vi "ControlProgram5.5.vi"() -> ()   [LabVIEW 2016]
uses:
  <vilib>/Utility/error.llb/DialogType.ctl
  <vilib>/Utility/miscctls.llb/LVPoint32TypeDef.ctl
  <vilib>/DAQmx/write.llb/DAQmx Write (Digital Bool 1Line 1Point).vi
  <vilib>/DAQmx/create/channels.llb/DAQmx Create Channel (DO-Digital Output).vi
  <vilib>/platform/TimedLoop/XDataNode/XDataNode.xnode
  <vilib>/Platform/TimedLoop/XDataNode/nitl_modes.ctl
  <vilib>/Platform/TimedLoop/XDataNode/XDNodeRunTimeDep.lvlib
  <vilib>/Platform/TimedLoop/XDataNode/wakeup.ctl
  <vilib>/Platform/TimedLoop/XDataNode/timing_clust.ctl
  <vilib>/DAQmx/create/channels.llb/DAQmx Create Channel (AI-Voltage-Basic).vi
  <vilib>/DAQmx/create/channels.llb/DAQmx Create Channel (AO-Voltage-Basic).vi
  <vilib>/DAQmx/write.llb/DAQmx Write (Analog 1D DBL NChan 1Samp).vi
  <resource>/objmgr/daqmx.rc
  <vilib>/Analysis/NI_AALBase.lvlib
  <vilib>/Analysis/baseanly.llb/Mean (DBL).vi
  <vilib>/Instr/_visa.llb/VISA Configure Serial Port (Instr).vi
  <vilib>/Utility/inputDevices.llb/closeMouse.vi
  <vilib>/Utility/inputDevices.llb/mouseAcquire.vi
  <vilib>/DAQmx/read.llb/DAQmx Read (Analog 2D DBL NChan NSamp).vi
  <vilib>/DAQmx/configure/timing.llb/DAQmx Timing (Sample Clock).vi
panel:
  in  "Save file index":i32
  out "Flush Sample Start Time":u32=2111292881
  out "Sample flush time (s)":dbl=48.0
  in  "Inject Sample":bool
  out "Chart Freq (Hz)":dbl=500.0
  out "Cal values":T1={"AX alpha"=612.9626061060078, "BX alpha"=549.6584469744151, "AX kappa"=0.3485731373010688, "BX kappa"=0.3853424216291352, "AX offset"=-0.03900484438240665, "BX offset"=-0.11295550662085417, "AY alpha"=582.7562541114835, "BY alpha"=571.1587543790358, "AY kappa"=0.37498408087930674, "BY kappa"=0.36252029651198364, "AY offset"=-0.21125584642206058, "BY offset"=-0.12469077200400738}
  in  "Inject Pump 1":bool
  in  "Inject Pump 2":bool
  in  "Tab Control 2":T2(tab)
  in  "Force FB script":bool
  in  "Got ADig bead":bool
  in  "Move Cap. 2 (ADig Top)":bool
  in  "Dump beads":bool
  in  "Got DNA bead":bool
  in  "Flow on\ncap 2?":bool=TRUE
  in  "Flow on\ncap 1?":bool=TRUE
  in  "Flow on\ndump?":bool=TRUE
  in  "Fish After TA?":bool=TRUE
  in  "Delta after tether":dbl=1600.0
  in  "TA Cancel Save?":bool=TRUE
  in  "Min fish\ndelta (nm)":dbl=1425.0 min=0.0 max=5000.0 step=50.0
  in  "Max fish\ndelta (nm)":dbl=1900.0 min=0.0 max=5000.0 step=25.0
  in  "Fish Speed (ms)":i32=5000
  in  "Wait (ms)":i32=1500
  in  "# attempts":dbl=10.0
  in  "Cutoff force (pN)":dbl=4.5
  in  "Raster after\n tether?":bool=TRUE
  out "Tether":bool
  out "Attempt #":i32
  in  "Flow on\nwhile fish?":bool=TRUE
  in  "Flow on\nafter raster?":bool=TRUE
  in  "Offset @ Delta (nm)":dbl=1600.0
  in  "Cal @ Delta (nm)":dbl=2500.0
  in  "Cal stage position":i32=3
  out "Cal Final Sampling Rate":dbl=125000.0
  in  "Cal Averaging":i32=1
  in  "Wait before dip (s)":dbl=3.0
  in  "Start dipping after?":bool
  in  "Start trap delta (nm)":dbl=1700.0
  in  "Cancel dwell":bool
  in  "Pause dwell":bool
  in  "Return position":dbl=3.0
  in  "Dip duration":dbl=15.0
  in  "Dip position":dbl=4.0
  in  "Dip":bool
  out "Dip time":i32
  in  "Stop":bool=TRUE
  in  "?":T3(tab)=enum."Raster scan"
  in  "Save N sets":bool
  in  "N sets":i32=200
  in  "Cal sets to save":i32=500
  in  "Reset data stream":bool
  out "Buffer Overflow":bool
  out "Stage moving":bool
  in  "Comment":string
  in  "Raster scan":bool
  out "Saving":bool
  in  "Save cal":bool
  in  "Save Data":bool
  in  "Stop saving":bool
  out "Calibrating":bool
  out "Progress":dbl(slide) scale=0.0..100.0
  in  "Read Cal":bool
  in  "Fish":bool
  in  "Averaging Number":i32=1250
  out "Final Sampling Rate":dbl=100.0
  in  "Trap position (V)":cluster{"X":dbl, "Y":dbl}={"X"=4.184262478968032, "Y"=2.3}
  in  "Trap delta (nm)":dbl=2500.0 min=0.0 max=5000.0 step=50.0
  in  "Fixed X":dbl=1.38
  in  "Fixed Y":dbl=2.3
  in  "Shutter 1 (B)":bool=TRUE
  in  "Shutter 2 (A)":bool
  in  "Pulling direction":bool
  out "Raster scanning...":bool
  out "Current file name":path=path "D:/data/160111/160111_006.dat"
  in  "AX alpha":dbl=612.9626061060078 format="%#_3p"
  in  "BX alpha":dbl=549.6584469744151 format="%#_3g"
  in  "AX kappa":dbl=0.3485731373010688 format="%#_3g"
  in  "BX kappa":dbl=0.3853424216291352 format="%#_3g"
  in  "AX offset":dbl=-0.03900484438240665 format="%#_3g"
  in  "BX offset":dbl=-0.11295550662085417 format="%#_3g"
  in  "AY alpha":dbl=582.7562541114835 format="%#_3g"
  in  "BY alpha":dbl=571.1587543790358 format="%#_3g"
  in  "AY kappa":dbl=0.37498408087930674 format="%#_3g"
  in  "BY kappa":dbl=0.36252029651198364 format="%#_3g"
  in  "AY offset":dbl=-0.21125584642206058 format="%#_3g"
  in  "BY offset":dbl=-0.12469077200400738 format="%#_3g"
  out "Buffer status":u8(slide) scale=0.0..100.0
  in  "Set Current\nPos to (0,0,0)":bool
  in  "dump spot":string="Dump beads spot"
  in  "up flow spot":string="Upper flow spot"
  in  "low flow spot":string="Lower flow spot"
  in  "up cap":string="Upper capillary (ADig beads)"
  in  "bottom cap":string="Lower capillary (DNA beads)"
  in  "Move to Position 5":bool
  in  "Set Position 5":bool
  in  "Saved stage positions":dbl[][](array[numeric])=[[1.0, 0.0, 0.0, 0.0], [2.0, -0.13716, -3.21132, 0.01436], [3.0, 0.45, -0.73974, 0.005], [4.0, 0.45, -2.1978, 0.005], [5.0, 0.45, -2.63158, -0.02256]]
  in  "Set Position 2":bool
  in  "Move to Position 2":bool
  in  "Set Position 1":bool
  in  "Move to Position 1":bool
  in  "Set Position 4":bool
  in  "Move to Position 4":bool
  in  "Set Position 3":bool
  in  "Move to Position 3":bool
  out "Stage error":errorcluster
  in  "Clear Volume":bool
  out "Sample Flush Meter":u8(slide) scale=0.0..100.0
  out "Flushing Sample":bool
  in  "Flush Sample":bool
  in  "Normal \nRate (ul/hr)  3":dbl=100.0
  in  "Normal \nVolume (ul) 3":dbl=250.0
  in  "Normal \nVolume (ul) 2":dbl
  in  "Normal \nRate (ul/hr)":dbl
  in  "Normal \nVolume (ul)":dbl
  in  "Flush\nRate (ul/min)":dbl
  in  "Flush\nVolume (ul)":dbl
  in  "Flush \nRate (ul/min)  2":dbl
  in  "Flush Pump 2":bool
  in  "Flush\nVolume (ul)  2":dbl
  in  "Flush Pump 1":bool
  in  "Normal \nRate (ul/hr)  2":dbl
  in  "Write Wait":i32=1000
  in  "Flush \nRate (ul/min)  3":dbl=100.0
  in  "Flush\nVolume (ul)  3":dbl=80.0
  out "error out":errorcluster
  in  "Use Mouse to Move Trap?":bool
  in  "Pause Mouse/Mirror Connection":bool
  out "Reference Voltage":cluster{dbl, dbl}={0.0, -0.0}
  out "Saved voltage":cluster{dbl, dbl}={5.766666666666665, 1.45}
  out "Real Coordinates":cluster{"Horizontal":i32, "Vertical":i32}={"Horizontal"=897, "Vertical"=-1271}
  out "CoordinatesMousePressed":T4
  out "Sum error":dbl(knob) scale=-0.1..0.1
  out "Trap sep":waveform(dbl)[](graph)=[{"t0"=timestamp(254.52999999991349 s since 1904-01-01), "dt"=0.002, "Y"=[2500.401353709495, 2500.7138927997967, 2500.64380131258, 2500.593243518474, 2500.684017739553], "attributes"=variant("NI_ChannelName"=variant(string "T2 X"))}, {"t0"=timestamp(254.52999999991349 s since 1904-01-01), "dt"=0.002, "Y"=[2.3273345839872768, 2.356012897788485, 2.38273587208189, 2.3403701811713593, 2.3442808603313674], "attributes"=variant("NI_ChannelName"=variant(string "T2 Y"))}]
  in  "Set reading to\nsetpoint":bool
  in  "Offset Y (nm)":dbl format="%0.2f"
  in  "Offset X (nm)":dbl format="%0.2f"
  in  "Remove offsets":bool
  in  "Force Feedback":bool
  out "Feedback Output Voltage 2":cluster{dbl, dbl} {"?" format="%#_4g"; "?" format="%#_4g"}
  in  "Offset":cluster{"Off Y":dbl, "Off X":dbl}={"Off Y"=1.5, "Off X"=0.17}
  in  "Setpoint voltage":cluster{"SP Y":dbl, "SP X":dbl}={"SP Y"=0.6, "SP X"=0.0}
  in  "Feedback const":T5={"Ki_B_Y"=0.5, "Ki_B_X"=0.0, "Kp Y"=1.0, "Kp X"=0.0}
  out "Mean Trap Pos X 2 (nm)":dbl=2500.6072618159797 format="%0.2f"
  out "Mean Trp Pos Y 2 (nm)":dbl=2.3501468790720756 format="%0.2f"
  out "T2 X RMS (A)":dbl=1.1062679088370557 format="%0.2f"
  out "T2 Y RMS (A)":dbl=0.1869142822643123 format="%0.2f"
  in  "Scan range (nm)":dbl=425.0
  in  "Scan speed (nm/s)":dbl=100.0 min=0.0 max=100.0
  in  "Step size (nm)":dbl=1.0
  in  "Save scans":bool=TRUE
  in  "# scans":i32=1
  in  "Load param":bool
  in  "Scan Parameters":T6(array[cluster])=[{"Label"="Offset", "Max delta 2"=3.8, "Start delta 2"=2.4, "Speed (ms) 2"=10000, "# scans 2"=1}]
  in  "Trap delta\nafter (nm)":dbl=1750.0
  in  "Stop raster":bool
  out "Scan range (V)":dbl=0.47672462142456534
  out "Scan steps (mirror)":u64=425
  out "Scan increment (V)":dbl=0.0011217049915872126
  out "Time per step (ms)":dbl=10.0
  out "Total raster time (s)":dbl=8.5
  out "N sets to be saved":dbl=850.0
  out "Continue to display?":bool
  out "Video Error":errorcluster
  in  "# Samples/channel (in)":i32=40000 format="%.2f"
  out "Buffer size\n(Samples/channel)":u32=511
  out "DAQ rate\n(Samples/s)":dbl=125000.0 format="%#_6p"
  out "# Samples/channel":i32=1250
  out "# Samples/channel/s":dbl=100.0
  out "AvailSampPerChan":u32=9
  out "Data update period (s/set)":dbl=0.01 format="%#_6p"
  out "AvailSampPerChan 2":u32=110
  in  "PC samp per channel":i32=1000
  in  "Sampling Rate":dbl=125000.0 format="%0.0p"
  in  "DAQ Rate2":dbl=1000000.0 format="%#_6p"
  out "Data period (s)":dbl=8e-06 format="%#_6p"
  in  "Tether break\nforce (pN)":dbl=1.0
  in  "Path":path=path "D:/data"
  out "Mirror task":refnum<k21>
  in  "Conv X (nm/V)":dbl=891.5
  in  "Conv Y (nm/V)":dbl=505.7
  in  "Min value Y":dbl format="%.1g"
  in  "Max value Y":dbl=10.0 format="%.1f"
  in  "Min value X":dbl format="%0.1f"
  in  "Max value X":dbl=10.0 format="%.1f"
  in  "HWP1":string="Half waveplate 1: differential trap power"
  in  "HWP0":string="Half waveplate 0: total trap power"
  in  "Move 1":bool
  in  "\"Degrees\" 1":dbl
  in  "Move 0":bool
  in  "\"Degrees\" 0":dbl
  out "Chamber":T7(plugin-control)
  out "Deflection":T4
  in  "Sampling Rate":dbl=125000.0 format="%0.2f"
  in  "Averaging Number":i32=12500
  in  "DAQ Rate":dbl=1000000.0
  out "Final Sampling Rate":dbl
  in  "Tab Control":T8(tab)
  in  "Downsamp\nfact":dbl=250.0
  out "Bead sep":waveform(dbl)[](graph)=[{"t0"=timestamp(254.52999999991349 s since 1904-01-01), "dt"=0.002, "Y"=[213.39995113031458, 213.93706235351536, 212.9933488170291, 212.83435664066477, 214.2058422181686], "attributes"=variant("NI_ChannelName"=variant(string "T2"))}, {"t0"=timestamp(254.52999999991349 s since 1904-01-01), "dt"=0.002, "Y"=[5.143660273474187, 5.894059413878943, 4.88588887583271, 5.354302143675658, 5.8339035430258015], "attributes"=variant("NI_ChannelName"=variant(string "T1"))}]
  out "Force (pN)":waveform(dbl)[](graph)=[{"t0"=timestamp(254.52999999991349 s since 1904-01-01), "dt"=0.002, "Y"=[77.86854854855086, 78.08600694234892, 77.6994254352176, 77.66772581948469, 78.22322365982815], "attributes"=variant("NI_ChannelName"=variant(string "T2"))}, {"t0"=timestamp(254.52999999991349 s since 1904-01-01), "dt"=0.002, "Y"=[1.9758532189955713, 2.255599507656321, 1.8769321413323554, 2.045475885196074, 2.2199437572021146], "attributes"=variant("NI_ChannelName"=variant(string "T1"))}]
  out "Mean force (pN)":dbl=39.991873491581266 format="%0.2f"
  out "Force noise (pN)":dbl=0.17287401460430454 format="%0.2f"
  out "Mean Bead Sep\n(nm)":dbl=109.44823754095798 format="%0.2f"
  out "Bead Sep Noise\n(A)":dbl=4.382305822805036 format="%0.2f"
  out "PSD 2":cluster{dbl[], dbl[]}(graph)
  out "PSD 1":cluster{dbl[], dbl[]}(graph)
  out "PSD 1 Sum":dbl(slide) scale=0.0..10.0
  out "PSD 2 Sum":dbl(slide) scale=0.0..10.0
  in  "Start":bool
  out "All signals":waveform(dbl)[](graph)=[{"t0"=timestamp(254.52999999991349 s since 1904-01-01), "dt"=0.002, "Y"=[-0.015598133099047685, -0.01565794312346797, -0.015569001492569037, -0.015625202290861444, -0.015752814195447103], "attributes"=variant("NI_ChannelName"=variant(string "A y"))}, {"t0"=timestamp(254.52999999991349 s since 1904-01-01), "dt"=0.002, "Y"=[-0.008051314077172257, -0.008039455196512668, -0.008078641062942567, -0.008046931447407441, -0.00800258954569925], "attributes"=variant("NI_ChannelName"=variant(string "A x"))}, {"t0"=timestamp(254.52999999991349 s since 1904-01-01), "dt"=0.002, "Y"=[-0.8186799727186506, -0.828518168587136, -0.8182847428509795, -0.8289376238127658, -0.8367167087325929], "attributes"=variant("NI_ChannelName"=variant(string "B y"))}, {"t0"=timestamp(254.52999999991349 s since 1904-01-01), "dt"=0.002, "Y"=[-0.7880865286255396, -0.794686015346124, -0.785544853888779, -0.7877818022288781, -0.7909004423629264], "attributes"=variant("NI_ChannelName"=variant(string "B x"))}, {"t0"=timestamp(254.52999999991349 s since 1904-01-01), "dt"=0.002, "Y"=[0.031377424462748806, 0.03139546842223122, 0.03140835696460643, 0.03146506655133351, 0.031459911134330096], "attributes"=variant("NI_ChannelName"=variant(string "A sum"))}, {"t0"=timestamp(254.52999999991349 s since 1904-01-01), "dt"=0.002, "Y"=[6.456821009406946, 6.459892496810089, 6.459914408291232, 6.460361662568834, 6.464131742766271], "attributes"=variant("NI_ChannelName"=variant(string "B sum"))}, {"t0"=timestamp(254.52999999991349 s since 1904-01-01), "dt"=0.002, "Y"=[4.184712679427364, 4.185063256085021, 4.184984634113943, 4.18492792318393, 4.185029745080822], "attributes"=variant("NI_ChannelName"=variant(string "Trap x"))}, {"t0"=timestamp(254.52999999991349 s since 1904-01-01), "dt"=0.002, "Y"=[2.3046022040418968, 2.3046589141739933, 2.3047117577063116, 2.3046279813746713, 2.304635714574513], "attributes"=variant("NI_ChannelName"=variant(string "Trap y"))}]
  # "Bead Calibration"
  # "Y"
  # "X"
  # "Pump #1 Controls"
  # "Pump #2 Controls"
  # "Sample Pump Controls"
  # "Retract the pumps manually. Change it back to INFUSE when you're done. Suck it up, don't whine."
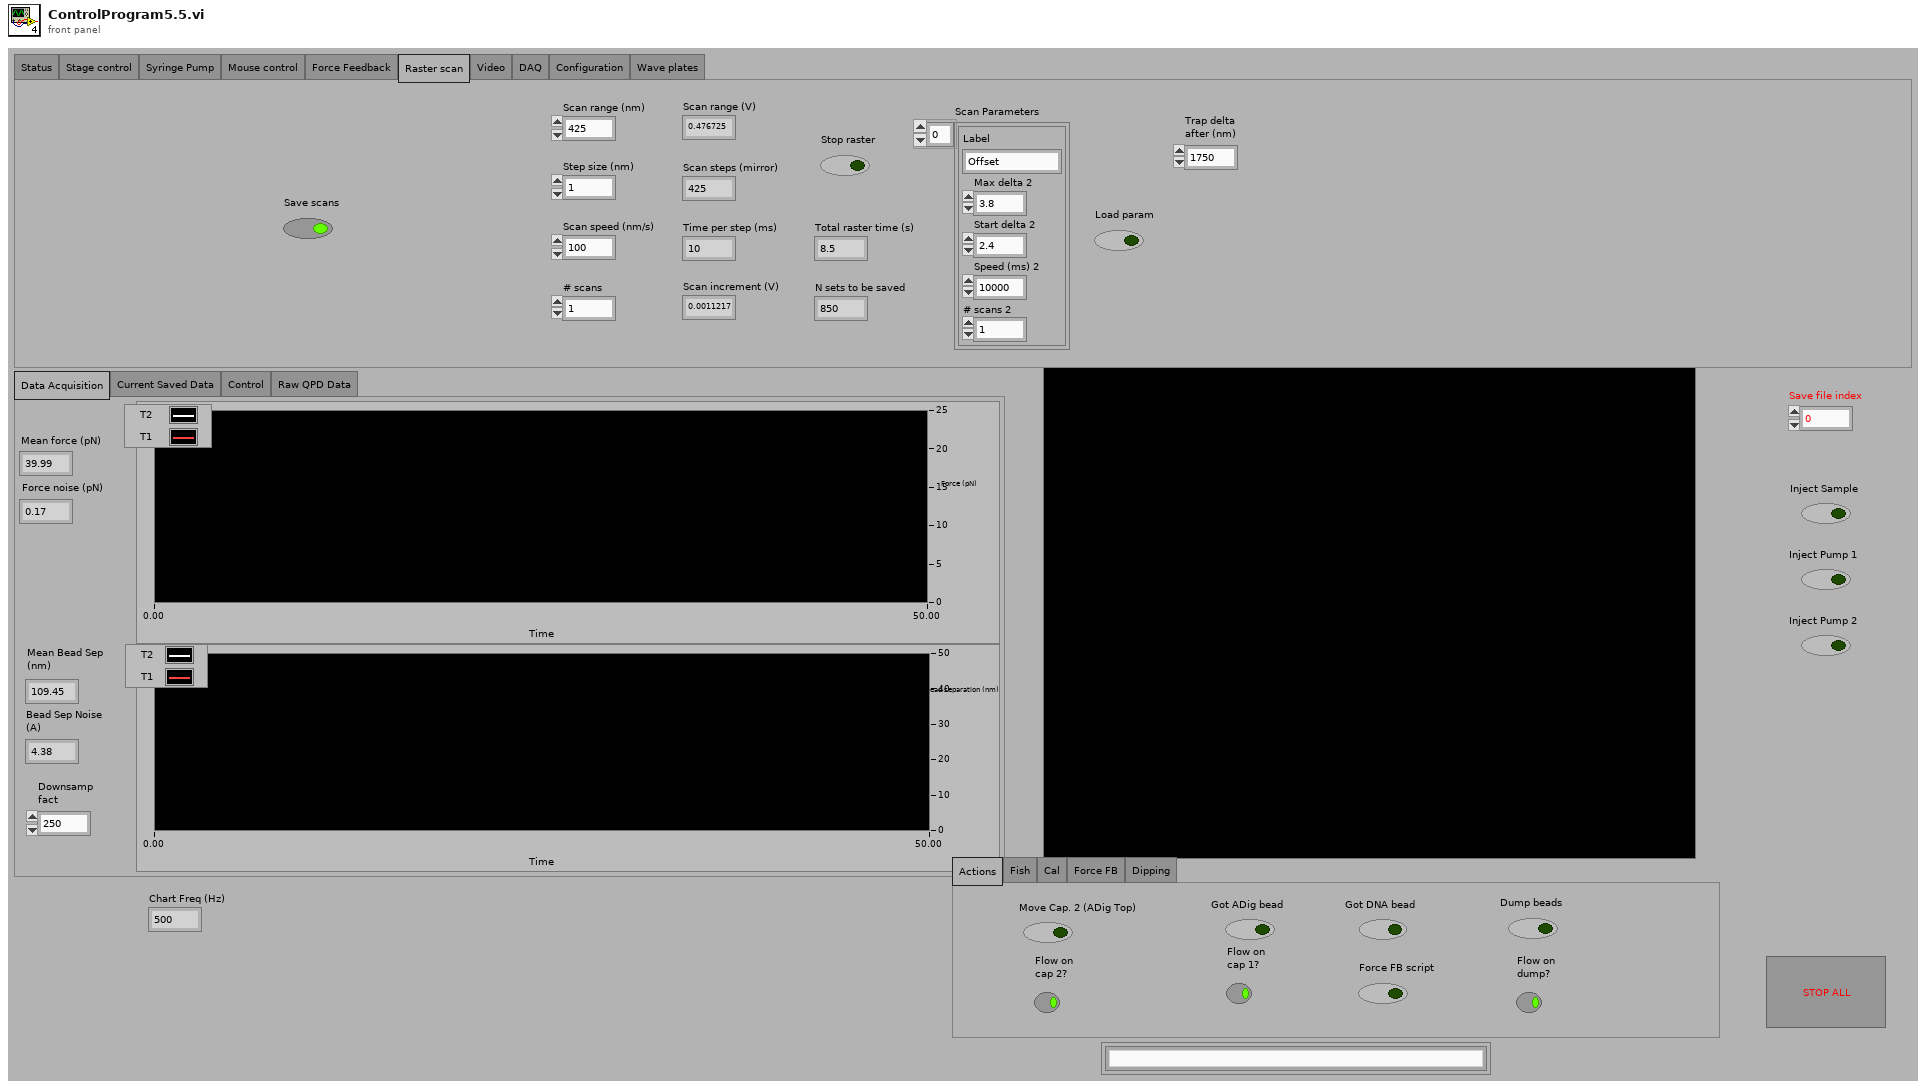
[diagram p1: front panel]
types:
  T1 = cluster{"AX alpha":dbl, "BX alpha":dbl, "AX kappa":dbl, "BX kappa":dbl, "AX offset":dbl, "BX offset":dbl, "AY alpha":dbl, "BY alpha":dbl, "AY kappa":dbl, "BY kappa":dbl, "AY offset":dbl, "BY offset":dbl}
  T2 = enum32{"Actions", "Fish", "Cal", "Force FB", "Dipping"}
  T3 = enum32{"Status", "Stage control", "Syringe Pump", "Mouse control", "Force Feedback", "Raster scan", "Video", "DAQ", "Configuration", "Wave plates"}
  T4 = typedef "LVPoint32TypeDef.ctl" = cluster{"Horizontal":i32, "Vertical":i32}
  T5 = cluster{"Ki_B_Y":dbl, "Ki_B_X":dbl, "Kp Y":dbl, "Kp X":dbl}
  T6 = cluster{"Label":string, "Max delta 2":dbl, "Start delta 2":dbl, "Speed (ms) 2":i32, "# scans 2":i32}[]
  T7 = typedef "IMAQ Image.ctl" = refnum<image>
  T8 = enum32{"Data Acquisition", "Current Saved Data", "Control", "Raw QPD Data"}
  T9 = enum16{"open", "replace", "create", "open or create", "replace or create", "replace or create with confirmation"}
  T10 = enum16{"big-endian, network order", "native, host order", "little-endian"}
  T11 = cluster{string, string, string, string, string, string, string, string}
  T12 = typedef "XDNodeRunTimeDep.lvlib/timing_clust.ctl" = cluster{"Expected End [f-1]":u64, "Actual End [f-1]":u64, "Finished Late? [f-1]":bool, "Expected End [i-1]":u64, "Actual End [i-1]":u64, "Finished Late? [i-1]":bool, "Expected Start [i]":u64, "Actual Start [i]":u64, "Expected Start [f]":u64, "Actual Start [f]":u64, "Source Name":string, "Structure Name":string, "Period":i64, "Deadline":i64, "Offset":i64, "Start":i64, "Priority":i32, "Timeout":i32, "Mode":T13, "Wakeup Reason":T14, "Error":errorcluster, "Source Type":string, "Secondary Source Type":string, "Global End Time":u64, "Global Start Time":u64, "Frame Duration":u64, "Iteration Duration":u64, "Assigned CPU":i32, "I/O Scan Engine Mode":u32}
  T13 = typedef "XDNodeRunTimeDep.lvlib/nitl_modes.ctl" = enum32{"No Change", "Process missed periods, maintain original phase", "Discard missed periods, maintain original phase", "Process missed periods, ignore original phase", "Discard missed periods, ignore original phase"}
  T14 = typedef "XDNodeRunTimeDep.lvlib/wakeup.ctl" = enum32{"Normal", "Aborted", "Asynchronous wakeup", "Timing source error", "Timed loop error", "Timeout"}
  T15 = typedef "DialogType.ctl" = u16
  T16 = cluster{"button 1":bool, "button 2":bool, "button 3":bool, "button 4":bool}
  T17 = cluster{"[0]":dbl, "[1]":dbl, "[2]":dbl, "[3]":dbl, "[4]":dbl, "[5]":dbl, "[6]":dbl, "[7]":dbl, "[8]":dbl, "[9]":dbl, "[10]":dbl, "[11]":dbl}
  T18 = cluster{"Label":string, "Max delta 2":dbl, "Start delta 2":dbl, "Speed (ms) 2":i32, "# scans 2":i32}
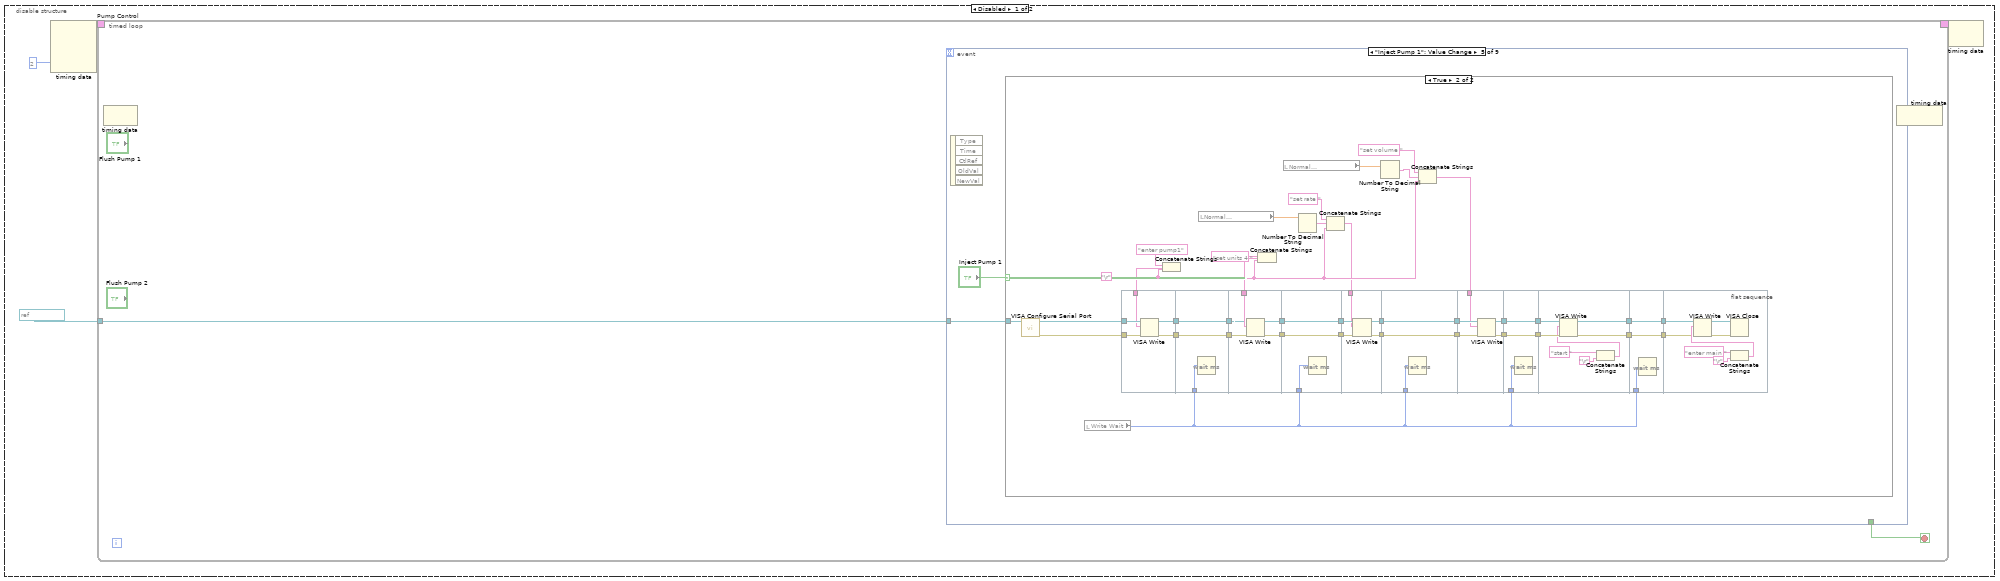
[diagram p2: hidden frame]
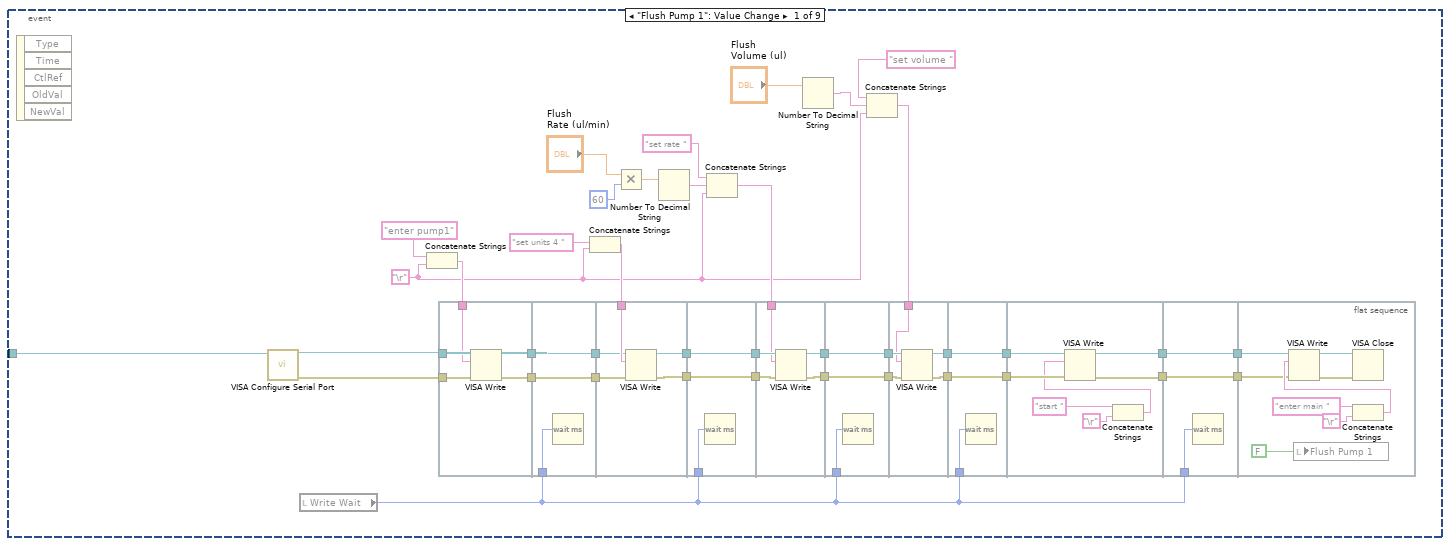
[diagram p3: hidden frame]
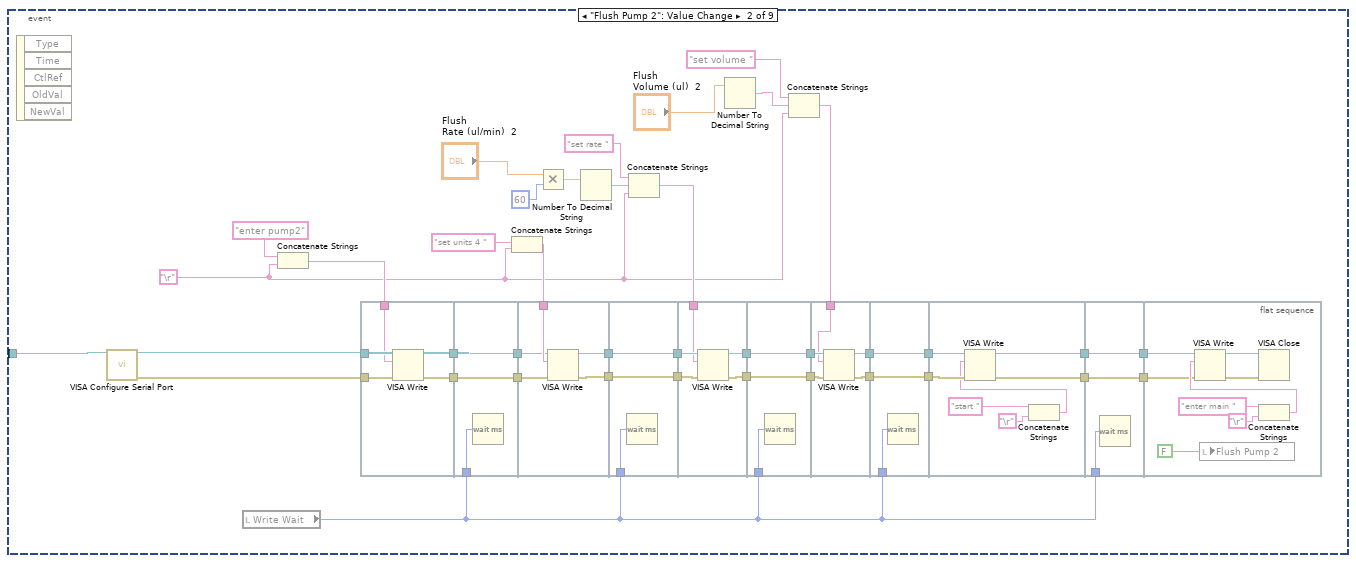
[diagram p4: hidden frame]
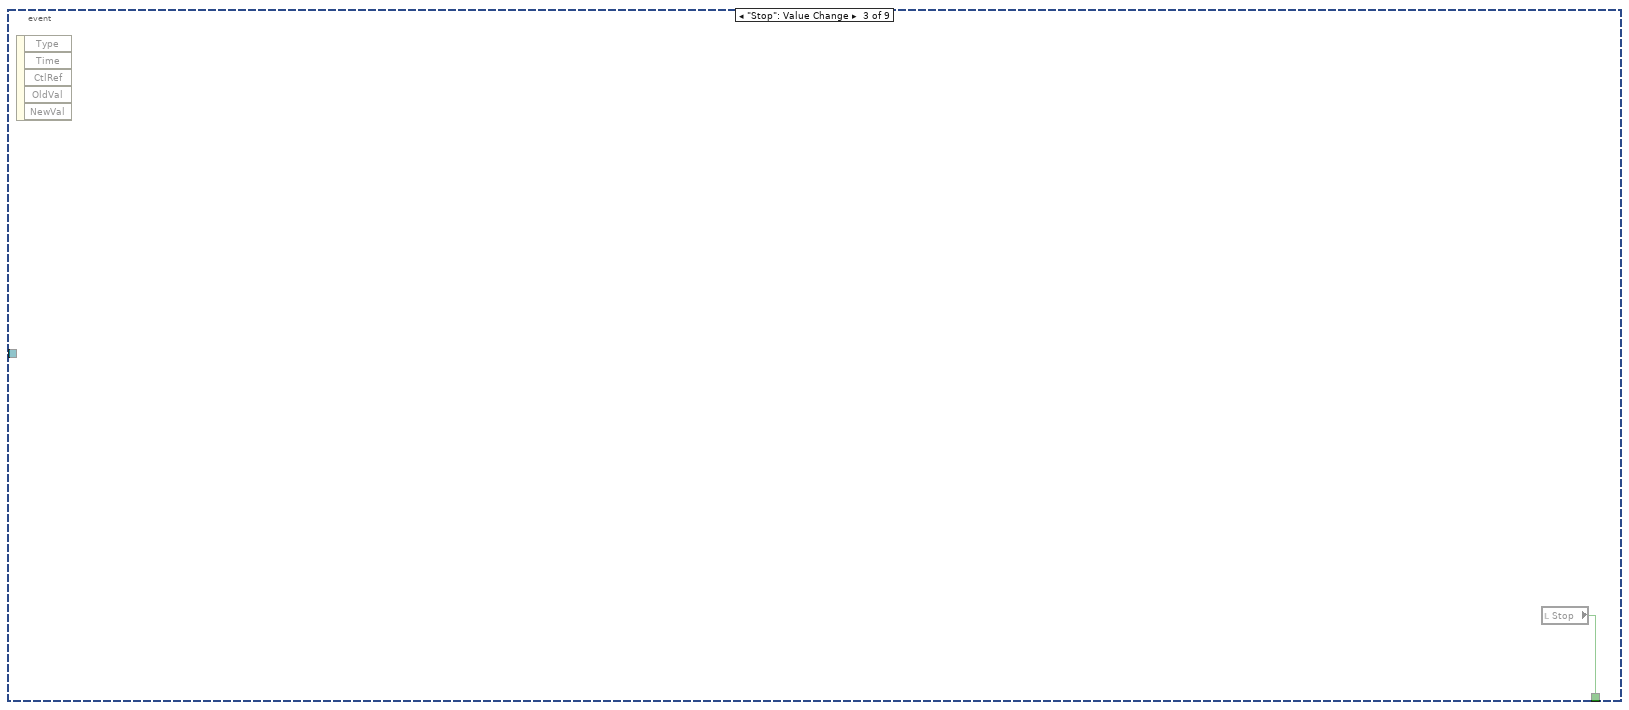
[diagram p5: hidden frame]
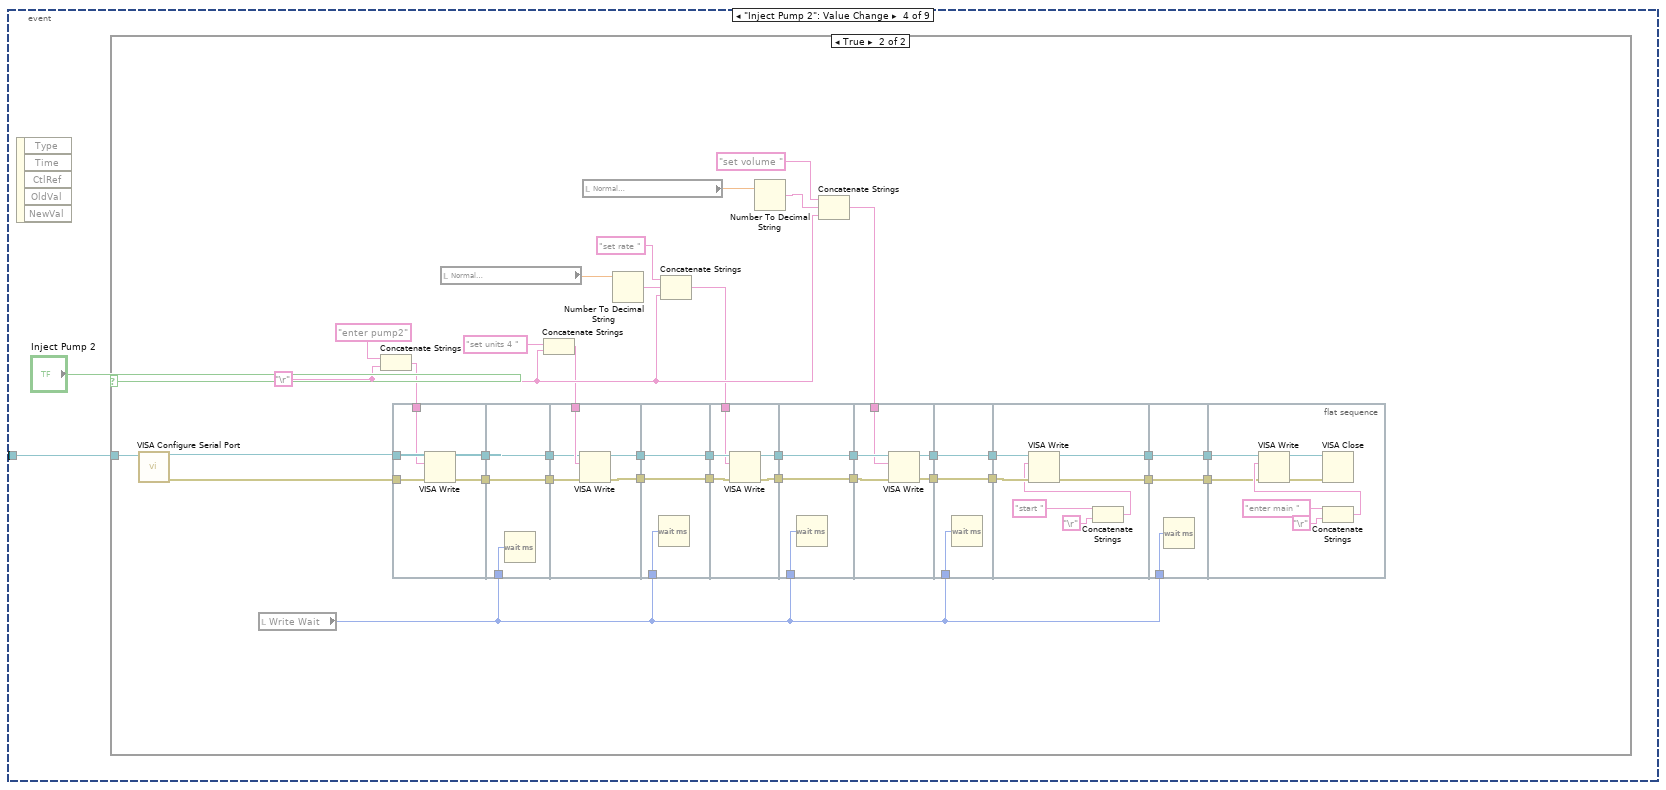
[diagram p6: hidden frame]
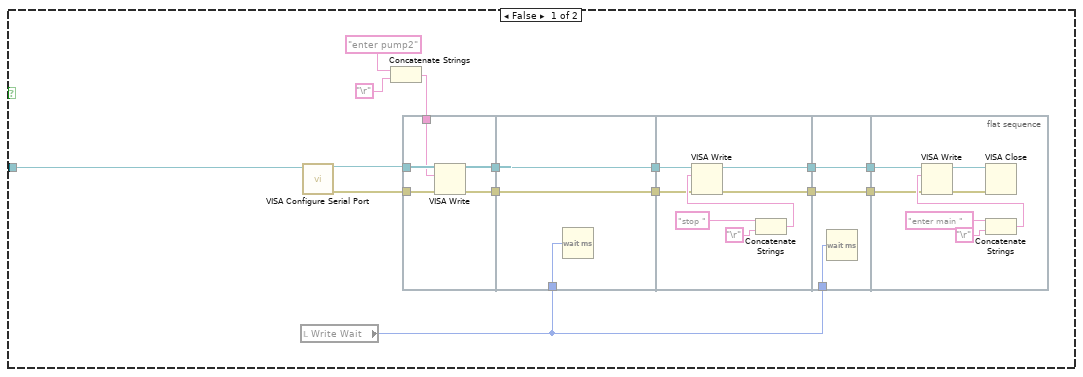
[diagram p7: hidden frame]
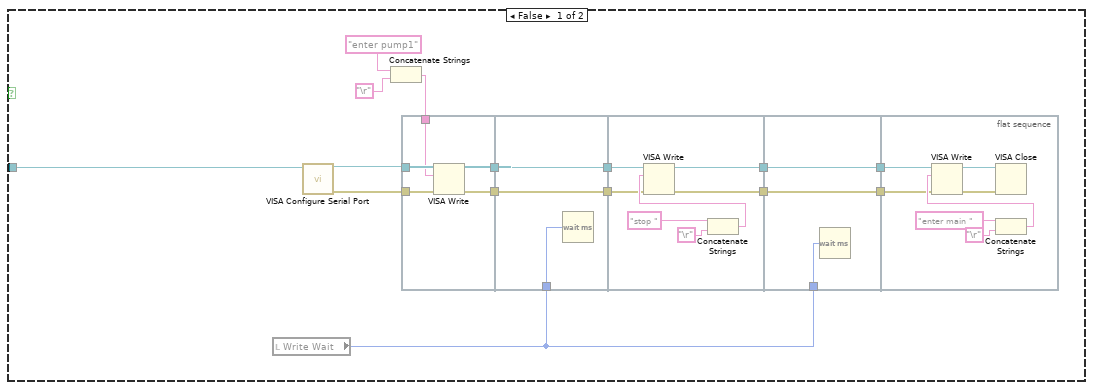
[diagram p8: hidden frame]
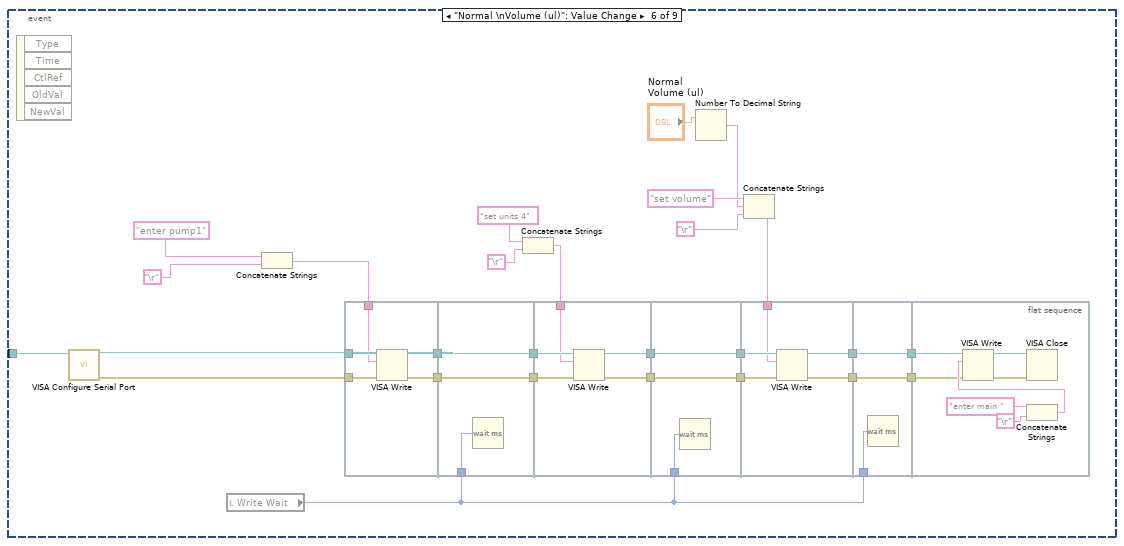
[diagram p9: hidden frame]
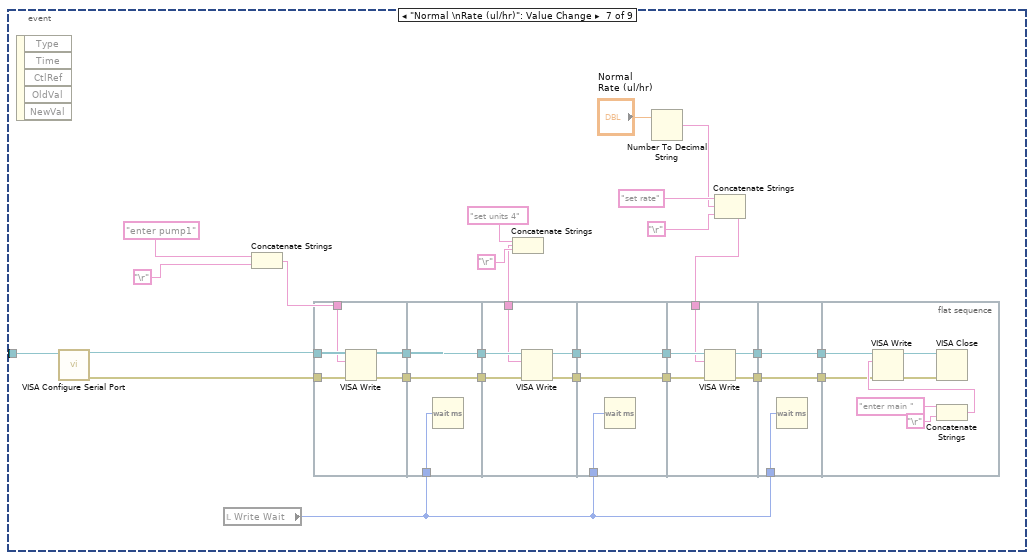
[diagram p10: hidden frame]
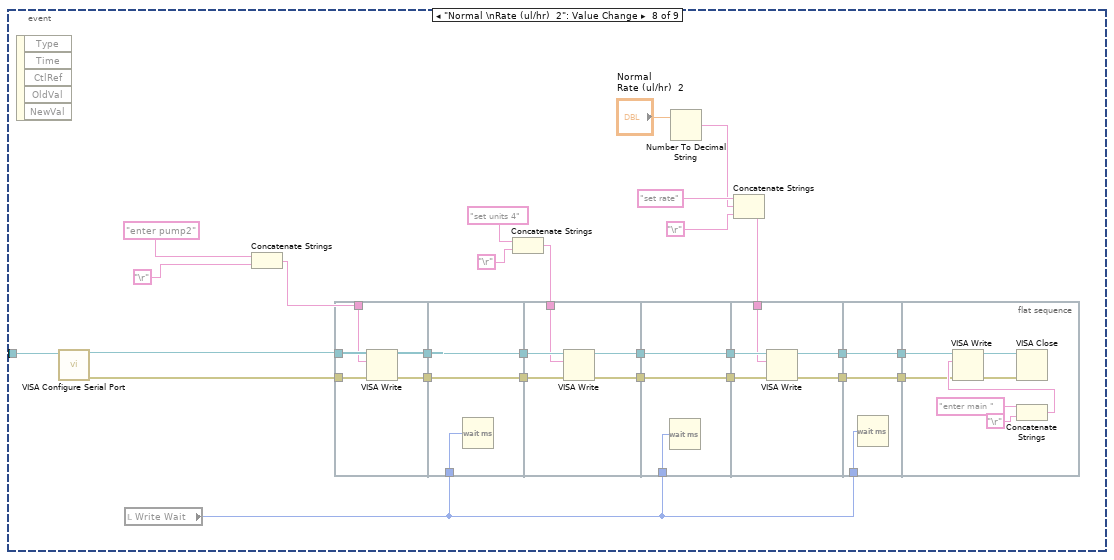
[diagram p11: hidden frame]
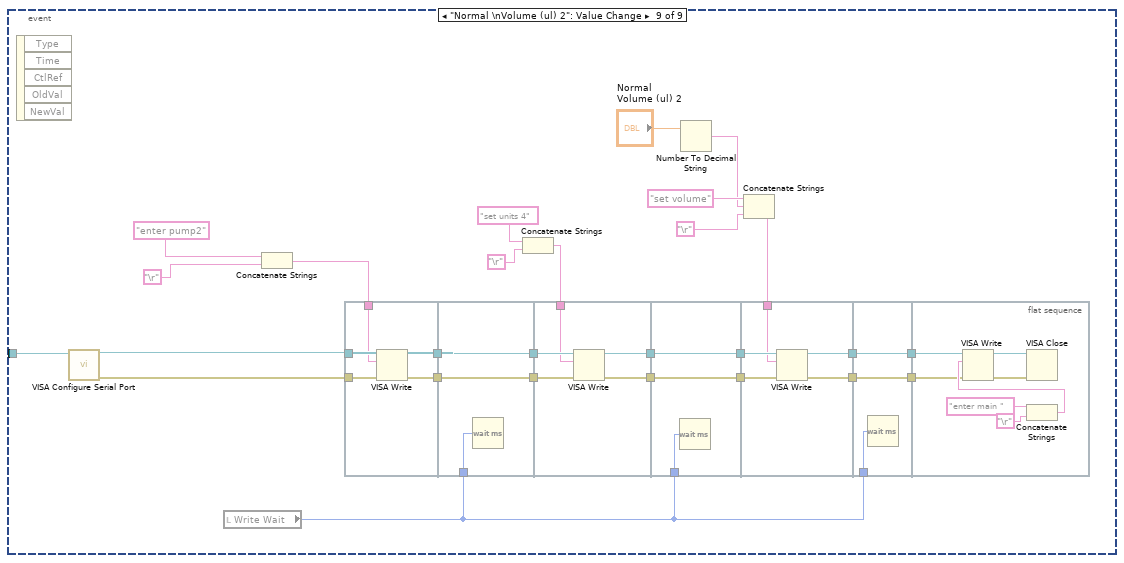
[diagram p12: hidden frame]
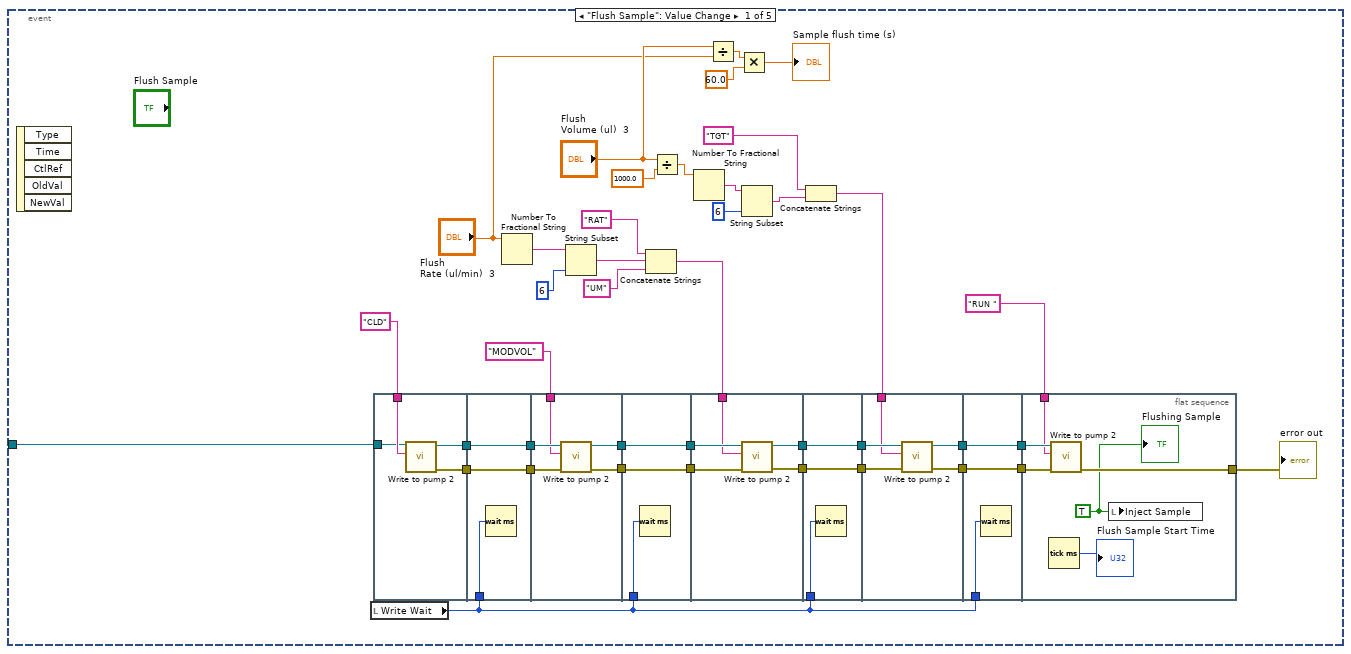
[diagram p13: hidden frame]
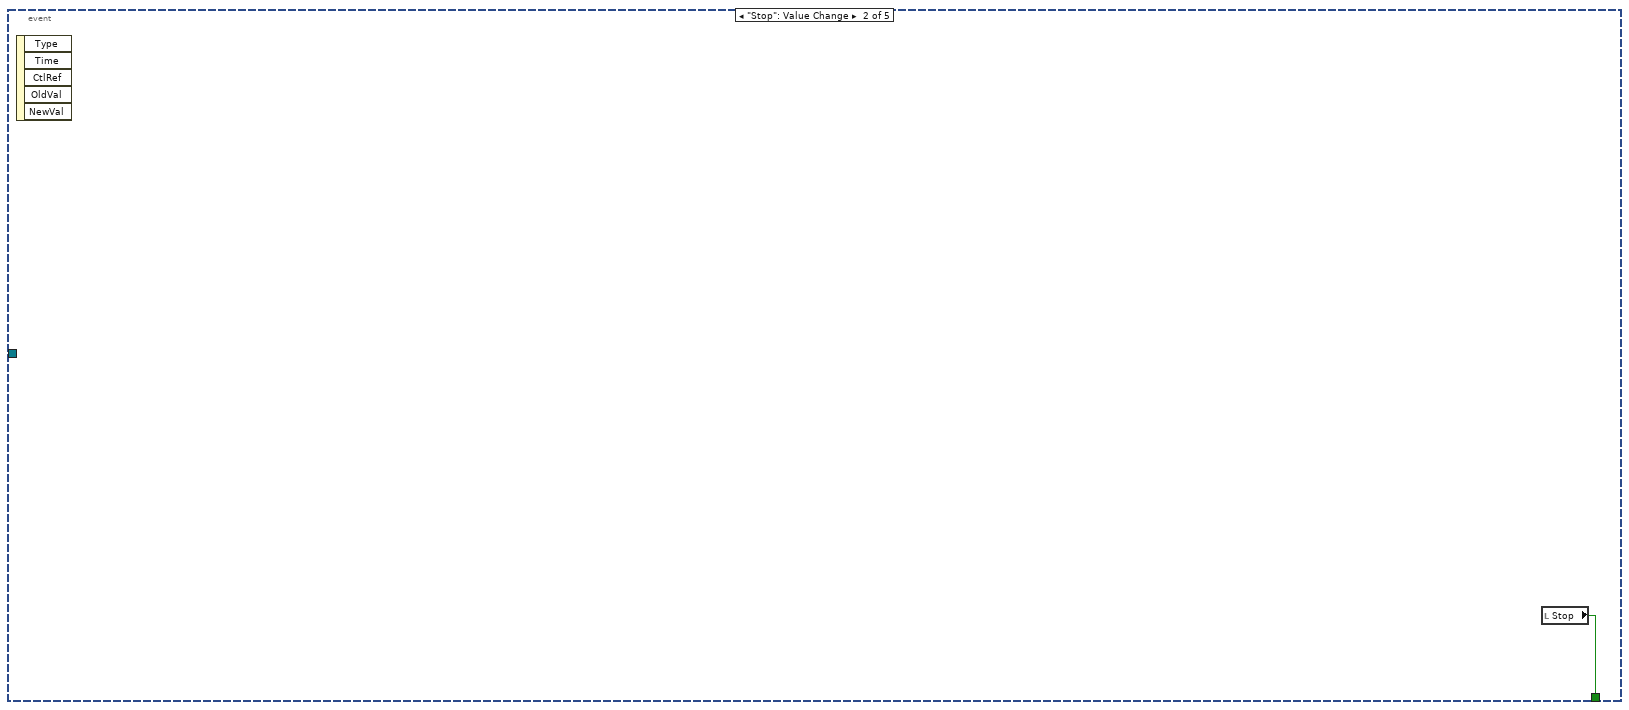
[diagram p14: hidden frame]
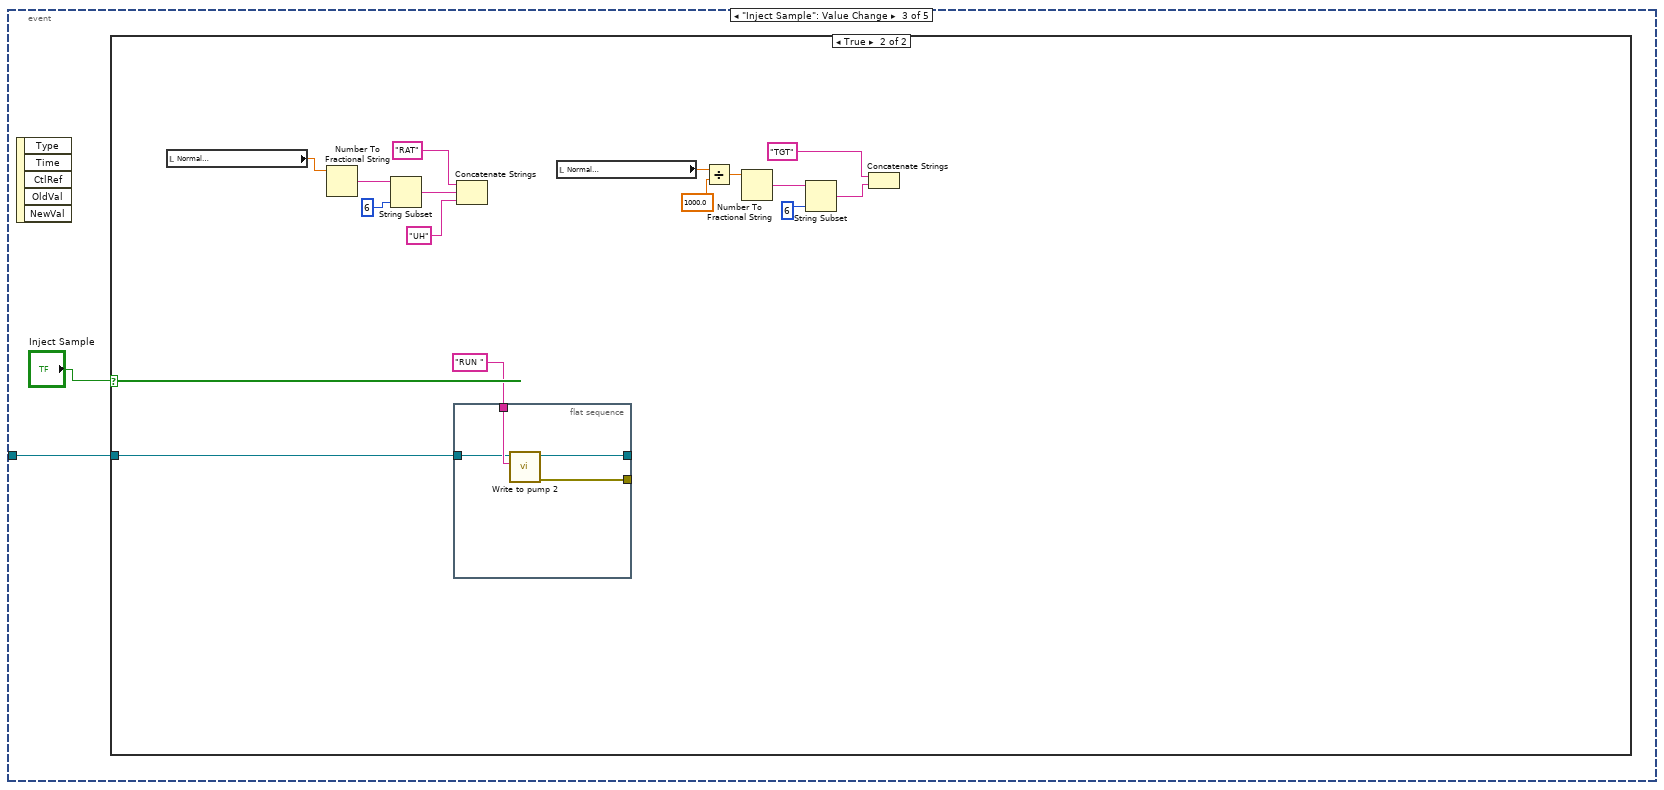
[diagram p15: hidden frame]
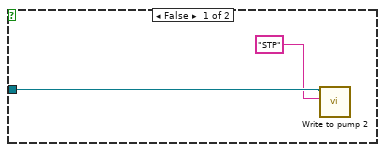
[diagram p16: hidden frame]
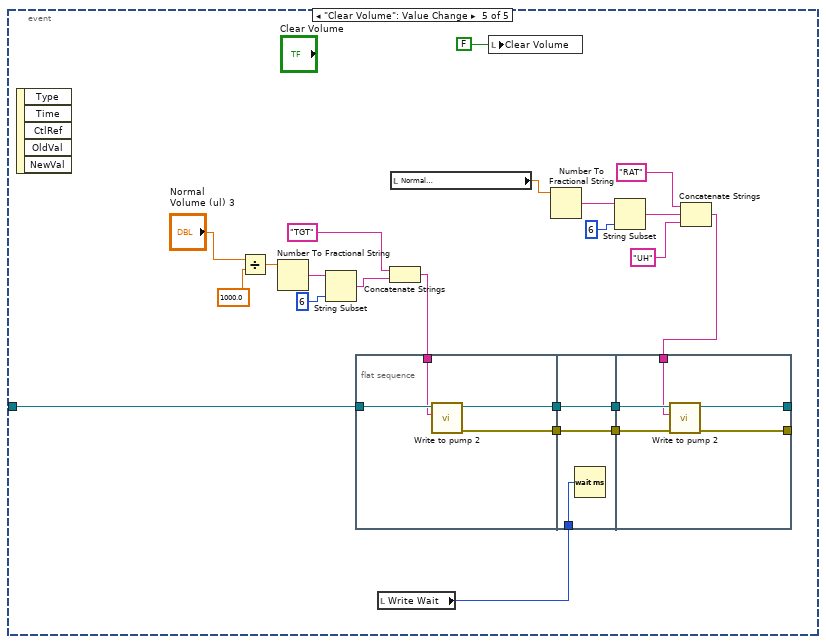
[diagram p17: hidden frame]
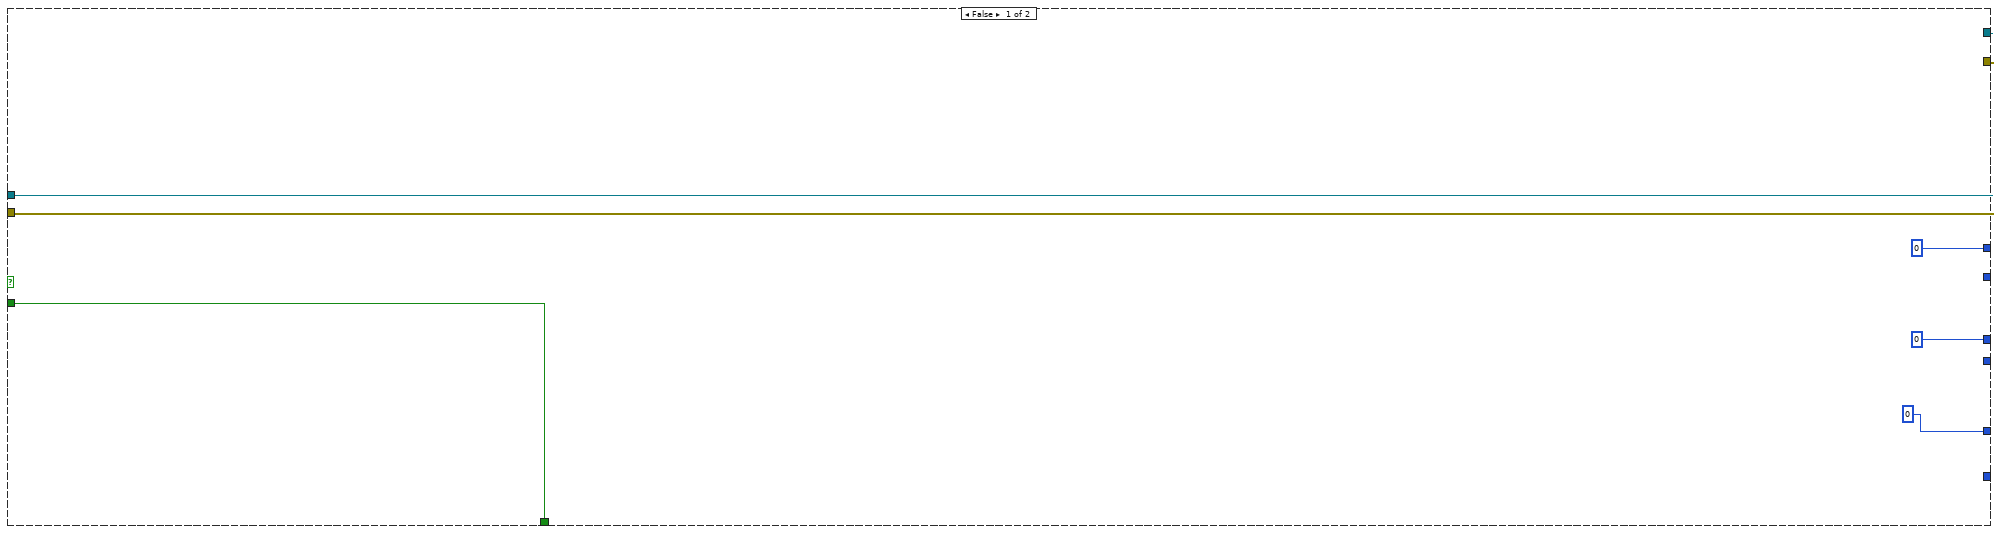
[diagram p20: hidden frame]
diagram:
  w42 = 10.0 ("Minimum Value")
  w43 = -10.0 ("Minimum Value")
  w45 = -2.0 ("Minimum Value")
  w46 = 2.0 ("Maximum Value")
  w71 = 10123 items=["Finite Samples"=10178, "Continuous Samples"=10123] ("sample mode")
  w92 = tag "Dev1/port2/line1"  # Shutter 2
  w95 = tag "Dev1/port1/line4"  # Shutter 1
  # "Create channels for movable mirror"
  # "Create channels for detectors"
  n1 = call-poly <vilib>:"DAQmx Create Virtual Channel.vi"("maximum value"=w46, "minimum value"=w45, "physical channels"=tag "Dev1/ai0" ("Physical Channel")) -> ("task out"=w47:refnum<k21>, "error out"=w70:errorcluster)  [unwired: 11 in]
  n2 = call-poly <vilib>:"DAQmx Create Virtual Channel.vi"("task in"=w47, "maximum value"=w46, "minimum value"=w45, "physical channels"=tag "Dev1/ai1", "error in"=w70) -> ("task out"=w68:refnum<k21>, "error out"=w67:errorcluster)  [unwired: 9 in]
  n3 = call-poly <vilib>:"DAQmx Create Virtual Channel.vi"("task in"=w68, "maximum value"=w46, "minimum value"=w45, "physical channels"=tag "Dev1/ai2", "error in"=w67) -> ("task out"=w59:refnum<k21>, "error out"=w58:errorcluster)  [unwired: 9 in]
  n4 = call-poly <vilib>:"DAQmx Create Virtual Channel.vi"("task in"=w59, "maximum value"=w46, "minimum value"=w45, "physical channels"=tag "Dev1/ai3" ("Physical Channel"), "error in"=w58) -> ("task out"=w44:refnum<k21>, "error out"=w64:errorcluster)  [unwired: 9 in]
  n5 = call-poly <vilib>:"DAQmx Create Virtual Channel.vi"("task in"=w44, "maximum value"=w42, "minimum value"=w43, "physical channels"=tag "Dev1/ai4", "error in"=w64) -> ("task out"=w62:refnum<k21>, "error out"=w61:errorcluster)  [unwired: 9 in]
  n6 = call-poly <vilib>:"DAQmx Create Virtual Channel.vi"("task in"=w62, "maximum value"=w42, "minimum value"=w43, "physical channels"=tag "Dev1/ai5", "error in"=w61) -> ("task out"=w57:refnum<k21>, "error out"=w56:errorcluster)  [unwired: 9 in]
  n7 = call-poly <vilib>:"DAQmx Create Virtual Channel.vi"("task in"=w57, "maximum value"=w42, "minimum value"=w43, "physical channels"=tag "Dev1/ai6", "error in"=w56) -> ("task out"=w51:refnum<k21>, "error out"=w49:errorcluster)  [unwired: 9 in]
  n8 = call-poly <vilib>:"DAQmx Create Virtual Channel.vi"("task in"=w51, "maximum value"=w42, "minimum value"=w43, "physical channels"=tag "Dev1/ai7", "error in"=w49) -> ("task out"=w50:refnum<k21>, "error out"=w48:errorcluster)  [unwired: 9 in]
  n9 = call-poly <vilib>:"DAQmx Timing.vi"("task/channels in"=w50, "sample mode"=w71, "samples per channel"="PC samp per channel", "rate"="Sampling Rate", "error in"=w48) -> ("task out"=w54:refnum<k21>, "error out"=w53:errorcluster)  [unwired: 9 in]
  n10 = call-poly <vilib>:"DAQmx Create Virtual Channel.vi"("maximum value"="Max value Y", "minimum value"="Min value Y", "physical channels"=tag "Dev1/ao1" ("Trap X Axis")) -> ("task out"=w39:refnum<k21>, "error out"=w41:errorcluster)  [unwired: 11 in]
  n11 = property class="DAQmx Timing"(reference=w54, error in=w53, "More:AI Convert:Rate"="DAQ Rate2") -> (reference out=w6:refnum<k21>, error out=w5:errorcluster, "SampClk.Rate"=→"DAQ rate\n(Samples/s)":dbl)
  n12 = call-poly <vilib>:"DAQmx Create Virtual Channel.vi"("task in"=w39, "maximum value"="Max value X", "minimum value"="Min value X", "physical channels"=tag "Dev1/ao0" ("Trap Y Axis"), "error in"=w41) -> ("task out"=w30:refnum<k21>, "error out"=w29:errorcluster)  [unwired: 9 in]
  "Mirror task" <- w30
  n13 = property class="DAQmx Buffer"(reference=w6, error in=w5) -> (reference out=w3:refnum<k21>, error out=w2:errorcluster, "Input.OnbrdBufSize"=→"Buffer size\n(Samples/channel)":u32)
  n14 = call <vilib>:"DAQmx Start Task.vi"("task/channels in"=w3, "error in"=w2) -> ("task out"=w31:refnum<k21>)  [unwired: 12 in, 1 out]
  n15 = while {
    tunnel: [w126] -> w77
    tunnel: [w318] -> w78
    tunnel: [w124] -> w76
    tunnel: [w430] -> w73
    tunnel: w31 -> [w111]
    tunnel: w30 -> [w426]
    tunnel: w29 -> [w431]
    stop <- w430 stop-if-true
    w167 = "NI_ChannelName" ("name")
    w243 = -1
    # "Scan # counter"
    # "DAQ loop iteration\ncounter (for timing)"
    # "Step counter"
    # "Force feedback"
    # "Raster scan"
    # "Rewire everything"
    # "Invert these because changed\nfrom PSD to QPD"
    # "Trap Y"
    # "Trap X"
    # "Convert to\npN"
    # "Convert to\nnm"
    # "Subtract\noffset"
    # "Normalize by\nsum"
    # "B sum"
    # "BX"
    # "BY"
    # "AX"
    # "AY"
    # "A sum"
    # "Close files when done saving"
    n16 = disable-structure shown="Disabled" {
      frame Disabled {
        n17 = property class="DAQmx Read"() -> ("AvailSampPerChan"=→"AvailSampPerChan 2":u32)  [unwired: 2 in, 2 out]
      }
      frame Enabled {
      }
    }
    n18 = local read "Averaging Number"() -> (w134:i32)
    n19 = local read "Averaging Number"() -> (w137:i32)
    "# Samples/channel" <- w137
    n20 = local read "Sampling Rate"() -> (w429:dbl)
    n21 = call-poly <vilib>:"DAQmx Read.vi"("task/channels in"=w111, "number of samples per channel"=w134, "timeout"=10.0) -> ("task out"=w110:refnum<k21>, "data"=w135:dbl[][], "error out"=w246:errorcluster)  [unwired: 10 in]
    n22 = Unbundle By Name(w246) -> ("status"=w366:bool)
    n23 = Divide(x=w429, y="Cal Averaging") -> (x/y=→"Cal Final Sampling Rate":dbl)
    n24 = Divide(x=w429, y=w137) -> (x/y=→"Final Sampling Rate" →"# Samples/channel/s":dbl)
    n25 = disable-structure shown="Disabled" {
      frame Disabled {
        n26 = local read "Buffer size\n(Samples/channel)"() -> (w433:u32)
        n27 = property class="DAQmx Read"() -> ("AvailSampPerChan"=w434:u32)  [unwired: 2 in, 2 out]
        "AvailSampPerChan" <- w434
        n28 = Divide(x=w434, y=w433) -> (x/y=→"Buffer status":dbl)
      }
      frame Enabled {
      }
    }
    n29 = case shown="True" w366 {
      frame False {
      }
      frame True {
        n30 = call <vilib>:"Beep.vi"() -> ()  [unwired: 12 in]
        "Buffer Overflow" <- TRUE
      }
    }
    n31 = local read "Cal values"() -> (w358:T1)
    n32 = Index Array(array=w135, index (row)=4) -> (element=w235:dbl[])  [unwired: 1 in]
    n33 = Index Array(array=w135, index (row)=0) -> (element=w245:dbl[])  [unwired: 1 in]
    n34 = Index Array(array=w135, index (row)=2) -> (element=w240:dbl[])  [unwired: 1 in]
    n35 = Index Array(array=w135, index (row)=1) -> (element=w244:dbl[])  [unwired: 1 in]
    n36 = Index Array(array=w135, index (row)=3) -> (element=w238:dbl[])  [unwired: 1 in]
    n37 = Index Array(array=w135, index (row)=6) -> (element=w237:dbl[])  [unwired: 1 in]
    n38 = Index Array(array=w135, index (row)=7) -> (element=w236:dbl[])  [unwired: 1 in]
    n39 = Index Array(array=w135, index (row)=5) -> (element=w234:dbl[])  [unwired: 1 in]
    n40 = Unbundle(w358) -> ("AX alpha"=w346:dbl, "BX alpha"=w342:dbl, "AX kappa"=w338:dbl, "BX kappa"=w334:dbl, "AX offset"=w352:dbl, "BX offset"=w350:dbl, "AY alpha"=w349:dbl, "BY alpha"=w344:dbl, "AY kappa"=w340:dbl, "BY kappa"=w336:dbl, "AY offset"=w356:dbl, "BY offset"=w354:dbl)
    n41 = Multiply(x=w244, y=w243) -> (x*y=w239:dbl[])
    n42 = Multiply(x=w245, y=w243) -> (x*y=w241:dbl[])
    n43 = local write "AX alpha"(w346) -> ()
    n44 = local write "BY offset"(w354) -> ()
    n45 = Build Array(w241, w240, w239, w238, w237, w236, w235, w234) -> (w164:dbl[][])
    n46 = local write "BX alpha"(w342) -> ()
    n47 = case shown="True" "Reset data stream" {
      selector: "Reset data stream" -> [_ w573]
      tunnel: w110 -> [w565 w571]
      tunnel: [w565 w569] -> w318
      tunnel: w246 -> [w564 w568]
      tunnel: [w564 w566] -> _
      frame False {
      }
      frame True {
        n48 = Not(x=w573) -> (.not. x?=w572:bool)
        n49 = call <vilib>:"DAQmx Stop Task.vi"("task/channels in"=w571, "error in"=w568) -> ("task out"=w570:refnum<k21>, "error out"=w567:errorcluster)  [unwired: 12 in]
        n50 = local write "Reset data stream"(w572) -> ()
        n51 = local write "Buffer Overflow"(w572) -> ()
        n52 = call <vilib>:"DAQmx Start Task.vi"("task/channels in"=w570, "error in"=w567) -> ("task out"=w569:refnum<k21>, "error out"=w566:errorcluster)  [unwired: 12 in]
      }
    }
    n53 = call-poly <vilib>:"Mean.vi"("X"=w234) -> ("mean"=w372:dbl)  [unwired: 1 out]
    n54 = local write "AY offset"(w356) -> ()
    n55 = call-poly <vilib>:"Mean.vi"("X"=w235) -> ("mean"=w373:dbl)  [unwired: 1 out]
    n56 = call-poly <vilib>:"Mean.vi"("X"=w240) -> ("mean"=w379:dbl)  [unwired: 1 out]
    n57 = call-poly <vilib>:"Mean.vi"("X"=w238) -> ("mean"=w377:dbl)  [unwired: 1 out]
    n58 = call-poly <vilib>:"Mean.vi"("X"=w237) -> ("mean"=w376:dbl)  [unwired: 1 out]
    n59 = call-poly <vilib>:"Mean.vi"("X"=w236) -> ("mean"=w375:dbl)  [unwired: 1 out]
    n60 = local read "Averaging Number"() -> (w133:i32)
    n61 = local write "BY kappa"(w336) -> ()
    n62 = local write "AX kappa"(w338) -> ()
    n63 = call-poly <vilib>:"Mean.vi"("X"=w239) -> ("mean"=w378:dbl)  [unwired: 1 out]
    n64 = local write "AY kappa"(w340) -> ()
    n65 = call-poly <vilib>:"Mean.vi"("X"=w241) -> ("mean"=w380:dbl)  [unwired: 1 out]
    n66 = local read "DAQ rate\n(Samples/s)"() -> (w142:dbl)
    n67 = Build Array(w373, w372) -> (w371:dbl[])
    n68 = local write "BX kappa"(w334) -> ()
    n69 = local write "BY alpha"(w344) -> ()
    n70 = local write "AX offset"(w352) -> ()
    n71 = local write "BX offset"(w350) -> ()
    n72 = local write "AY alpha"(w349) -> ()
    n73 = Build Array(w380, w379, w378, w377, w376, w375) -> (w369:dbl[])
    n74 = Divide(x=w133, y=w142) -> (x/y=w139:dbl)
    "Data update period (s/set)" <- w139
    n75 = Reciprocal(x=w142) -> (1/x=w143:dbl)
    "Data period (s)" <- w143
    n76 = Divide(x=w380, y=w376) -> (x/y=w410:dbl)
    n77 = Divide(x=w379, y=w376) -> (x/y=w411:dbl)
    n78 = Divide(x=w378, y=w375) -> (x/y=w418:dbl)
    n79 = Divide(x=w377, y=w375) -> (x/y=w419:dbl)
    n80 = Subtract(x=w410, y="AY offset") -> (x-y=w392:dbl)
    n81 = Subtract(x=w411, y="AX offset") -> (x-y=w393:dbl)
    n82 = Subtract(x=w418, y="BY offset") -> (x-y=w391:dbl)
    n83 = Subtract(x=w419, y="BX offset") -> (x-y=w394:dbl)
    n84 = Subtract(x=w418, y=w410) -> (x-y=w408:dbl)
    n85 = Subtract(x=w419, y=w411) -> (x-y=w409:dbl)
    n86 = feedback #1(0.0) -> (w317:dbl)
    n87 = Multiply(x="Downsamp\nfact", y=w143) -> (x*y=w144:dbl)
    n88 = Multiply(x=w392, y="AY alpha") -> (x*y=w326:dbl)
    n89 = Multiply(x=w393, y="AX alpha") -> (x*y=w324:dbl)
    n90 = Multiply(x=w394, y="BX alpha") -> (x*y=w325:dbl)
    n91 = Multiply(x=w391, y="BY alpha") -> (x*y=w327:dbl)
    n92 = Add(x=w139, y=w317) -> (x+y=w315:dbl)
    n93 = feedback-in #1(w315) -> ()
    n94 = Square(x=w326) -> (x^2=w402:dbl)
    n95 = Square(x=w324) -> (x^2=w403:dbl)
    n96 = Square(x=w327) -> (x^2=w404:dbl)
    n97 = Square(x=w325) -> (x^2=w405:dbl)
    n98 = Bundle(w408, w409) -> (w136:cluster{dbl, dbl})  [unwired: 1 in]
    n99 = case shown="True" "Set reading to\nsetpoint" {
      tunnel: w136 -> [_ w562]
      frame False {
      }
      frame True {
        n100 = local write "Set reading to\nsetpoint"(FALSE ("Set reading to\nsetpoint")) -> ()
        n101 = local read "Trap position (V)"() -> (w561:cluster{"X":dbl, "Y":dbl})
        n102 = property on="Setpoint voltage" class="Clust (strict)"("Val(Sgnl)"=w562) -> ()  [unwired: 2 in, 2 out]
        n103 = Unbundle(w561) -> ("X"=w560:dbl, "Y"=w559:dbl)
        n104 = Bundle("Y"=w559, "X"=w560) -> (w558:cluster{"Y":dbl, "X":dbl})  [unwired: 1 in]
        n105 = property on="Offset" class="Clust (strict)"("Val(Sgnl)"=w558) -> ()  [unwired: 2 in, 2 out]
      }
    }
    n106 = Reciprocal(x=w144) -> (1/x=→"Chart Freq (Hz)":dbl)
    n107 = To Time Stamp(1:w315) -> (0:w314:timestamp)
    n108 = Add(x=w402, y=w403) -> (x+y=w406:dbl)
    n109 = Add(x=w404, y=w405) -> (x+y=w417:dbl)
    n110 = Multiply(x=w324, y="AX kappa") -> (x*y=w320:dbl)
    n111 = Bundle("A y", "A x", "B y", "B x", "A sum", "B sum", "Trap x", "Trap y") -> (w305:T11)  [unwired: 1 in]
    n112 = Multiply(x=w325, y="BX kappa") -> (x*y=w321:dbl)
    n113 = Square Root(x=w406) -> (sqrt(x)=w422:dbl)
    n114 = Square Root(x=w417) -> (sqrt(x)=w421:dbl)
    n115 = Multiply(x=w326, y="AY kappa") -> (x*y=w322:dbl)
    n116 = Multiply(x=w327, y="BY kappa") -> (x*y=w323:dbl)
    n117 = Subtract(x=w372, y="Fixed Y") -> (x-y=w407:dbl)
    n118 = Subtract(x=w373, y="Fixed X") -> (x-y=w412:dbl)
    n119 = Cluster To Array(cluster=w305) -> (array=w304:string[])
    n120 = for {
      tunnel: w164 -> [w550] mode=indexing
      tunnel: w144 -> [w549]
      tunnel: "Downsamp\nfact" -> [w555]
      tunnel: [w553] -> w220 mode=indexing
      tunnel: w314 -> [w557]
      tunnel: w304 -> [w552] mode=indexing
      tunnel: "NI_ChannelName" ("name") -> [w551]
      n121 = call "Downsample 1D array.vi"("Ave N"=w555, "Arrray In"=w550) -> ("Array Out"=w556:dbl[])  [unwired: 9 in]
      n122 = Bundle By Name("Y"=w556, "dt"=w549, "t0"=w557) -> (w554:waveform(dbl))  [unwired: 1 in]
      n123 = Set Waveform Attribute(5:w552, 6:w551, 7:w554) -> (3:w553:waveform(dbl))  [unwired: 1 in, 2 out]
    }
    "All signals" <- w220
    n124 = Square(x=w322) -> (x^2=w395:dbl)
    n125 = Square(x=w320) -> (x^2=w396:dbl)
    n126 = Square(x=w323) -> (x^2=w397:dbl)
    n127 = Square(x=w321) -> (x^2=w398:dbl)
    n128 = Add(x=w395, y=w396) -> (x+y=w399:dbl)
    n129 = Add(x=w397, y=w398) -> (x+y=w400:dbl)
    n130 = Multiply(x=w407, y="Conv Y (nm/V)") -> (x*y=w329:dbl)
    n131 = Multiply(x=w412, y="Conv X (nm/V)") -> (x*y=w330:dbl)
    n132 = feedback #2() -> (w367:cluster{"B_Y":dbl, "B_X":dbl})  [unwired: 1 in]
    n133 = case shown="True" "Force Feedback" {
      tunnel: [w847 w863] -> w127
      tunnel: [w846 w862] -> w125
      tunnel: w136 -> [_ w861]
      tunnel: [cluster{"B_Y":dbl, "B_X":dbl} {"B_Y"=0.0, "B_X"=0.0} ("Sum error past") w853] -> w368
      tunnel: w367 -> [_ w860]
      tunnel: w426 -> [w847 w856]
      tunnel: w431 -> [w846 w855]
      frame False {
        # "Force feedback"
      }
      frame True {
        n134 = call "ForceFeedback2.vi"("PSD/Mirror Voltages"=w861, "Sum error"=w860, "task/channels in"=w856, "error in"=w855, "Desired voltage"="Setpoint voltage", "Feedback const"="Feedback const", "offset"="Offset") -> ("task out"=w863:refnum<k21>, "Sum error past"=w853:cluster{"B_Y":dbl, "B_X":dbl}, "Output Voltage"=→"Feedback Output Voltage 2":cluster{dbl, dbl}, "error out"=w862:errorcluster)  [unwired: 8 in, 1 out]
        n135 = local read "Pulling direction"() -> (w852:bool)
        n136 = Unbundle(w853) -> ("B_Y"=w850:dbl, "B_X"=w849:dbl)
        n137 = Select(t=w850, s=w852, f=w849) -> (s? t:f=→"Sum error":dbl)
      }
    }
    n138 = feedback-in #2(w368) -> ()
    n139 = Square Root(x=w399) -> (sqrt(x)=w328:dbl)
    n140 = Square Root(x=w400) -> (sqrt(x)=w423:dbl)
    n141 = Add(x=w328, y=w423) -> (x+y=w401:dbl)
    n142 = Build Array(w410, w411, w418, w419, w376, w375, w328, w423, w422, w421, w330, w329) -> ()  [unwired: 1 out]
    n143 = Divide(x=w401, y=2.0) -> (x/y=w365:dbl)
    n144 = Index Array(array=w220, index=6) -> (element=w169:waveform(dbl))
    n145 = Index Array(array=w220, index=7) -> (element=w171:waveform(dbl))
    n146 = local read "Fixed X"() -> (w224:dbl)
    n147 = local read "Fixed Y"() -> (w226:dbl)
    n148 = Unbundle By Name(w169) -> ("Y"=w228:dbl[])
    n149 = Unbundle By Name(w171) -> ("Y"=w227:dbl[])
    n150 = Index Array(array=w220, index=0) -> (element=w177:waveform(dbl))
    n151 = Index Array(array=w220, index=1) -> (element=w301:waveform(dbl))
    n152 = Index Array(array=w220, index=4) -> (element=w295:waveform(dbl))
    n153 = Subtract(x=w228, y=w224) -> (x-y=w225:dbl[])
    n154 = Subtract(x=w227, y=w226) -> (x-y=w222:dbl[])
    n155 = Unbundle By Name(w177) -> ("Y"=w293:dbl[])
    n156 = Unbundle By Name(w301) -> ("Y"=w292:dbl[])
    n157 = Unbundle By Name(w295) -> ("Y"=w291:dbl[])
    n158 = Index Array(array=w220, index=5) -> (element=w294:waveform(dbl))
    n159 = local read "Conv X (nm/V)"() -> (w223:dbl)
    n160 = local read "Conv Y (nm/V)"() -> (w221:dbl)
    n161 = Index Array(array=w220, index=2) -> (element=w174:waveform(dbl))
    n162 = Index Array(array=w220, index=3) -> (element=w298:waveform(dbl))
    n163 = Set Waveform Attribute(5:"T2 X", 6:w167, 7:w169) -> (3:w168:waveform(dbl))  [unwired: 1 in, 2 out]
    n164 = Set Waveform Attribute(5:"T2 Y", 6:w167, 7:w171) -> (3:w170:waveform(dbl))  [unwired: 1 in, 2 out]
    n165 = Unbundle By Name(w294) -> ("Y"=w288:dbl[])
    n166 = Unbundle By Name(w174) -> ("Y"=w290:dbl[])
    n167 = Unbundle By Name(w298) -> ("Y"=w289:dbl[])
    n168 = Divide(x=w293, y=w291) -> (x/y=w192:dbl[])
    n169 = Divide(x=w292, y=w291) -> (x/y=w190:dbl[])
    n170 = local read "AY offset"() -> (w279:dbl)
    n171 = local read "AX offset"() -> (w277:dbl)
    n172 = Multiply(x=w225, y=w223) -> (x*y=w161:dbl[])
    n173 = Multiply(x=w222, y=w221) -> (x*y=w163:dbl[])
    n174 = Divide(x=w289, y=w288) -> (x/y=w191:dbl[])
    n175 = Subtract(x=w190, y=w277) -> (x-y=w280:dbl[])
    n176 = local read "BY offset"() -> (w284:dbl)
    n177 = local read "BX offset"() -> (w287:dbl)
    n178 = Subtract(x=w192, y=w279) -> (x-y=w281:dbl[])
    n179 = Divide(x=w290, y=w288) -> (x/y=w193:dbl[])
    n180 = local read "AY alpha"() -> (w278:dbl)
    n181 = local read "AX alpha"() -> (w276:dbl)
    n182 = call-poly <vilib>:"Mean.vi"("X"=w163) -> ("mean"=w203:dbl)  [unwired: 1 out]
    "Mean Trp Pos Y 2 (nm)" <- w203
    n183 = Subtract(x=w193, y=w192) -> (x-y=w189:dbl[])
    n184 = Subtract(x=w191, y=w190) -> (x-y=w188:dbl[])
    n185 = Subtract(x=w161, y="Offset X (nm)") -> (x-y=w160:dbl[])
    n186 = Subtract(x=w163, y="Offset Y (nm)") -> (x-y=w162:dbl[])
    n187 = Subtract(x=w193, y=w284) -> (x-y=w286:dbl[])
    n188 = Subtract(x=w191, y=w287) -> (x-y=w285:dbl[])
    n189 = Subtract(x=w203, y=w163) -> (x-y=w202:dbl[])
    n190 = call-poly <vilib>:"Mean.vi"("X"=w161) -> ("mean"=w207:dbl)  [unwired: 1 out]
    "Mean Trap Pos X 2 (nm)" <- w207
    n191 = Build Array(w189, w188) -> (w186:dbl[][])
    n192 = Index Array(array=w186, index (row)=0) -> (element=w184:dbl[])  [unwired: 1 in]
    n193 = Index Array(array=w186, index (row)=1) -> (element=w183:dbl[])  [unwired: 1 in]
    n194 = call-poly <vilib>:"Mean.vi"("X"=w184) -> ("mean"=w182:dbl)  [unwired: 1 out]
    n195 = call-poly <vilib>:"Mean.vi"("X"=w183) -> ("mean"=w181:dbl)  [unwired: 1 out]
    n196 = Bundle("mean"=w182, "mean"=w181) -> ()  [unwired: 1 in, 1 out]
    n197 = local read "BY alpha"() -> (w283:dbl)
    n198 = local read "BX alpha"() -> (w282:dbl)
    n199 = Multiply(x=w281, y=w278) -> (x*y=w269:dbl[])
    n200 = Multiply(x=w280, y=w276) -> (x*y=w268:dbl[])
    n201 = Square(x=w202) -> (x^2=w201:dbl[])
    n202 = Subtract(x=w207, y=w161) -> (x-y=w206:dbl[])
    n203 = Bundle By Name(cluster=w170, "Y"=w162) -> (w218:waveform(dbl))
    n204 = Bundle By Name(cluster=w168, "Y"=w160) -> (w219:waveform(dbl))
    n205 = local read "Raster scanning..."() -> (w109:bool)
    n206 = local read "Saving"() -> (w331:bool)
    n207 = local read "Tether"() -> (w332:bool)
    n208 = Square(x=w206) -> (x^2=w205:dbl[])
    n209 = call-poly <vilib>:"Mean.vi"("X"=w201) -> ("mean"=w200:dbl)  [unwired: 1 out]
    n210 = Square(x=w269) -> (x^2=w275:dbl[])
    n211 = Multiply(x=w286, y=w283) -> (x*y=w267:dbl[])
    n212 = Square(x=w268) -> (x^2=w274:dbl[])
    n213 = Multiply(x=w285, y=w282) -> (x*y=w266:dbl[])
    n214 = Less?(x=w365, y="Tether break\nforce (pN)") -> (x < y?=w363:bool)
    n215 = call-poly <vilib>:"Mean.vi"("X"=w205) -> ("mean"=w204:dbl)  [unwired: 1 out]
    n216 = Build Array(w219, w218) -> (w128:waveform(dbl)[])
    "Trap sep" <- w128
    n217 = Square Root(x=w200) -> (sqrt(x)=w199:dbl)
    n218 = Square(x=w267) -> (x^2=w273:dbl[])
    n219 = Square(x=w266) -> (x^2=w272:dbl[])
    n220 = Add(x=w275, y=w274) -> (x+y=w271:dbl[])
    n221 = Square Root(x=w204) -> (sqrt(x)=w197:dbl)
    n222 = Compound Arithmetic op=AND(w331, w332, w363) -> (w362:bool)
    n223 = Multiply(x=w199, y=10) -> (x*y=→"T2 Y RMS (A)":dbl)
    n224 = Square Root(x=w271) -> (sqrt(x)=w156:dbl[])
    n225 = Add(x=w273, y=w272) -> (x+y=w270:dbl[])
    n226 = Set Waveform Attribute(5:"T2", 6:"NI_ChannelName" ("name"), 7:w177) -> (3:w176:waveform(dbl))  [unwired: 1 in, 2 out]
    n227 = Set Waveform Attribute(5:"T1", 6:"NI_ChannelName" ("name"), 7:w174) -> (3:w173:waveform(dbl))  [unwired: 1 in, 2 out]
    n228 = case shown="True" w362 {
      selector: w362 -> [_ w580]
      tunnel: w109 -> [w574 w575]
      tunnel: [w574 w575] -> w108
      frame False {
      }
      frame True {
        n229 = call <vilib>:"Beep.vi"() -> ()  [unwired: 12 in]
        n230 = Not(x=w580) -> (.not. x?=w578:bool)
        n231 = And(x=w575, y="Fish After TA?") -> (x .and. y?=w577:bool)
        n232 = local write "Tether"(w578) -> ()
        n233 = local write "Force Feedback"(w578) -> ()
        n234 = case shown="True" w577 {
          selector: w577 -> [_ w581]
          frame False {
          }
          frame True {
            n235 = property on="Fish" class="Bool (strict)"("Val(Sgnl)"=w581) -> ()  [unwired: 2 in, 2 out]
          }
        }
        n236 = property on="Stop saving" class="Bool (strict)"("Val(Sgnl)"="TA Cancel Save?") -> ()  [unwired: 2 in, 2 out]
      }
    }
    n237 = Square Root(x=w270) -> (sqrt(x)=w155:dbl[])
    n238 = Multiply(x=w197, y=10) -> (x*y=→"T2 X RMS (A)":dbl)
    n239 = Bundle By Name(cluster=w176, "Y"=w156) -> (w180:waveform(dbl))
    n240 = Bundle By Name(cluster=w173, "Y"=w155) -> (w248:waveform(dbl))
    n241 = Add(x=w156, y=w155) -> (x+y=w154:dbl[])
    n242 = case shown="True" "Remove offsets" {
      selector: "Remove offsets" -> [_ w547]
      frame False {
      }
      frame True {
        n243 = local read "Mean Trp Pos Y 2 (nm)"() -> (w545:dbl)
        n244 = Not(x=w547) -> (.not. x?=w548:bool)
        n245 = local read "Mean Trap Pos X 2 (nm)"() -> (w546:dbl)
        n246 = local write "Remove offsets"(w548) -> ()
        n247 = local write "Offset Y (nm)"(w545) -> ()
        n248 = local write "Offset X (nm)"(w546) -> ()
      }
    }
    n249 = Build Array(w180, w248) -> (→"Bead sep":waveform(dbl)[])
    n250 = local read "AY kappa"() -> (w265:dbl)
    n251 = local read "AX kappa"() -> (w264:dbl)
    n252 = Divide(x=w154, y=2) -> (x/y=w152:dbl[])
    n253 = local read "BX kappa"() -> (w262:dbl)
    n254 = local read "BY kappa"() -> (w263:dbl)
    n255 = call-poly <vilib>:"Mean.vi"("X"=w152) -> ("mean"=w151:dbl)  [unwired: 1 out]
    "Mean Bead Sep\n(nm)" <- w151
    n256 = local read "Calibrating"() -> (w424:bool)
    n257 = Multiply(x=w269, y=w265) -> (x*y=w258:dbl[])
    n258 = Multiply(x=w268, y=w264) -> (x*y=w259:dbl[])
    n259 = Square(x=w258) -> (x^2=w257:dbl[])
    n260 = Square(x=w259) -> (x^2=w256:dbl[])
    n261 = Subtract(x=w152, y=w151) -> (x-y=w150:dbl[])
    n262 = Multiply(x=w267, y=w263) -> (x*y=w260:dbl[])
    n263 = Multiply(x=w266, y=w262) -> (x*y=w261:dbl[])
    n264 = Or(x=w108, y="Raster scan") -> (x .or. y?=w123:bool)
    n265 = Add(x=w257, y=w256) -> (x+y=w253:dbl[])
    n266 = Square(x=w150) -> (x^2=w149:dbl[])
    n267 = Square Root(x=w253) -> (sqrt(x)=w217:dbl[])
    n268 = Square(x=w260) -> (x^2=w255:dbl[])
    n269 = Square(x=w261) -> (x^2=w254:dbl[])
    n270 = call-poly <vilib>:"Mean.vi"("X"=w149) -> ("mean"=w148:dbl)  [unwired: 1 out]
    n271 = Add(x=w255, y=w254) -> (x+y=w252:dbl[])
    n272 = Bundle By Name(cluster=w176, "Y"=w217) -> (w251:waveform(dbl))
    n273 = local read "Saving"() -> (w361:bool)
    n274 = Or(x=w424, y=w361) -> ()  [unwired: 1 out]
    n275 = Square Root(x=w148) -> (sqrt(x)=w147:dbl)
    n276 = Square Root(x=w252) -> (sqrt(x)=w216:dbl[])
    n277 = Multiply(x=10, y=w147) -> (x*y=→"Bead Sep Noise\n(A)":dbl)
    n278 = Bundle By Name(cluster=w173, "Y"=w216) -> (w250:waveform(dbl))
    n279 = Add(x=w217, y=w216) -> (x+y=w215:dbl[])
    n280 = Build Array(w251, w250) -> (→"Force (pN)":waveform(dbl)[])
    n281 = Divide(x=w215, y=2) -> (x/y=w212:dbl[])
    n282 = call-poly <vilib>:"Mean.vi"("X"=w212) -> ("mean"=w213:dbl)  [unwired: 1 out]
    "Mean force (pN)" <- w213
    n283 = Subtract(x=w213, y=w212) -> (x-y=w211:dbl[])
    n284 = Square(x=w211) -> (x^2=w210:dbl[])
    n285 = call-poly <vilib>:"Mean.vi"("X"=w210) -> ("mean"=w209:dbl)  [unwired: 1 out]
    n286 = Square Root(x=w209) -> (sqrt(x)=→"Force noise (pN)":dbl)
    n287 = flat-sequence {
      tunnel: w424 -> [w621]
      tunnel: w361 -> [_]
      tunnel: w424 -> [_]
      tunnel: w361 -> [_]
      tunnel: w164 -> [w608]
      tunnel: [w608] -> w382
      tunnel: w246 -> [w607]
      tunnel: [w607] -> w381
      tunnel: w369 -> [w606]
      tunnel: [w606] -> w374
      tunnel: w371 -> [w605]
      tunnel: [w605] -> w370
      tunnel: [w602] -> w360
      tunnel: [w599] -> w359
      tunnel: [w596] -> w233
      tunnel: [w595] -> w232
      tunnel: [w592] -> w231
      tunnel: w130 -> [w589]
      tunnel: ["Save Data"] -> w129
      tunnel: w382 -> [w769]
      tunnel: w381 -> [w768]
      tunnel: w374 -> [_]
      tunnel: w370 -> [_]
      tunnel: w360 -> [w767]
      tunnel: w359 -> [w766]
      tunnel: w233 -> [w765]
      tunnel: w232 -> [w764]
      tunnel: w231 -> [w763]
      tunnel: w129 -> [w761]
      tunnel: w128 -> [w760]
      frame #0 {
        w587 = 0.0
        # "1: old trap\n0: fleezers"
        # "Create files if saving data"
        n288 = local read "Save N sets"() -> (w591:bool)
        n289 = local read "Sampling Rate"() -> (w619:dbl)
        n290 = Or(x=w591, y="Save Data") -> (x .or. y?=w590:bool)
        n291 = Build Array(w590, "Save cal", w589) -> (w610:bool[])
        n292 = Compound Arithmetic op=OR("Save Data", "Save cal", w589) -> (w612:bool)
        n293 = Boolean Array To Number(Boolean array=w610) -> (number=w609:u32)
        n294 = local read "Trap position (V)"() -> (w616:cluster{"X":dbl, "Y":dbl})
        n295 = local read "Fixed X"() -> (w586:dbl)
        n296 = local read "Fixed Y"() -> (w585:dbl)
        n297 = Unbundle(w616) -> ("X"=w584:dbl, "Y"=w583:dbl)
        n298 = Build Array(w584, w583, w586, w585, w587, w587) -> (w615:dbl[])
        n299 = feedback #3(refnum<k0> refnum) -> (w600:refnum<file>)
        n300 = feedback #4() -> (w597:dbl)  [unwired: 1 in]
        n301 = feedback #5(FALSE) -> (w593:bool)
        n302 = feedback #6(0) -> (w613:i32)
        n303 = feedback #7(refnum<k0> refnum) -> (w603:refnum<file>)
        n304 = case shown="True" w612 {
          tunnel: w621 -> [_ _]
          tunnel: 9 -> [_ w664]
          tunnel: w619 -> [_ w663]
          tunnel: 6 -> [_ w662]
          tunnel: 5 -> [_ w661]
          tunnel: w615 -> [_ w660]
          tunnel: [w626 1] -> w596
          tunnel: w613 -> [w627 _]
          tunnel: w609 -> [_ w635]
          tunnel: [w625 w633] -> w602
          tunnel: w603 -> [w625 _]
          tunnel: [w624 w632] -> w599
          tunnel: w600 -> [w624 _]
          tunnel: 1.0 -> [_ w631]
          tunnel: [w623 w630] -> w595
          tunnel: w597 -> [w623 _]
          tunnel: [w622 w629] -> w592
          tunnel: w593 -> [w622 _]
          frame False {
            n305 = Increment(x=w627) -> (x+1=w626:i32)
          }
          frame True {
            w636 = FALSE ("Save Data")
            w642 = FALSE
            w643 = T10."big-endian, network order" ("byte order (0:big-endian, network order)")
            n306 = local write "Save cal"(w636) -> ()
            n307 = local write "Save Data"(w636) -> ()
            n308 = case shown="4" w635 {
              tunnel: w664 -> [w711 w729 w759]
              tunnel: w663 -> [w689 w728 w734]
              tunnel: w662 -> [w710 w726 w755]
              tunnel: w661 -> [w709 w725 w754]
              tunnel: w660 -> [w707 w722 w751]
              tunnel: [w706 w721 w740] -> w657
              tunnel: [w708 w718 w739] -> w629
              tunnel: ["Averaging Number" 200 w737] -> _
              tunnel: w631 -> [w694 w713 w736]
              tunnel: [w690 "Cal sets to save" w730] -> w630
              frame 1, Default {
                w708 = TRUE
                w695 = 0.0
                # "Time trace"
                n309 = local read "Averaging Number"() -> (w705:i32)
                n310 = Boolean To (0,1)(Boolean=w708) -> (0, 1=w700:i16)
                n311 = Increment(x=w700) -> (x+1=w699:i16)
                n312 = Divide(x=w689, y=w705) -> (x/y=w704:dbl)
                n313 = To Double Precision Float(number=w699) -> (double precision float=w698:dbl)
                n314 = Reciprocal(x=w704) -> (1/x=w703:dbl)
                n315 = Reciprocal(x=w689) -> (1/x=w688:dbl)
                n316 = Build Array(w711, w688, w703, w710, w709, 0 ("f")) -> (w702:dbl[])
                n317 = Build Array(w698, w694, w695, w695, w695) -> (w701:dbl[])
                n318 = Build Array (concatenate)(w702, w707, w701) -> (w706:dbl[])
                n319 = Select(t="N sets", s="Save N sets", f=2147483647) -> (s? t:f=w690:i32)
              }
              frame 2 {
                w718 = FALSE
                w716 = 0.0
                # "Calibration file"
                n320 = Reciprocal(x=w728) -> (1/x=w727:dbl)
                n321 = Boolean To (0,1)(Boolean=w718) -> (0, 1=w720:i16)
                n322 = To Double Precision Float(number=w720) -> (double precision float=w719:dbl)
                n323 = Build Array(w729, w727, w727, w726, w725, 1) -> (w723:dbl[])
                n324 = Build Array(w719, w713, w716, w716, w716) -> (w717:dbl[])
                n325 = Build Array (concatenate)(w723, w722, w717) -> (w721:dbl[])
                "Calibrating" <- TRUE ("Calibrating")
              }
              frame 4 {
                w747 = 0.0
                w739 = TRUE
                # "Not using ncycles"
                # "FX curve"
                n326 = local read "Averaging Number"() -> (w758:i32)
                n327 = Boolean To (0,1)(Boolean=w739) -> (0, 1=w750:i16)
                n328 = Increment(x=w750) -> (x+1=w749:i16)
                n329 = local write "Raster scan"(FALSE ("Raster scan")) -> ()
                n330 = To Double Precision Float(number=w749) -> (double precision float=w748:dbl)
                n331 = Divide(x=w734, y=w758) -> (x/y=w757:dbl)
                n332 = Reciprocal(x=w757) -> (1/x=w756:dbl)
                n333 = Build Array(w748, w736, w747, w747, w747) -> (w746:dbl[])
                n334 = Reciprocal(x=w734) -> (1/x=w733:dbl)
                n335 = Build Array(w759, w733, w756, w755, w754, 2) -> (w752:dbl[])
                n336 = local read "Pulling direction"() -> (w744:bool)
                n337 = local read "Scan range (V)"() -> (w731:dbl)
                n338 = local read "N sets to be saved"() -> (w730:dbl)
                n339 = local read "Scan steps (mirror)"() -> (w732:u64)
                n340 = local read "# scans"() -> (w742:i32)
                n341 = Not(x=w744) -> (.not. x?=w743:bool)
                n342 = local read "Averaging Number"() -> (w737:i32)
                n343 = Boolean To (0,1)(Boolean=w743) -> (0, 1=w745:i16)
                n344 = Build Array(w745, w731, w732, 0, w742) -> (w741:dbl[])
                n345 = Build Array (concatenate)(w752, w751, w746, w741) -> (w740:dbl[])
              }
            }
            n346 = call "CreateSaveFile.vi"("Index In"="Save file index", "Ext"=".dat", "Insert"="", "Directory"="Path") -> ("Index Out"=w628:i32, "Path Out"=w641:path)  [unwired: 6 in]
            "Current file name" <- w641
            n347 = Open/Create/Replace File(file path (use dialog)=w641, operation (0:open)=T9."create", access (0:read/write)=enum16{"read/write", "read-only", "write-only"}."write-only") -> (refnum out=w650:refnum<file>, error out=w651:errorcluster)  [unwired: 3 in, 1 out]
            n348 = local write "Save file index"(w628) -> ()
            n349 = Array Size(array=w657) -> (size(s)=w659:i32)
            n350 = case shown="True" w629 {
              tunnel: w641 -> [_ w687]
              tunnel: [refnum<k0> refnum w666] -> w632
              frame False {
              }
              frame True {
                w673 = 0.0
                n351 = Path To String(path=w687) -> (string=w683:string)
                n352 = Build Array(w673, w673, w673, w673, w673, w673, w673, w673) -> (w670:dbl[])
                n353 = String Length(string=w683) -> (length=w686:i32)
                n354 = Array Size(array=w670) -> (size(s)=w672:i32)
                n355 = Subtract(x=w686, y=4) -> (x-y=w684:i32)
                n356 = To Double Precision Float(number=w672) -> (double precision float=w671:dbl)
                n357 = String Subset(string=w683, length (rest)=w684) -> (substring=w682:string)  [unwired: 1 in]
                n358 = Build Array (concatenate)(w671, w670) -> (w669:dbl[])
                n359 = Concatenate Strings(w682, "_pos.dat" ("string")) -> (w680:string)
                n360 = String To Path(string=w680) -> (path=w679:path)
                n361 = Open/Create/Replace File(file path (use dialog)=w679, operation (0:open)=T9."create", access (0:read/write)=enum16{"read/write", "read-only", "write-only"}."write-only") -> (refnum out=w675:refnum<file>, error out=w676:errorcluster)  [unwired: 3 in, 1 out]
                n362 = Deny Access(4:w676, 7:w675) -> (3:w674:refnum<file>)  [unwired: 1 in, 1 out]
                n363 = Write to Binary File(file (use dialog)=w674, data=w669, 5:FALSE ("prepend array or string size? (T)"), 9:T10."big-endian, network order" ("byte order (0:big-endian, network order)")) -> (refnum out=w666:refnum<file>)  [unwired: 2 in, 2 out]
              }
            }
            n364 = Deny Access(4:w651, 7:w650) -> (0:w640:errorcluster, 3:w649:refnum<file>)  [unwired: 1 in]
            n365 = String Length(string="Comment") -> (length=w656:i32)
            n366 = To Double Precision Float(number=w659) -> (double precision float=w658:dbl)
            n367 = To Double Precision Float(number=w656) -> (double precision float=w655:dbl)
            n368 = Build Array (concatenate)(w658, w657, w655) -> (w646:dbl[])
            n369 = Write to Binary File(file (use dialog)=w649, data=w646, error in=w640, 5:w642, 9:w643) -> (refnum out=w645:refnum<file>, error out=w639:errorcluster)  [unwired: 1 in, 1 out]
            n370 = Write to Binary File(file (use dialog)=w645, data="Comment", error in=w639, 5:w642, 9:w643) -> (refnum out=w633:refnum<file>)  [unwired: 1 in, 2 out]
            "Saving" <- TRUE
          }
        }
        n371 = feedback-in #3(w599) -> ()
        n372 = feedback-in #4(w595) -> ()
        n373 = feedback-in #5(w592) -> ()
        n374 = feedback-in #6(w596) -> ()
        n375 = feedback-in #7(w602) -> ()
      }
      frame #1 {
        n376 = local read "Saving"() -> (w762:bool)
        n377 = case shown="True" w762 {
          tunnel: w769 -> [_ w788]
          tunnel: w768 -> [_ w787]
          tunnel: w767 -> [_ w786]
          tunnel: w766 -> [_ w785]
          tunnel: w765 -> [_ w775]
          tunnel: w764 -> [_ w776]
          tunnel: w763 -> [_ w779]
          tunnel: w761 -> [_ w771]
          tunnel: w760 -> [_ w770]
          frame False {
            (unwired) FALSE ("Calibrating")
          }
          frame True {
            n378 = local read "Stop"() -> (w783:bool)
            n379 = Less Or Equal?(x=w775, y=w776) -> (x <= y?=w784:bool)
            n380 = Divide(x=w775, y=w776) -> (x/y=w774:dbl)
            n381 = Or(x=w783, y="Stop saving") -> (x .or. y?=w782:bool)
            n382 = Not(x=w782) -> (.not. x?=w781:bool)
            n383 = Multiply(x=100.0, y=w774) -> (x*y=w773:dbl)
            n384 = And(x=w784, y=w781) -> (x .and. y?=w780:bool)
            n385 = case shown="True" w780 {
              tunnel: w786 -> [w793 w802]
              tunnel: w787 -> [_ w801]
              tunnel: w788 -> [_ w800]
              tunnel: w785 -> [w792 w799]
              tunnel: w779 -> [w790 _]
              tunnel: [0.0 ("Progress") w798] -> w778
              tunnel: w773 -> [_ w798]
              tunnel: w771 -> [_ w795]
              tunnel: w770 -> [_ w796]
              frame False {
                w791 = FALSE
                n386 = Close File(refnum=w793) -> ()  [unwired: 1 in, 2 out]
                n387 = case shown="True" w790 {
                  tunnel: w792 -> [_ w794]
                  frame False {
                  }
                  frame True {
                    n388 = Close File(refnum=w794) -> ()  [unwired: 1 in, 2 out]
                  }
                }
                n389 = call <vilib>:"Beep.vi"() -> ()  [unwired: 12 in]
                n390 = local write "Saving"(w791) -> ()
                n391 = local write "Stop saving"(w791) -> ()
                n392 = local write "Calibrating"(w791) -> ()
              }
              frame True {
                n393 = local read "Calibrating"() -> (w797:bool)
                n394 = case shown="True" w797 {
                  tunnel: w802 -> [w829 w845]
                  tunnel: w801 -> [_ w844]
                  tunnel: w800 -> [w816 w838]
                  tunnel: w799 -> [w815 _]
                  tunnel: w796 -> [w807 _]
                  tunnel: w795 -> [_ _]
                  frame False {
                    n395 = local read "Averaging Number"() -> (w823:i32)
                    n396 = Array Subset(array=w816, index (row)=0 ("index"), length (row)=6 ("length")) -> (w812:dbl[][])  [unwired: 2 in]
                    n397 = Array Subset(array=w816, index (row)=6 ("index"), length (row)=2 ("length")) -> (w811:dbl[][])  [unwired: 2 in]
                    n398 = Array Size(array=w811) -> (size(s)=w822:i32[])
                    n399 = Array Size(array=w812) -> (size(s)=w819:i32[])
                    n400 = Index Array(array=w807, index=0) -> (element=w804:waveform(dbl))
                    n401 = Index Array(array=w807, index=1) -> (element=w803:waveform(dbl))
                    n402 = for {
                      tunnel: w812 -> [w833] mode=indexing
                      tunnel: w823 -> [w835]
                      tunnel: [w834] -> w810 mode=indexing
                      n403 = call "Downsample 1D array.vi"("Ave N"=w835, "Arrray In"=w833) -> ("Array Out"=w834:dbl[])  [unwired: 9 in]
                    }
                    n404 = Unbundle By Name(w804) -> ()  [unwired: 1 out]
                    n405 = Unbundle By Name(w803) -> ()  [unwired: 1 out]
                    n406 = Multiply Array Elements(1:w819) -> (0:w818:i32)
                    n407 = for {
                      tunnel: w811 -> [w832] mode=indexing
                      tunnel: w823 -> [w831]
                      tunnel: [w830] -> w814 mode=indexing
                      n408 = call "Downsample 1D array.vi"("Ave N"=w831, "Arrray In"=w832) -> ("Array Out"=w830:dbl[])  [unwired: 9 in]
                    }
                    n409 = Multiply Array Elements(1:w822) -> (0:w821:i32)
                    n410 = Divide(x=w818, y=w823) -> (x/y=w824:dbl)
                    n411 = Divide(x=w821, y=w823) -> (x/y=w820:dbl)
                    n412 = Transpose 2D Array(2D array=w810) -> (transposed array=w809:dbl[][])
                    n413 = Transpose 2D Array(2D array=w814) -> (transposed array=w808:dbl[][])
                    n414 = Reshape Array(w809, w824) -> (w813:dbl[])
                    n415 = Reshape Array(w808, w820) -> (w817:dbl[])
                    n416 = call <vilib>:"Write File+ [SGL].vi"("1D array"=w817, "refnum"=w815) -> ()  [unwired: 7 in, 3 out]
                    n417 = call <vilib>:"Write File+ [SGL].vi"("1D array"=w813, "refnum"=w829) -> ()  [unwired: 7 in, 3 out]
                  }
                  frame True {
                    n418 = Array Subset(array=w838, index (row)=0 ("index"), length (row)=6 ("length")) -> (w836:dbl[][])  [unwired: 2 in]
                    n419 = Transpose 2D Array(2D array=w836) -> (transposed array=w842:dbl[][])
                    n420 = Array Size(array=w836) -> (size(s)=w837:i32[])
                    n421 = Multiply Array Elements(1:w837) -> (0:w843:i32)
                    n422 = Reshape Array(w842, w843) -> (w841:dbl[])
                    n423 = call <vilib>:"Write File+ [SGL].vi"("1D array"=w841, "error in (no error)"=w844, "refnum"=w845) -> ()  [unwired: 6 in, 3 out]
                  }
                }
              }
            }
            "Progress" <- w778
          }
        }
      }
    }
    n424 = local read "Flushing Sample"() -> (w132:bool)
    n425 = case shown="True" w132 {
      frame False {
      }
      frame True {
        n426 = local read "Flush Sample Start Time"() -> (w541:u32)
        n427 = local read "Sample flush time (s)"() -> (w534:dbl)
        n428 = Tick Count (ms)() -> (millisecond timer value=w542:u32)
        n429 = Subtract(x=w542, y=w541) -> (x-y=w532:u32)
        n430 = Multiply(x=u32 1000, y=w534) -> (x*y=w533:dbl)
        n431 = Divide(x=w532, y=w533) -> (x/y=w537:dbl)
        n432 = Greater?(x=w532, y=w533) -> (0:w540:bool)
        n433 = Not(x=w540) -> (.not. x?=w539:bool)
        n434 = Boolean To (0,1)(Boolean=w539) -> (0, 1=w538:i16)
        n435 = Compound Arithmetic op=MULTIPLY(w538, w537, 100.0 ("value")) -> (→"Sample Flush Meter":dbl)
        n436 = case shown="True" w540 {
          frame False {
          }
          frame True {
            w544 = FALSE ("Inject Sample")
            n437 = property on="Clear Volume" class="Bool (strict)"("Val(Sgnl)"=TRUE ("Value (Signaling)")) -> ()  [unwired: 2 in, 2 out]
            n438 = local write "Inject Sample"(w544) -> ()
            n439 = local write "Flushing Sample"(w544) -> ()
          }
        }
      }
    }
    n440 = feedback #8(0) -> (w116:i32)
    n441 = feedback #9(0) -> (w113:i32)
    n442 = feedback #10(0) -> (w118:i32)
    n443 = case shown="True" w123 {
      tunnel: w127 -> [w442 w490]
      tunnel: [w442 w474] -> w126
      tunnel: w125 -> [w441 w489]
      tunnel: [w441 w473] -> w124
      tunnel: "Raster scan" -> [w440 w466]
      tunnel: [w440 w465] -> w121
      tunnel: [0 w464] -> w119
      tunnel: w118 -> [_ w458]
      tunnel: w116 -> [_ w446]
      tunnel: [0 w449] -> w115
      tunnel: w113 -> [_ w455]
      tunnel: [0 w454] -> w112
      frame False {
      }
      frame True {
        # "Reset step counter"
        # "Current position"
        # "Initial values"
        n444 = disable-structure shown="Disabled" {
          frame Disabled {
            n445 = local write "Raster scan"(FALSE ("Raster scan")) -> ()
            n446 = property on="Reset data stream" class="Bool (strict)"("Val(Sgnl)"=TRUE) -> ()  [unwired: 2 in, 2 out]
          }
          frame Enabled {
          }
        }
        n447 = local read "Data update period (s/set)"() -> (w463:dbl)
        n448 = local read "Time per step (ms)"() -> (w460:dbl)
        n449 = local read "Trap position (V)"() -> (w445:cluster{"X":dbl, "Y":dbl})
        n450 = local read "Fixed X"() -> (w483:dbl)
        n451 = local read "Fixed Y"() -> (w484:dbl)
        n452 = Unbundle(w445) -> ("X"=w443:dbl, "Y"=w444:dbl)
        n453 = local read "Scan steps (mirror)"() -> (w472:u64)
        n454 = Multiply(x=w463, y=1000.0) -> (x*y=w461:dbl)
        n455 = local read "Stop raster"() -> (w479:bool)
        n456 = local read "Stop saving"() -> (w480:bool)
        n457 = Select(t=w483, s="Pulling direction", f=w484) -> (s? t:f=w491:dbl)
        n458 = Divide(x=w460, y=w461) -> (x/y=w459:dbl)
        n459 = Quotient & Remainder(x=w458, y=w459) -> (x-y*floor(x/y)=w457:dbl)  [unwired: 1 out]
        n460 = Not(x=w479) -> (.not. x?=w478:bool)
        n461 = Not(x=w480) -> (.not. x?=w477:bool)
        n462 = Multiply(x=u64 2, y=w472) -> (x*y=w468:u64)
        n463 = Select(t=w444, s="Pulling direction", f=w443) -> (s? t:f=w467:dbl)
        n464 = Equal To 0?(x=w457) -> (x = 0?=w456:bool)
        n465 = Less?(x=w446, y=w468) -> (x < y?=w469:bool)
        n466 = Compound Arithmetic op=AND(w469, w478, w477, w456) -> (w470:bool)
        n467 = Not(x=w469) -> (.not. x?=w452:bool)
        n468 = feedback #11() -> (w475:dbl)  [unwired: 1 in]
        n469 = case shown="True" w470 {
          tunnel: w491 -> [_ w527]
          tunnel: w467 -> [_ w509]
          tunnel: w490 -> [w504 w526]
          tunnel: w489 -> [w503 w525]
          tunnel: [w504 w524] -> w474
          tunnel: [w503 w523] -> w473
          tunnel: [w500 w512] -> w476
          tunnel: w446 -> [w501 w507]
          tunnel: w475 -> [w500 w506]
          tunnel: w466 -> [w502 w511]
          tunnel: [w502 w511] -> w465
          tunnel: [w501 w510] -> w450
          frame False {
          }
          frame True {
            # "Go forward or backward?"
            n470 = local read "Scan increment (V)"() -> (w505:dbl)
            n471 = local read "Scan steps (mirror)"() -> (w516:u64)
            n472 = Multiply(x=w505, y=w507) -> (x*y=w508:dbl)
            n473 = Less?(x=w507, y=w516) -> (x < y?=w515:bool)
            n474 = Add(x=w509, y=w508) -> (x+y=w518:dbl)
            n475 = Subtract(x=w506, y=w505) -> (x-y=w517:dbl)
            n476 = Select(t=w518, s=w515, f=w517) -> (s? t:f=w512:dbl)
            n477 = local read "Pulling direction"() -> (w514:bool)
            n478 = Build Array(w512, w527) -> (w521:dbl[])
            n479 = Build Array(w527, w512) -> (w520:dbl[])
            n480 = Select(t=w521, s=w514, f=w520) -> (s? t:f=w519:dbl[])
            n481 = call-poly <vilib>:"DAQmx Write.vi"("task/channels in"=w526, "auto start"=TRUE, "data"=w519, "error in"=w525) -> ("task out"=w524:refnum<k21>, "error out"=w523:errorcluster)  [unwired: 9 in, 1 out]
            n482 = Increment(x=w507) -> (x+1=w510:i32)
            "Raster scanning..." <- TRUE ("Raster scanning...")
          }
        }
        n483 = feedback-in #11(w476) -> ()
        n484 = case shown="True" w452 {
          tunnel: w455 -> [w497 w499]
          tunnel: [w497 w498] -> w454
          frame False {
          }
          frame True {
            n485 = Increment(x=w499) -> (x+1=w498:i32)
          }
        }
        n486 = local read "# scans"() -> (w453:i32)
        n487 = local read "Stop saving"() -> (w482:bool)
        n488 = Greater Or Equal?(x=w454, y=w453) -> (x >= y?=w447:bool)
        n489 = Not(x=w447) -> (.not. x?=w448:bool)
        n490 = And(x=w452, y=w448) -> (x .and. y?=w451:bool)
        n491 = Compound Arithmetic op=OR(w447, "Stop raster", w482) -> (w485:bool)
        n492 = case shown="True" w485 {
          frame False {
          }
          frame True {
            n493 = flat-sequence {
              frame #0 {
                n494 = Wait (ms)(milliseconds to wait=u32 300) -> ()  [unwired: 1 out]
              }
              frame #1 {
                n495 = property on="Trap delta (nm)" class="DigNum (strict)"("Val(Sgnl)"="Trap delta\nafter (nm)") -> ()  [unwired: 2 in, 2 out]
              }
            }
          }
        }
        n496 = And(x="Flow on\nafter raster?", y=w485) -> (x .and. y?=w486:bool)
        n497 = case shown="True" w486 {
          frame False {
          }
          frame True {
            n498 = property on="Inject Sample" class="Bool (strict)"("Val(Sgnl)"=TRUE ("Value (Signaling)")) -> ()  [unwired: 2 in, 2 out]
          }
        }
        n499 = case shown="True" w451 {
          tunnel: w450 -> [w495 _]
          tunnel: [w495 0] -> w449
          frame False {
          }
          frame True {
          }
        }
        n500 = Not(x=w485) -> (.not. x?=w488:bool)
        n501 = local write "Raster scanning..."(w488) -> ()
        n502 = Increment(x=w458) -> (x+1=w464:i32)
      }
    }
    n503 = And(x="Save scans", y=w121) -> (x .and. y?=w130:bool)
    n504 = feedback-in #8(w115) -> ()
    n505 = feedback-in #9(w112) -> ()
    n506 = feedback-in #10(w119) -> ()
    n507 = local read "Stop"() -> (w430:bool)
  }
  n508 = local write "Progress"(u8 0 ("Progress")) -> ()
  n509 = local write "Calibrating"(FALSE ("Calibrating")) -> ()
  n510 = call "InitializeChamberImage.vi"() -> ("error out"=w101:errorcluster, "IMAQ Session Out"=w102:refnum<k11>, "Display Out"=w103:T7, "Acquired Image"=w9:T7)  [unwired: 8 in]
  n511 = node-c288(i64 10 ("Period"), 2 ("Processor")) -> (w15:T12)  [unwired: 2 in]
  n512 = timed-loop {
    tunnel: w103 -> [w873]
    tunnel: w102 -> [w872]
    tunnel: w101 -> [w871]
    tunnel: [w869] -> w100
    tunnel: [w868] -> w99
    timing: w15 -> [_]
    timing-out: [_] -> w14
    i -> [w870]
    stop <- w864 continue-if-true
    n513 = node-c288() -> ()  [unwired: 1 in, 1 out]
    n514 = call <vilib>:"IMAQ Copy Acquired Buffer.vi"("IMAQ Session In"=w872, "Image In"=w873, "Buffer Number"=w870, "error in (no error)"=w871) -> ("IMAQ Session Out"=w869:refnum<k11>, "Image Out"=→"Chamber":T7, "error out"=w868:errorcluster)  [unwired: 7 in, 2 out]
    "Video Error" <- w868
    n515 = local read "Stop"() -> (w866:bool)
    n516 = Unbundle By Name(w868) -> ("status"=w867:bool)
    n517 = Not Or(1:w866, 2:w867) -> (0:w864:bool)
    "Continue to display?" <- w864
    n518 = node-c288() -> ()  [unwired: 1 in, 1 out]
  }
  n519 = node-c288(w14) -> ()  [unwired: 1 out]
  n520 = call <vilib>:"IMAQ Close.vi"("error in (no error)"=w99, "IMAQ Session In"=w100) -> ("error out"=w107:errorcluster)  [unwired: 9 in]
  n521 = call "IMAQ Dispose"("error in (no error)"=w107) -> ("error out"=w106:errorcluster)  [unwired: 5 in]
  n522 = call-poly "VISA Configure Serial Port"("VISA resource name"=refnum<visa-resource-name> "COM3") -> ("VISA resource name out"=w21:refnum<visa-resource-name>, "error out"=w20:errorcluster)  [unwired: 13 in]
  n523 = call "IMAQ Dispose"("Image"=w9, "error in (no error)"=w106) -> ("error out"=w105:errorcluster)  [unwired: 4 in]
  n524 = node-c288(i64 100 ("Period"), 2 ("Processor")) -> (w23:T12)  [unwired: 2 in]
  n525 = call <vilib>:"Simple Error Handler.vi"("error in (no error)"=w105) -> ()  [unwired: 4 in, 5 out]
  n526 = timed-loop {
    timing: w23 -> [_]
    timing-out: [_] -> w22
    tunnel: w21 -> [w876]
    tunnel: w20 -> [w878]
    tunnel: [w876] -> w19
    stop <- w877 stop-if-true
    n527 = node-c288() -> ()  [unwired: 1 in, 1 out]
    n528 = event shown="[6] \"Set Current Pos to (0,0,0)\": Value Change" {
      selector: _ -> [_ _ _ _ _ _ _ _ _ _ _ _]
      dyn-events: _ -> [_ _ _ _ _ _ _ _ _ _ _ _]
      timeout: _ -> [_ _ _ _ _ _ _ _ _ _ _ _]
      tunnel: w876 -> [w885 w924 w944 w961 w978 w997 w1020 w1030 _ _ _ _]
      tunnel: w878 -> [w884 w923 w943 w960 w977 w996 w1019 w1029 _ _ _ _]
      tunnel: [_ _ _ _ _ _ _ _ _ _ _ w1083] -> w877
      event "Got DNA bead": Value Change {
        n529 = event-data() -> ()  [unwired: 1 in, 5 out]
        n530 = flat-sequence {
          tunnel: w885 -> [w889]
          tunnel: w884 -> [w887]
          tunnel: [w904] -> w883
          tunnel: w883 -> [w907]
          tunnel: [w907] -> w882
          tunnel: w882 -> [w909]
          tunnel: [w909] -> w881
          tunnel: w881 -> [w913]
          tunnel: [w913] -> w880
          tunnel: w880 -> [w915]
          tunnel: [w915] -> w879
          tunnel: w879 -> [w917]
          frame #0 {
            n531 = local read "Saved stage positions"() -> (w890:dbl[][])
            n532 = disable-structure shown="Disabled" {
              frame Disabled {
                n533 = property on="Inject Pump 2" class="Bool (strict)"("Val(Sgnl)"=FALSE ("Inject Pump 2")) -> ()  [unwired: 2 in, 2 out]
              }
              frame Enabled {
              }
            }
            n534 = property on="Inject Sample" class="Bool (strict)"("Val(Sgnl)"=TRUE ("Value (Signaling)")) -> ()  [unwired: 2 in, 2 out]
            n535 = local write "Stage moving"(TRUE ("Stage moving")) -> ()
            n536 = property on="Trap delta (nm)" class="DigNum (strict)"("Val(Sgnl)"="Cal @ Delta (nm)") -> ()  [unwired: 2 in, 2 out]
            n537 = call "move to saved stage position.vi"("error in"=w887, "Stage VISA resource name in"=w889, "Position"="Cal stage position", "Saved Stage Positions"=w890) -> ()  [unwired: 2 out]
          }
          frame #1 {
            n538 = local write "Stage moving"(FALSE ("Stage moving")) -> ()
            n539 = property on="Inject Sample" class="Bool (strict)"("Val(Sgnl)"=FALSE ("Value (Signaling)")) -> ()  [unwired: 2 in, 2 out]
            n540 = call <vilib>:"Beep.vi"() -> ()  [unwired: 12 in]
          }
          frame #2 {
            n541 = Wait (ms)(milliseconds to wait=u32 1000) -> ()  [unwired: 1 out]
          }
          frame #3 {
            n542 = property on="Save cal" class="Bool (strict)"("Val(Sgnl)"=TRUE ("Value (Signaling)")) -> ()  [unwired: 2 in, 2 out]
          }
          frame #4 {
            n543 = Wait (ms)(milliseconds to wait=u32 2000) -> ()  [unwired: 1 out]
          }
          frame #5 {
            n544 = while {
              stop <- w900 stop-if-true
              n545 = local read "Saving"() -> (w901:bool)
              n546 = Not(x=w901) -> (.not. x?=w900:bool)
              n547 = Wait (ms)(milliseconds to wait=u32 100) -> ()  [unwired: 1 out]
            }
          }
          frame #6 {
            n548 = Wait (ms)(milliseconds to wait=u32 2000) -> ()  [unwired: 1 out]
            n549 = property on="Trap delta (nm)" class="DigNum (strict)"("Val(Sgnl)"="Offset @ Delta (nm)") -> ()  [unwired: 2 in, 2 out]
          }
          frame #7 {
            # "Only continue if there is no buffer\noverflow error"
            n550 = local read "Buffer Overflow"() -> (w905:bool)
            n551 = Not(x=w905) -> (.not. x?=w904:bool)
            n552 = case shown="True" w904 {
              frame False {
              }
              frame True {
                n553 = property on="Raster scan" class="Bool (strict)"("Val(Sgnl)"=TRUE ("Value (Signaling)")) -> ()  [unwired: 2 in, 2 out]
              }
            }
          }
          frame #8 {
            n554 = case shown="True" w907 {
              frame False {
              }
              frame True {
                n555 = Wait (ms)(milliseconds to wait=u32 2000) -> ()  [unwired: 1 out]
              }
            }
          }
          frame #9 {
            n556 = case shown="True" w909 {
              frame False {
              }
              frame True {
                n557 = while {
                  stop <- w911 stop-if-true
                  n558 = local read "Saving"() -> (w912:bool)
                  n559 = Not(x=w912) -> (.not. x?=w911:bool)
                  n560 = Wait (ms)(milliseconds to wait=u32 100) -> ()  [unwired: 1 out]
                }
              }
            }
          }
          frame #10 {
            n561 = case shown="True" w913 {
              frame False {
              }
              frame True {
                n562 = property on="Read Cal" class="Bool (strict)"("Val(Sgnl)"=TRUE ("Value (Signaling)")) -> ()  [unwired: 2 in, 2 out]
              }
            }
          }
          frame #11 {
            n563 = case shown="True" w915 {
              frame False {
              }
              frame True {
                n564 = Wait (ms)(milliseconds to wait=u32 1000) -> ()  [unwired: 1 out]
              }
            }
          }
          frame #12 {
            n565 = case shown="True" w917 {
              frame False {
              }
              frame True {
                n566 = property on="Fish" class="Bool (strict)"("Val(Sgnl)"=TRUE ("Value (Signaling)")) -> ()  [unwired: 2 in, 2 out]
                n567 = case shown="True" "Flow on\nwhile fish?" {
                  frame False {
                  }
                  frame True {
                    n568 = property on="Inject Sample" class="Bool (strict)"("Val(Sgnl)"=TRUE ("Value (Signaling)")) -> ()  [unwired: 2 in, 2 out]
                  }
                }
              }
            }
          }
        }
      }
      event "Dump beads": Value Change {
        n569 = event-data() -> ()  [unwired: 1 in, 5 out]
        n570 = flat-sequence {
          tunnel: w923 -> [w927]
          tunnel: w924 -> [w928]
          tunnel: [w928] -> w922
          tunnel: [w927] -> w921
          tunnel: w922 -> [w931]
          tunnel: w921 -> [w930]
          frame #0 {
            w925 = FALSE ("Fish")
            n571 = local read "Saving"() -> (w926:bool)
            n572 = local write "Pause dwell"(w925) -> ()
            n573 = local write "Force Feedback"(w925) -> ()
            n574 = local write "Dump beads"(w925) -> ()
            n575 = property on="Stop saving" class="Bool (strict)"("Val(Sgnl)"=w926) -> ()  [unwired: 2 in, 2 out]
            n576 = local write "Fish"(w925) -> ()
          }
          frame #1 {
            n577 = local read "Saved stage positions"() -> (w933:dbl[][])
            n578 = case shown="True" "Flow on\ndump?" {
              frame False {
              }
              frame True {
                n579 = property on="Inject Sample" class="Bool (strict)"("Val(Sgnl)"=TRUE ("Value (Signaling)")) -> ()  [unwired: 2 in, 2 out]
              }
            }
            n580 = local write "Stage moving"(TRUE ("Stage moving")) -> ()
            n581 = call "move to saved stage position.vi"("error in"=w930, "Stage VISA resource name in"=w931, "Position"=5, "Saved Stage Positions"=w933) -> ()  [unwired: 2 out]
          }
          frame #2 {
            n582 = local read "Shutter 1 (B)"() -> (w938:bool)
            n583 = local read "Shutter 2 (A)"() -> (w937:bool)
            n584 = call <vilib>:"Beep.vi"() -> ()  [unwired: 12 in]
            n585 = case shown="True" w938 {
              frame False {
              }
              frame True {
                n586 = property on="Shutter 1 (B)" class="Bool (strict)"("Val(Sgnl)"=FALSE ("Value (Signaling)")) -> ()  [unwired: 2 in, 2 out]
              }
            }
            n587 = case shown="True" w937 {
              frame False {
              }
              frame True {
                n588 = property on="Shutter 2 (A)" class="Bool (strict)"("Val(Sgnl)"=FALSE) -> ()  [unwired: 2 in, 2 out]
              }
            }
            n589 = local write "Stage moving"(FALSE ("Stage moving")) -> ()
            n590 = local write "Tether"(FALSE ("Tether")) -> ()
          }
          frame #3 {
            n591 = property on="Move Cap. 2 (ADig Top)" class="Bool (strict)"("Val(Sgnl)"=TRUE ("Value (Signaling)")) -> ()  [unwired: 2 in, 2 out]
          }
        }
      }
      event "Move Cap. 2 (ADig Top)": Value Change {
        n592 = event-data() -> ()  [unwired: 1 in, 5 out]
        n593 = flat-sequence {
          tunnel: w944 -> [w948]
          tunnel: w943 -> [w947]
          frame #0 {
            n594 = local read "Saved stage positions"() -> (w946:dbl[][])
            n595 = case shown="True" "Flow on\ncap 2?" {
              frame False {
              }
              frame True {
                n596 = property on="Inject Sample" class="Bool (strict)"("Val(Sgnl)"=TRUE ("Value (Signaling)")) -> ()  [unwired: 2 in, 2 out]
              }
            }
            n597 = local write "Move Cap. 2 (ADig Top)"(FALSE ("Move Cap. 2 (ADig Top)")) -> ()
            n598 = local write "Stage moving"(TRUE ("Stage moving")) -> ()
            n599 = call "move to saved stage position.vi"("error in"=w947, "Stage VISA resource name in"=w948, "Position"=2, "Saved Stage Positions"=w946) -> ()  [unwired: 2 out]
          }
          frame #1 {
            # "Make sure you don't reverse\nwhich is ON and OFF"
            n600 = local read "Cal @ Delta (nm)"() -> (w955:dbl)
            n601 = local write "Stage moving"(FALSE ("Stage moving")) -> ()
            n602 = call <vilib>:"Beep.vi"() -> ()  [unwired: 12 in]
            n603 = property on="Trap delta (nm)" class="DigNum (strict)"("Val(Sgnl)"=w955) -> ()  [unwired: 2 in, 2 out]
            n604 = disable-structure shown="Disabled" {
              frame Disabled {
                n605 = property on="Inject Pump 1" class="Bool (strict)"("Val(Sgnl)"=TRUE ("Inject Pump 2")) -> ()  [unwired: 2 in, 2 out]
              }
              frame Enabled {
              }
            }
            n606 = local read "Shutter 2 (A)"() -> (w954:bool)
            n607 = case shown="False" w954 {
              frame False {
                n608 = property on="Shutter 2 (A)" class="Bool (strict)"("Val(Sgnl)"=TRUE ("Value (Signaling)")) -> ()  [unwired: 2 in, 2 out]
              }
              frame True {
              }
            }
            n609 = property on="Inject Sample" class="Bool (strict)"("Val(Sgnl)"=FALSE ("Value (Signaling)")) -> ()  [unwired: 2 in, 2 out]
          }
        }
      }
      event "Got ADig bead": Value Change {
        n610 = event-data() -> ()  [unwired: 1 in, 5 out]
        n611 = flat-sequence {
          tunnel: w961 -> [w965]
          tunnel: w960 -> [w964]
          frame #0 {
            n612 = local read "Saved stage positions"() -> (w967:dbl[][])
            n613 = property on="Inject Pump 1" class="Bool (strict)"("Val(Sgnl)"=FALSE ("Inject Pump 2")) -> ()  [unwired: 2 in, 2 out]
            n614 = case shown="True" "Flow on\ncap 1?" {
              frame False {
              }
              frame True {
                n615 = property on="Inject Sample" class="Bool (strict)"("Val(Sgnl)"=TRUE ("Value (Signaling)")) -> ()  [unwired: 2 in, 2 out]
              }
            }
            n616 = local write "Stage moving"(TRUE ("Stage moving")) -> ()
            n617 = call "move to saved stage position.vi"("error in"=w964, "Stage VISA resource name in"=w965, "Position"=1, "Saved Stage Positions"=w967) -> ()  [unwired: 2 out]
          }
          frame #1 {
            n618 = local read "Shutter 1 (B)"() -> (w971:bool)
            n619 = disable-structure shown="Disabled" {
              frame Disabled {
                n620 = property on="Inject Pump 2" class="Bool (strict)"("Val(Sgnl)"=TRUE ("Inject Pump 2")) -> ()  [unwired: 2 in, 2 out]
              }
              frame Enabled {
              }
            }
            n621 = local write "Stage moving"(FALSE ("Stage moving")) -> ()
            n622 = case shown="False" w971 {
              frame False {
                n623 = property on="Shutter 1 (B)" class="Bool (strict)"("Val(Sgnl)"=TRUE ("Value (Signaling)")) -> ()  [unwired: 2 in, 2 out]
              }
              frame True {
              }
            }
            n624 = property on="Inject Sample" class="Bool (strict)"("Val(Sgnl)"=FALSE ("Value (Signaling)")) -> ()  [unwired: 2 in, 2 out]
            n625 = call <vilib>:"Beep.vi"() -> ()  [unwired: 12 in]
          }
        }
        n626 = local write "Got ADig bead"(FALSE ("Got ADig bead")) -> ()
      }
      event "Set Position 1", "Set Position 2", "Set Position 3", "Set Position 4", "Set Position 5": Value Change {
        n627 = event-data() -> ()  [unwired: 1 in, 5 out]
        n628 = Build Array("Set Position 1", "Set Position 2", "Set Position 3", "Set Position 4", "Set Position 5") -> (w990:bool[])
        n629 = Boolean Array To Number(Boolean array=w990) -> (number=w989:u32)
        n630 = call "Read Stage Position.vi"("error in"=w977, "VISA resource name in"=w978) -> ("Current Position"=w975:cluster{dbl, dbl, dbl}, "error out"=→"Stage error":errorcluster)  [unwired: 1 in, 1 out]
        n631 = Logarithm Base 2(1:w989) -> (0:w983:dbl)
        n632 = Cluster To Array(cluster=w975) -> (array=w985:dbl[])
        n633 = Increment(x=w983) -> (x+1=w986:dbl)
        n634 = Build Array (concatenate)(w986, w985) -> (w984:dbl[])
        n635 = Replace Array Subset(array="Saved stage positions", new element=w984, index (row)=w983) -> (w987:dbl[][])  [unwired: 1 in]
        n636 = local write "Saved stage positions"(w987) -> ()
      }
      event "Move to Position 2", "Move to Position 4", "Move to Position 3", "Move to Position 5", "Move to Position 1": Value Change {
        n637 = event-data() -> ()  [unwired: 1 in, 5 out]
        n638 = Build Array("Move to Position 1", "Move to Position 2", "Move to Position 3", "Move to Position 4", "Move to Position 5") -> (w1000:bool[])
        n639 = Boolean Array To Number(Boolean array=w1000) -> (number=w999:u32)
        n640 = Logarithm Base 2(1:w999) -> (0:w998:dbl)
        n641 = flat-sequence {
          tunnel: w998 -> [w1005]
          tunnel: w997 -> [w1004]
          tunnel: w996 -> [w1003]
          frame #0 {
            n642 = local read "Saved stage positions"() -> (w1006:dbl[][])
            n643 = Increment(x=w1005) -> (x+1=w1002:dbl)
            n644 = call "move to saved stage position.vi"("error in"=w1003, "Stage VISA resource name in"=w1004, "Position"=w1002, "Saved Stage Positions"=w1006) -> ()  [unwired: 2 out]
            "Stage moving" <- TRUE ("Stage moving")
          }
          frame #1 {
            n645 = call <vilib>:"Beep.vi"() -> ()  [unwired: 12 in]
            n646 = local write "Stage moving"(FALSE ("Stage moving")) -> ()
          }
        }
      }
      event "Set Current\nPos to (0,0,0)": Value Change {
        w1010 = ";" ("string")
        # "DH is \"Define Home\" -KW"
        n647 = event-data() -> ()  [unwired: 1 in, 5 out]
        n648 = local write "Set Current\nPos to (0,0,0)"(FALSE ("Set Current\nPos to (0,0,0)")) -> ()
        n649 = call-poly "VISA Configure Serial Port"("VISA resource name"=w1020, "baud rate (9600)"=u32 19200, "error in (no error)"=w1019) -> ("VISA resource name out"=w1014:refnum<visa-resource-name>, "error out"=w1013:errorcluster)  [unwired: 11 in]
        n650 = Concatenate Strings("1DH" ("string"), w1010, "2DH" ("string"), w1010, "3DH" ("string"), "\r") -> (w1012:string)
        n651 = VISA Write(VISA resource name=w1014, write buffer=w1012, error in (no error)=w1013) -> (error out=w1011:errorcluster)  [unwired: 2 out]
        n652 = local write "Stage error"(w1011) -> ()
      }
      event "Dip": Value Change {
        n653 = event-data() -> ()  [unwired: 1 in, 5 out]
        n654 = local write "Dip"(FALSE ("Dip")) -> ()
        n655 = flat-sequence {
          tunnel: w1030 -> [w1032]
          tunnel: w1029 -> [w1031]
          tunnel: [w1033] -> w1027
          tunnel: [w1032] -> w1025
          tunnel: [w1031] -> w1023
          tunnel: [w1041] -> w1028
          tunnel: w1027 -> [w1041]
          tunnel: [w1040] -> w1026
          tunnel: w1025 -> [w1040]
          tunnel: [w1039] -> w1024
          tunnel: w1023 -> [w1039]
          tunnel: w1028 -> [w1060]
          tunnel: w1026 -> [w1059]
          tunnel: w1024 -> [w1058]
          frame #0 {
            n656 = local read "Saved stage positions"() -> (w1033:dbl[][])
            n657 = local write "Stage moving"(TRUE) -> ()
            n658 = call "move to saved stage position.vi"("error in"=w1031, "Stage VISA resource name in"=w1032, "Position"="Dip position", "Saved Stage Positions"=w1033) -> ()  [unwired: 2 out]
          }
          frame #1 {
            n659 = node-c288() -> (w1038:T12)  [unwired: 4 in]
            n660 = timed-loop {
              timing: w1038 -> [_]
              timing-out: [_] -> w1037
              i -> [w1051]
              stop <- w1042 stop-if-true
              n661 = node-c288() -> ()  [unwired: 1 in, 1 out]
              n662 = Greater Or Equal?(x=w1051, y="Dip duration") -> (x >= y?=w1047:bool)
              n663 = local read "Dump beads"() -> (w1044:bool)
              n664 = Or(x=w1047, y="Cancel dwell") -> (x .or. y?=w1045:bool)
              n665 = Not(x="Pause dwell") -> (.not. x?=w1048:bool)
              n666 = node-c288() -> ()  [unwired: 1 in, 1 out]
              n667 = And(x=w1048, y=w1045) -> (x .and. y?=w1043:bool)
              n668 = Or(x=w1043, y=w1044) -> (x .or. y?=w1042:bool)
              "Dip time" <- w1051
            }
            n669 = local write "Stage moving"(FALSE ("Stage moving")) -> ()
            n670 = node-c288(w1037) -> ()  [unwired: 1 out]
          }
          frame #2 {
            n671 = local write "Cancel dwell"(FALSE ("Cancel dwell")) -> ()
            n672 = call "move to saved stage position.vi"("error in"=w1058, "Stage VISA resource name in"=w1059, "Position"="Return position", "Saved Stage Positions"=w1060) -> ()  [unwired: 2 out]
          }
          frame #3 {
            n673 = local write "Stage moving"(FALSE ("Stage moving")) -> ()
          }
        }
      }
      event "Force FB script": Value Change {
        n674 = event-data() -> ()  [unwired: 1 in, 5 out]
        n675 = flat-sequence {
          frame #0 {
            n676 = disable-structure shown="Disabled" {
              frame Disabled {
                n677 = local read "# Samples/channel"() -> (w1064:i32)
                n678 = local write "# Samples/channel (in)"(w1064) -> ()
              }
              frame Enabled {
              }
            }
            n679 = local write "Force FB script"(FALSE ("Force FB script")) -> ()
            n680 = property on="Trap delta (nm)" class="DigNum (strict)"("Val(Sgnl)"="Start trap delta (nm)") -> ()  [unwired: 2 in, 2 out]
          }
          frame #1 {
            n681 = Wait (ms)(milliseconds to wait=u32 500) -> ()  [unwired: 1 out]
          }
          frame #2 {
            n682 = property on="Set reading to\nsetpoint" class="Bool (strict)"("Val(Sgnl)"=TRUE ("Value (Signaling)")) -> ()  [unwired: 2 in, 2 out]
          }
          frame #3 {
            n683 = Wait (ms)(milliseconds to wait=u32 300) -> ()  [unwired: 1 out]
          }
          frame #4 {
            n684 = local write "Force Feedback"(TRUE ("Force Feedback")) -> ()
            n685 = property on="Tabs" class="TabCtl (strict)"("Val(Sgnl)"=T3."Force Feedback" ("Value (Signaling)")) -> ()  [unwired: 2 in, 2 out]
          }
          frame #5 {
            n686 = property on="Save Data" class="Bool (strict)"("Val(Sgnl)"=TRUE ("Value (Signaling)")) -> ()  [unwired: 2 in, 2 out]
          }
          frame #6 {
            n687 = Multiply(x="Wait before dip (s)", y=1000) -> (x*y=w1071:dbl)
            n688 = Wait (ms)(milliseconds to wait=w1071) -> ()  [unwired: 1 out]
          }
          frame #7 {
            n689 = case shown="True" "Start dipping after?" {
              selector: "Start dipping after?" -> [_ w1076]
              frame False {
              }
              frame True {
                n690 = property on="Dip" class="Bool (strict)"("Val(Sgnl)"=w1076) -> ()  [unwired: 2 in, 2 out]
              }
            }
            n691 = property on="Remove offsets" class="Bool (strict)"("Val(Sgnl)"=TRUE ("Value (Signaling)")) -> ()  [unwired: 2 in, 2 out]
          }
        }
      }
      event "Move 0": Value Change {
        n692 = event-data() -> ()  [unwired: 1 in, 5 out]
        n693 = local write "Move 0"(FALSE) -> ()
        n694 = call "HalfWavePlate.vi"("Degrees"="\"Degrees\" 0", "Motor"=0) -> ()  [unwired: 1 in]
      }
      event "Move 1": Value Change {
        n695 = event-data() -> ()  [unwired: 1 in, 5 out]
        n696 = local write "Move 1"(FALSE) -> ()
        n697 = call "HalfWavePlate.vi"("Degrees"="\"Degrees\" 1", "Motor"=1) -> ()  [unwired: 1 in]
      }
      event "Stop": Value Change {
        n698 = event-data() -> ()  [unwired: 1 in, 5 out]
        n699 = local read "Stop"() -> (w1083:bool)
      }
    }
    n700 = node-c288() -> ()  [unwired: 1 in, 1 out]
  }
  n701 = node-c288(2 ("Processor")) -> (w75:T12)  [unwired: 3 in]
  n702 = node-c288(2 ("Processor")) -> (w27:T12)  [unwired: 3 in]
  n703 = timed-loop {
    timing: w75 -> [_]
    timing-out: [_] -> w74
    stop <- w1086 stop-if-true
    n704 = node-c288() -> ()  [unwired: 1 in, 1 out]
    n705 = case shown="\"Current Saved Data\"" "Tab Control" {
      frame "Control" {
        n706 = case shown="True" "Start" {
          frame False {
          }
          frame True {
            w1099 = T15 3 items=["no dialog", "OK message", "continue or stop message", "OK message + warnings", "continue/stop + warnings"] ("type of dialog (OK msg:1)")
            n707 = call "InitializeAcquireFF.vi"("DAQ Rate"="DAQ Rate", "Averaging Number"="Averaging Number", "Sampling Rate"="Sampling Rate") -> ("error out"=w1093:errorcluster, "task out"=w1092:refnum<k21>, "Final Sampling Rate"=→"Final Sampling Rate":dbl)  [unwired: 4 in, 2 out]
            n708 = while {
              tunnel: [w1111] -> w1098
              tunnel: [w1110] -> w1091
              tunnel: "Averaging Number" -> [w1109]
              tunnel: w1093 -> [w1108]
              tunnel: w1092 -> [w1106]
              stop <- w1107 continue-if-true
              n709 = call "Acquire2_QPD.vi"("task/channels in"=w1106, "Save Data?"=FALSE ("Take Data?"), "Averaging Number"=w1109, "error in"=w1108) -> ("PSD 1"=→"PSD 1":cluster{dbl[], dbl[]}, "PSD 1 Sum"=→"PSD 1 Sum":dbl, "PSD 2"=→"PSD 2":cluster{dbl[], dbl[]}, "PSD 2 Sum"=→"PSD 2 Sum":dbl, "task out"=w1111:refnum<k21>, "error out"=w1110:errorcluster)  [unwired: 14 in, 4 out]
              n710 = local read "Start"() -> (w1107:bool)
            }
            n711 = call <vilib>:"DAQmx Clear Task.vi"("task in"=w1098, "error in"=w1091) -> ("error out"=w1100:errorcluster)  [unwired: 13 in]
            n712 = call <vilib>:"Simple Error Handler.vi"("type of dialog (OK msg:1)"=w1099, "error in (no error)"=w1100) -> ()  [unwired: 3 in, 5 out]
          }
        }
      }
      frame "Current Saved Data" {
      }
      frame "Data Acquisition" {
      }
      frame "Raw QPD Data" {
      }
    }
    n713 = local read "Stop"() -> (w1086:bool)
    n714 = node-c288() -> ()  [unwired: 1 in, 1 out]
  }
  n715 = call-poly <vilib>:"DAQmx Create Virtual Channel.vi"("lines"=w92) -> ("task out"=w91:refnum<k21>)  [unwired: 13 in, 1 out]
  n716 = call-poly <vilib>:"DAQmx Create Virtual Channel.vi"("lines"=w95) -> ("task out"=w94:refnum<k21>)  [unwired: 13 in, 1 out]
  n717 = timed-loop {
    timing: w27 -> [_]
    timing-out: [_] -> w26
    stop <- w1112 stop-if-true
    n718 = node-c288() -> ()  [unwired: 1 in, 1 out]
    n719 = event shown="[0] \"Pause Mouse/Mirror Connection\": Value Change" {
      selector: _ -> [_ _]
      dyn-events: _ -> [_ _]
      timeout: _ -> [_ _]
      tunnel: [w1205 _] -> w1113
      tunnel: [_ w1206] -> w1112
      event "Pause Mouse/Mirror Connection": Value Change {
        n720 = event-data() -> ("NewVal"=w1205:bool)  [unwired: 1 in]
      }
      event "Stop": Value Change {
        n721 = event-data() -> ("NewVal"=w1206:bool)  [unwired: 1 in]
      }
    }
    n722 = case shown="True" w1113 {
      frame False {
      }
      frame True {
        n723 = call "InitializeMouseControl.vi"() -> ("error out 2"=w1122:errorcluster, "task out"=w1123:refnum<k21>, "error out"=w1125:errorcluster, "device ID"=w1124:refnum<k1>)  [unwired: 8 in]
        n724 = while {
          tunnel: w1125 -> [w1137]
          tunnel: w1124 -> [w1136]
          tunnel: w1123 -> [w1135]
          tunnel: w1122 -> [w1134]
          tunnel: [w1133] -> w1120
          tunnel: [w1132] -> w1119
          tunnel: [w1131] -> w1116
          tunnel: [w1130] -> w1117
          stop <- w1129 stop-if-true
          n725 = case shown="True" "Use Mouse to Move Trap?" {
            tunnel: w1136 -> [w1144 w1167]
            tunnel: w1137 -> [w1143 w1166]
            tunnel: w1135 -> [w1142 w1165]
            tunnel: w1134 -> [w1141 w1164]
            tunnel: [w1144 w1163] -> w1131
            tunnel: [w1143 w1162] -> w1130
            tunnel: [w1142 w1161] -> w1133
            tunnel: [w1141 w1160] -> w1132
            frame False {
              (unwired) FALSE ("button 1")
            }
            frame True {
              w1155 = 0.0 ("y")
              w1157 = 10
              n726 = local read "Deflection"() -> (w1168:T4)
              n727 = call-poly <vilib>:"Acquire Input Data.vi"("device ID"=w1167, "error in (no error)"=w1166) -> ("device ID"=w1163:refnum<k1>, "button info"=w1181:T16, "error out"=w1162:errorcluster)  [unwired: 14 in, 1 out]
              n728 = Unbundle By Name(w1168) -> ("Horizontal"=w1170:i32, "Vertical"=w1169:i32)
              n729 = local read "Saved voltage"() -> (w1146:cluster{dbl, dbl})
              n730 = Divide(x=w1170, y=30) -> (x/y=w1173:dbl)
              n731 = Divide(x=w1169, y=-20) -> (x/y=w1174:dbl)
              n732 = Unbundle By Name(w1181) -> ("button 1"=w1159:bool, "button 2"=w1175:bool)
              n733 = Bundle(w1173, w1174) -> (w1151:cluster{dbl, dbl})  [unwired: 1 in]
              n734 = local write "Reference Voltage"(w1151) -> ()
              n735 = Add(x=w1151, y=w1146) -> (x+y=w1179:cluster{dbl, dbl})
              n736 = case shown="True" w1159 {
                frame False {
                  n737 = stacked-sequence {
                    frame #0 {
                      n738 = local write "CoordinatesMousePressed"(T4 {"Horizontal"=0, "Vertical"=0} ("Coords when pressed")) -> ()
                      n739 = local write "Deflection"(T4 {"Horizontal"=0, "Vertical"=0} ("deflaction")) -> ()
                    }
                  }
                }
                frame True {
                  n740 = local read "CoordinatesMousePressed"() -> (w1204:T4)
                  n741 = local read "Real Coordinates"() -> (w1203:cluster{"Horizontal":i32, "Vertical":i32})
                  n742 = Subtract(x=w1203, y=w1204) -> (x-y=w1202:T4)
                  n743 = local write "Deflection"(w1202) -> ()
                }
              }
              n744 = Unbundle(w1179) -> (w1156:dbl, w1147:dbl)
              n745 = case shown="True" w1175 {
                frame False {
                }
                frame True {
                  n746 = local read "Reference Voltage"() -> (w1185:cluster{dbl, dbl})
                  n747 = local read "Saved voltage"() -> (w1183:cluster{dbl, dbl})
                  n748 = Add(x=w1185, y=w1183) -> (x+y=→"Saved voltage":cluster{dbl, dbl})
                  n749 = local read "Real Coordinates"() -> (w1184:cluster{"Horizontal":i32, "Vertical":i32})
                  n750 = local write "CoordinatesMousePressed"(w1184) -> ()
                }
              }
              n751 = Less?(x=w1156, y=w1157) -> (x < y?=w1154:bool)
              n752 = Greater?(x=w1156, y=w1155) -> (0:w1153:bool)
              n753 = Greater?(x=w1147, y=w1155) -> (0:w1149:bool)
              n754 = Less?(x=w1147, y=w1157) -> (x < y?=w1150:bool)
              n755 = And(x=w1149, y=w1150) -> (x .and. y?=w1148:bool)
              n756 = And(x=w1154, y=w1153) -> (x .and. y?=w1152:bool)
              n757 = case shown="False" w1148 {
                tunnel: [w1195 w1199] -> w1158
                tunnel: w1147 -> [w1193 w1199]
                frame False {
                  n758 = Greater?(x=w1193, y=10.0) -> (0:w1196:bool)
                  n759 = case shown="True" w1196 {
                    tunnel: [0.0 10.0] -> w1195
                    frame False {
                    }
                    frame True {
                    }
                  }
                }
                frame True {
                }
              }
              n760 = case shown="False" w1152 {
                tunnel: w1156 -> [w1187 w1192]
                tunnel: [w1188 w1192] -> w1180
                frame False {
                  n761 = Greater?(x=w1187, y=10.0) -> (0:w1189:bool)
                  n762 = case shown="True" w1189 {
                    tunnel: [0.0 10.0] -> w1188
                    frame False {
                    }
                    frame True {
                    }
                  }
                }
                frame True {
                }
              }
              n763 = Bundle(w1180, w1158) -> (w1145:cluster{dbl, dbl})  [unwired: 1 in]
              n764 = Cluster To Array(cluster=w1145) -> (array=w1176:dbl[])
              n765 = call-poly <vilib>:"DAQmx Write.vi"("task/channels in"=w1165, "data"=w1176, "error in"=w1164) -> ("task out"=w1178:refnum<k21>, "error out"=w1177:errorcluster)  [unwired: 10 in, 1 out]
              n766 = call <vilib>:"DAQmx Is Task Done.vi"("task/channels in"=w1178, "error in"=w1177) -> ("task out"=w1161:refnum<k21>, "error out"=w1160:errorcluster)  [unwired: 11 in, 1 out]
            }
          }
          n767 = event shown="[0] \"Pane\": Mouse Move" {
            selector: _ -> [_ _ _]
            dyn-events: _ -> [_ _ _]
            timeout: _ -> [_ _ _]
            event Mouse Move {
              n768 = event-data() -> ("Coords"=w1139:T4)  [unwired: 1 in]
              n769 = local write "Real Coordinates"(w1139) -> ()
            }
            event Mouse Down {
              n770 = event-data() -> ("Coords"=w1140:T4)  [unwired: 1 in]
              n771 = local write "CoordinatesMousePressed"(w1140) -> ()
            }
            event "Pause Mouse/Mirror Connection": Value Change {
              n772 = event-data() -> ()  [unwired: 1 in, 3 out]
            }
          }
          n773 = local read "Stop"() -> (w1126:bool)
          n774 = Not(x="Pause Mouse/Mirror Connection") -> (.not. x?=w1127:bool)
          n775 = Or(x=w1127, y=w1126) -> (x .or. y?=w1129:bool)
        }
        n776 = call <vilib>:"DAQmx Clear Task.vi"("task in"=w1120, "error in"=w1119) -> ("error out"=w1121:errorcluster)  [unwired: 13 in]
        n777 = call <vilib>:"Simple Error Handler.vi"("error in (no error)"=w1121) -> ()  [unwired: 4 in, 5 out]
        n778 = call-poly <vilib>:"Close Input Device.vi"("error in (no error)"=w1117, "device ID"=w1116) -> ("error out"=w1118:errorcluster)  [unwired: 8 in]
        n779 = call <vilib>:"Simple Error Handler.vi"("error in (no error)"=w1118) -> ()  [unwired: 4 in, 5 out]
      }
    }
    n780 = node-c288() -> ()  [unwired: 1 in, 1 out]
  }
  n781 = node-c288(i64 100 ("Period")) -> (w89:T12)  [unwired: 3 in]
  n782 = timed-loop {
    tunnel: w91 -> [w1209]
    tunnel: [w1208] -> w90
    tunnel: w94 -> [w1211]
    tunnel: [w1210] -> w93
    timing: w89 -> [_]
    timing-out: [_] -> w88
    stop <- w1207 stop-if-true
    n783 = node-c288() -> ()  [unwired: 1 in, 1 out]
    n784 = event shown="[1] \"Shutter 2 (A)\": Value Change" {
      selector: _ -> [_ _ _]
      dyn-events: _ -> [_ _ _]
      timeout: _ -> [_ _ _]
      tunnel: w1211 -> [w1215 _ _]
      tunnel: [w1214 _ _] -> w1210
      tunnel: w1209 -> [_ w1235 _]
      tunnel: [_ w1233 _] -> w1208
      tunnel: [_ _ w1252] -> w1207
      event "Shutter 1 (B)": Value Change {
        n785 = event-data() -> ()  [unwired: 1 in, 1 out]
        n786 = flat-sequence {
          tunnel: [w1221] -> w1218
          tunnel: w1215 -> [w1220]
          tunnel: [w1225] -> w1217
          tunnel: [w1228] -> w1216
          tunnel: w1218 -> [w1223]
          tunnel: w1217 -> [w1232]
          tunnel: w1216 -> [w1230]
          tunnel: [w1229] -> w1214
          frame #0 {
            n787 = call-poly <vilib>:"DAQmx Write.vi"("task/channels in"=w1220, "data"=FALSE) -> ("task out"=w1221:refnum<k21>)  [unwired: 11 in, 2 out]
            n788 = Wait (ms)(milliseconds to wait=100) -> ()  [unwired: 1 out]
          }
          frame #1 {
            n789 = Or(x="Shutter 1 (B)", y=TRUE) -> (x .or. y?=w1225:bool)
            n790 = call-poly <vilib>:"DAQmx Write.vi"("task/channels in"=w1223, "data"=w1225) -> ("task out"=w1228:refnum<k21>)  [unwired: 11 in, 2 out]
            n791 = Wait (ms)(milliseconds to wait=100) -> ()  [unwired: 1 out]
          }
          frame #2 {
            n792 = Not(x=w1232) -> (.not. x?=w1231:bool)
            n793 = call-poly <vilib>:"DAQmx Write.vi"("task/channels in"=w1230, "data"=w1231) -> ("task out"=w1229:refnum<k21>)  [unwired: 11 in, 2 out]
          }
        }
      }
      event "Shutter 2 (A)": Value Change {
        n794 = event-data() -> ()  [unwired: 1 in, 1 out]
        n795 = flat-sequence {
          tunnel: w1235 -> [w1240]
          tunnel: [w1239] -> w1234
          tunnel: [w1244] -> w1237
          tunnel: [w1247] -> w1236
          tunnel: w1234 -> [w1242]
          tunnel: w1237 -> [w1251]
          tunnel: w1236 -> [w1249]
          tunnel: [w1248] -> w1233
          frame #0 {
            n796 = call-poly <vilib>:"DAQmx Write.vi"("task/channels in"=w1240, "data"=FALSE) -> ("task out"=w1239:refnum<k21>)  [unwired: 11 in, 2 out]
            n797 = Wait (ms)(milliseconds to wait=100) -> ()  [unwired: 1 out]
          }
          frame #1 {
            n798 = Or(x="Shutter 2 (A)", y=TRUE) -> (x .or. y?=w1244:bool)
            n799 = call-poly <vilib>:"DAQmx Write.vi"("task/channels in"=w1242, "data"=w1244) -> ("task out"=w1247:refnum<k21>)  [unwired: 11 in, 2 out]
            n800 = Wait (ms)(milliseconds to wait=100) -> ()  [unwired: 1 out]
          }
          frame #2 {
            n801 = Not(x=w1251) -> (.not. x?=w1250:bool)
            n802 = call-poly <vilib>:"DAQmx Write.vi"("task/channels in"=w1249, "data"=w1250) -> ("task out"=w1248:refnum<k21>)  [unwired: 11 in, 2 out]
          }
        }
      }
      event "Stop": Value Change {
        n803 = event-data() -> ("NewVal"=w1252:bool)  [unwired: 1 in, 5 out]
      }
    }
    n804 = node-c288() -> ()  [unwired: 1 in, 1 out]
  }
  n805 = node-c288(w88) -> ()  [unwired: 1 out]
  n806 = node-c288(w74) -> ()  [unwired: 1 out]
  n807 = call <vilib>:"DAQmx Clear Task.vi"("task in"=w90) -> ()  [unwired: 14 in, 1 out]
  n808 = call <vilib>:"DAQmx Clear Task.vi"("task in"=w93) -> ()  [unwired: 14 in, 1 out]
  n809 = node-c288(w26) -> ()  [unwired: 1 out]
  n810 = node-c288(w22) -> ()  [unwired: 1 out]
  n811 = local write "Tether"(FALSE ("Tether")) -> ()
  n812 = local read "Path"() -> (w81:path)
  n813 = node-c288(i64 1 ("Period"), 2 ("Processor")) -> (w87:T12)  [unwired: 2 in]
  n814 = VISA Close(VISA resource name=w19) -> (error out=w104:errorcluster)  [unwired: 1 in]
  n815 = timed-loop {
    timing: w87 -> [_]
    timing-out: [_] -> w86
    tunnel: w81 -> [w1254]
    stop <- w1253 stop-if-true
    n816 = node-c288() -> ()  [unwired: 1 in, 1 out]
    n817 = event shown="[1] \"Read Cal\": Value Change" {
      selector: _ -> [_ _ _ _ _ _ _ _ _]
      dyn-events: _ -> [_ _ _ _ _ _ _ _ _]
      timeout: _ -> [_ _ _ _ _ _ _ _ _]
      tunnel: w1254 -> [_ w1258 _ _ _ _ _ _ _]
      tunnel: [_ _ w1278 _ _ _ _ _ _] -> w1253
      event Timeout {
        n818 = event-data() -> ()  [unwired: 1 in, 2 out]
      }
      event "Read Cal": Value Change {
        n819 = event-data() -> ()  [unwired: 1 in, 6 out]
        n820 = Path To String(path=w1258) -> (string=w1257:string)
        n821 = Format Date/Time String(time format string (%c)="%y%m%d") -> (date/time string=w1259:string)  [unwired: 2 in]
        n822 = Concatenate Strings(w1257, "\\" ("string"), w1259, "\\" ("string"), "current.cal") -> (w1277:string)
        n823 = String To Path(string=w1277) -> (path=w1276:path)
        n824 = Open/Create/Replace File(file path (use dialog)=w1276, operation (0:open)=T9."open", access (0:read/write)=enum16{"read/write", "read-only", "write-only"}."read-only") -> (refnum out=w1272:refnum<file>, error out=w1273:errorcluster)  [unwired: 3 in, 1 out]
        n825 = Deny Access(4:w1273, 7:w1272) -> (0:w1271:errorcluster, 3:w1270:refnum<file>)  [unwired: 1 in]
        n826 = Read from Binary File(5:0.0, 8:w1271, 9:T10."big-endian, network order" ("byte order (0:big-endian, network order)"), 10:12 ("count"), 11:w1270) -> (0:w1266:errorcluster, 2:w1264:dbl[], 3:w1267:refnum<file>)  [unwired: 1 in, 1 out]
        n827 = Array To Cluster(array=w1264) -> (cluster=→"Cal values":T17)
        n828 = Close File(refnum=w1267, error in=w1266) -> ()  [unwired: 2 out]
        n829 = local write "Read Cal"(FALSE ("Read Cal")) -> ()
      }
      event "Stop": Value Change {
        n830 = event-data() -> ("NewVal"=w1278:bool)  [unwired: 1 in, 5 out]
      }
      event "Trap position (V)": Value Change {
        # "Need to rotate so X and Y don't get mixed up."
        n831 = event-data() -> ()  [unwired: 1 in, 6 out]
        n832 = local read "Mirror task"() -> (w1279:refnum<k21>)
        n833 = Cluster To Array(cluster="Trap position (V)") -> (array=w1282:dbl[])
        n834 = Rotate 1D Array(1:w1282, 2:1 ("n")) -> (0:w1280:dbl[])
        n835 = call-poly <vilib>:"DAQmx Write.vi"("task/channels in"=w1279, "data"=w1280) -> ("task out"=w1285:refnum<k21>, "error out"=w1284:errorcluster)  [unwired: 11 in, 1 out]
        n836 = call <vilib>:"DAQmx Stop Task.vi"("task/channels in"=w1285, "error in"=w1284) -> ("error out"=w1283:errorcluster)  [unwired: 12 in, 1 out]
        n837 = call <vilib>:"Simple Error Handler.vi"("error in (no error)"=w1283) -> ()  [unwired: 4 in, 5 out]
      }
      event "Trap delta (nm)": Value Change {
        n838 = event-data() -> ()  [unwired: 1 in, 6 out]
        n839 = local read "Pulling direction"() -> (w1287:bool)
        n840 = local read "Conv Y (nm/V)"() -> (w1288:dbl)
        n841 = local read "Conv X (nm/V)"() -> (w1289:dbl)
        n842 = Select(t=w1288, s=w1287, f=w1289) -> (s? t:f=w1290:dbl)
        n843 = local read "Fixed Y"() -> (w1296:dbl)
        n844 = Divide(x="Trap delta (nm)", y=w1290) -> (x/y=w1291:dbl)
        n845 = local read "Fixed X"() -> (w1295:dbl)
        n846 = Select(t=w1296, s=w1287, f=w1295) -> (s? t:f=w1294:dbl)
        n847 = Add(x=w1291, y=w1294) -> (x+y=w1292:dbl)
        n848 = case shown="False" w1287 {
          tunnel: w1292 -> [w1297 w1298]
          frame False {
            n849 = property on="X" class="DigNum (strict)"("Val(Sgnl)"=w1297) -> ()  [unwired: 2 in, 2 out]
          }
          frame True {
            n850 = property on="Y" class="DigNum (strict)"("Val(Sgnl)"=w1298) -> ()  [unwired: 2 in, 2 out]
          }
        }
      }
      event "Fish": Value Change {
        n851 = event-data() -> ()  [unwired: 1 in, 6 out]
        n852 = local read "Fish"() -> (w1299:bool)
        n853 = case shown="True" w1299 {
          frame False {
          }
          frame True {
            w1308 = 0.0 ("minimum value")
            w1309 = 10.0 ("maximum value")
            # "Grab offset in pulling\ndirection and add to \ndelta values"
            n854 = call-poly <vilib>:"DAQmx Create Virtual Channel.vi"("maximum value"=w1309, "minimum value"=w1308, "physical channels"=tag "Dev1/ao0") -> ("task out"=w1313:refnum<k21>, "error out"=w1312:errorcluster)  [unwired: 11 in]
            n855 = call-poly <vilib>:"DAQmx Create Virtual Channel.vi"("task in"=w1313, "maximum value"=w1309, "minimum value"=w1308, "physical channels"=tag "Dev1/ao1", "error in"=w1312) -> ("task out"=w1307:refnum<k21>, "error out"=w1306:errorcluster)  [unwired: 9 in]
            n856 = node-c288(i64 1 ("Period")) -> (w1315:T12)  [unwired: 3 in]
            n857 = timed-loop {
              timing: w1315 -> [_]
              timing-out: [_] -> w1314
              tunnel: w1307 -> [w1371]
              tunnel: w1306 -> [w1370]
              tunnel: [w1369] -> w1302
              tunnel: [w1368] -> w1301
              tunnel: [w1337] -> w1304
              tunnel: [w1350] -> w1300
              i -> [w1354]
              stop <- w1350 stop-if-true
              # "Send offset in direction\nof not-pulling to DAQ"
              n858 = node-c288() -> ()  [unwired: 1 in, 1 out]
              n859 = local read "Pulling direction"() -> (w1332:bool)
              n860 = local read "Conv Y (nm/V)"() -> (w1334:dbl)
              n861 = local read "Conv X (nm/V)"() -> (w1333:dbl)
              n862 = local read "Fixed X"() -> (w1341:dbl)
              n863 = local read "Fixed Y"() -> (w1340:dbl)
              n864 = Select(t=w1340, s=w1332, f=w1341) -> (s? t:f=w1342:dbl)
              n865 = Select(t=w1341, s=w1332, f=w1340) -> (s? t:f=w1339:dbl)
              n866 = Select(t=w1334, s=w1332, f=w1333) -> (s? t:f=w1329:dbl)
              n867 = Divide(x="Max fish\ndelta (nm)", y=w1329) -> (x/y=w1331:dbl)
              n868 = Divide(x="Min fish\ndelta (nm)", y=w1329) -> (x/y=w1330:dbl)
              n869 = Add(x=w1342, y=w1331) -> (x+y=w1344:dbl)
              n870 = Subtract(x=w1331, y=w1330) -> (x-y=w1346:dbl)
              n871 = Divide(x=w1346, y="Fish Speed (ms)") -> (x/y=w1347:dbl)
              n872 = flat-sequence {
                tunnel: w1332 -> [w1390]
                tunnel: w1339 -> [w1389]
                tunnel: w1371 -> [w1388]
                tunnel: w1370 -> [w1387]
                tunnel: w1347 -> [w1386]
                tunnel: w1344 -> [w1385]
                tunnel: "Fish Speed (ms)" -> [w1380]
                tunnel: [w1384] -> w1367
                tunnel: [w1383] -> w1366
                tunnel: [w1382] -> w1365
                tunnel: [w1381] -> w1364
                tunnel: [w1374] -> w1353
                tunnel: [w1373] -> w1338
                tunnel: [w1372] -> w1335
                tunnel: [w1437] -> w1363
                tunnel: w1367 -> [w1437]
                tunnel: [w1436] -> w1362
                tunnel: w1366 -> [w1436]
                tunnel: [w1435] -> w1361
                tunnel: w1365 -> [w1435]
                tunnel: [w1434] -> w1360
                tunnel: w1364 -> [w1434]
                tunnel: w1353 -> [w1433]
                tunnel: [w1433] -> w1352
                tunnel: w1338 -> [w1432]
                tunnel: [w1431] -> w1336
                tunnel: w1335 -> [w1431]
                tunnel: w1363 -> [w1448]
                tunnel: w1362 -> [w1447]
                tunnel: w1361 -> [w1446]
                tunnel: w1360 -> [w1445]
                tunnel: w1349 -> [w1444]
                tunnel: [w1443] -> w1369
                tunnel: [w1442] -> w1368
                tunnel: w1352 -> [w1441]
                tunnel: [w1440] -> w1337
                tunnel: w1336 -> [w1439]
                frame #0 {
                  n873 = local read "Mean force (pN)"() -> (w1379:dbl)
                  n874 = local read "Cutoff force (pN)"() -> (w1378:dbl)
                  n875 = Less Or Equal?(x=w1379, y=w1378) -> (x <= y?=w1376:bool)
                  n876 = And(x="Fish", y=w1376) -> (x .and. y?=w1377:bool)
                  n877 = case shown="True" w1377 {
                    selector: w1377 -> [w1392 _]
                    tunnel: w1390 -> [w1395 w1411]
                    tunnel: w1389 -> [_ w1410]
                    tunnel: w1388 -> [w1397 w1409]
                    tunnel: w1387 -> [w1396 w1408]
                    tunnel: w1386 -> [w1394 w1407]
                    tunnel: w1385 -> [w1393 w1406]
                    tunnel: [w1397 w1405] -> w1384
                    tunnel: [w1396 w1404] -> w1383
                    tunnel: [w1395 w1403] -> w1382
                    tunnel: [w1393 w1402] -> w1372
                    tunnel: [w1394 w1401] -> w1381
                    tunnel: w1380 -> [_ w1400]
                    tunnel: [w1392 w1399] -> w1374
                    tunnel: [FALSE w1398] -> w1373
                    frame False {
                    }
                    frame True {
                      n878 = while {
                        tunnel: w1411 -> [w1420]
                        tunnel: w1410 -> [w1419]
                        tunnel: w1409 -> [w1427]
                        tunnel: w1408 -> [w1426]
                        tunnel: w1407 -> [w1418]
                        tunnel: w1406 -> [w1424]
                        tunnel: [w1422] -> w1405
                        tunnel: [w1421] -> w1404
                        tunnel: [w1420] -> w1403
                        tunnel: [w1419] -> w1402
                        tunnel: [w1418] -> w1401
                        tunnel: w1400 -> [w1417]
                        tunnel: [w1412] -> w1399
                        tunnel: [w1412] -> w1398
                        i -> [w1416]
                        stop <- w1413 stop-if-true
                        n879 = Multiply(x=w1418, y=w1416) -> (x*y=w1425:dbl)
                        n880 = Subtract(x=w1424, y=w1425) -> (x-y=w1423:dbl)
                        n881 = Build Array(w1419, w1423) -> (w1430:dbl[])
                        n882 = Build Array(w1423, w1419) -> (w1429:dbl[])
                        n883 = Greater Or Equal?(x=w1416, y=w1417) -> (x >= y?=w1412:bool)
                        n884 = Select(t=w1430, s=w1420, f=w1429) -> (s? t:f=w1428:dbl[])
                        n885 = local read "Fish"() -> (w1414:bool)
                        n886 = Not(x=w1414) -> (.not. x?=w1415:bool)
                        n887 = call-poly <vilib>:"DAQmx Write.vi"("task/channels in"=w1427, "data"=w1428, "error in"=w1426) -> ("task out"=w1422:refnum<k21>, "error out"=w1421:errorcluster)  [unwired: 10 in, 1 out]
                        n888 = Compound Arithmetic op=OR(w1412, w1415) -> (w1413:bool)
                      }
                    }
                  }
                }
                frame #1 {
                  n889 = case shown="True" w1432 {
                    frame False {
                    }
                    frame True {
                      n890 = Wait (ms)(milliseconds to wait="Wait (ms)") -> ()  [unwired: 1 out]
                    }
                  }
                }
                frame #2 {
                  n891 = case shown="True" w1441 {
                    tunnel: w1448 -> [w1451 w1460]
                    tunnel: w1447 -> [w1450 w1459]
                    tunnel: w1446 -> [_ w1458]
                    tunnel: w1445 -> [_ w1457]
                    tunnel: w1444 -> [_ w1456]
                    tunnel: [w1451 w1455] -> w1443
                    tunnel: [w1450 w1454] -> w1442
                    tunnel: [FALSE w1453] -> w1440
                    tunnel: w1439 -> [_ w1452]
                    frame False {
                    }
                    frame True {
                      n892 = while {
                        tunnel: w1460 -> [w1492]
                        tunnel: w1459 -> [w1491]
                        tunnel: w1458 -> [w1463]
                        tunnel: w1457 -> [w1489]
                        tunnel: w1456 -> [w1488]
                        tunnel: [w1486] -> w1455
                        tunnel: [w1485] -> w1454
                        tunnel: [w1470] -> w1453
                        tunnel: w1452 -> [w1461]
                        i -> [w1477]
                        stop <- w1482 stop-if-true
                        # "If tether formed,\nimmediately change\nto new delta."
                        n893 = local read "Conv Y (nm/V)"() -> (w1464:dbl)
                        n894 = local read "Conv X (nm/V)"() -> (w1462:dbl)
                        n895 = local read "Fixed Y"() -> (w1471:dbl)
                        n896 = local read "Fixed X"() -> (w1476:dbl)
                        n897 = Select(t=w1464, s=w1463, f=w1462) -> (s? t:f=w1465:dbl)
                        n898 = local read "Cutoff force (pN)"() -> (w1478:dbl)
                        n899 = Divide(x="Delta after tether", y=w1465) -> (x/y=w1466:dbl)
                        n900 = Multiply(x=w1489, y=w1477) -> (x*y=w1490:dbl)
                        n901 = local read "Mean force (pN)"() -> (w1479:dbl)
                        n902 = Add(x=w1488, y=w1490) -> (x+y=w1473:dbl)
                        n903 = Select(t=w1471, s=w1463, f=w1476) -> (s? t:f=w1475:dbl)
                        n904 = Greater?(x=w1479, y=w1478) -> (0:w1470:bool)
                        n905 = Add(x=w1475, y=w1466) -> (x+y=w1474:dbl)
                        n906 = Select(t=w1474, s=w1470, f=w1473) -> (s? t:f=w1472:dbl)
                        n907 = local read "Fish Speed (ms)"() -> (w1484:i32)
                        n908 = Build Array(w1461, w1472) -> (w1487:dbl[])
                        n909 = Build Array(w1472, w1461) -> (w1468:dbl[])
                        n910 = Select(t=w1487, s=w1463, f=w1468) -> (s? t:f=w1467:dbl[])
                        n911 = case shown="True" w1470 {
                          tunnel: w1466 -> [_ _]
                          tunnel: w1467 -> [_ w1494]
                          frame False {
                          }
                          frame True {
                            n912 = Array To Cluster(array=w1494) -> (cluster=w1493:cluster{"[0]":dbl, "[1]":dbl})
                            n913 = local write "Trap position (V)"(w1493) -> ()
                          }
                        }
                        n914 = local read "Fish"() -> (w1481:bool)
                        n915 = Greater Or Equal?(x=w1477, y=w1484) -> (x >= y?=w1483:bool)
                        n916 = Not(x=w1481) -> (.not. x?=w1480:bool)
                        n917 = call-poly <vilib>:"DAQmx Write.vi"("task/channels in"=w1492, "data"=w1467, "error in"=w1491) -> ("task out"=w1486:refnum<k21>, "error out"=w1485:errorcluster)  [unwired: 10 in, 1 out]
                        n918 = Compound Arithmetic op=OR(w1483, w1480, w1470) -> (w1482:bool)
                      }
                    }
                  }
                }
              }
              n919 = Add(x=w1342, y=w1330) -> (x+y=w1349:dbl)
              n920 = Decrement(x="# attempts") -> (x-1=w1358:dbl)
              n921 = Greater Or Equal?(x=w1354, y=w1358) -> (x >= y?=w1357:bool)
              n922 = local read "Mean force (pN)"() -> (w1356:dbl)
              n923 = Greater?(x=w1356, y="Cutoff force (pN)") -> (0:w1351:bool)
              n924 = Compound Arithmetic op=OR(w1337, w1351, w1357) -> (w1350:bool)
              n925 = case shown="True" w1337 {
                frame False {
                }
                frame True {
                  n926 = call <vilib>:"Beep.vi"() -> ()  [unwired: 12 in]
                }
              }
              n927 = node-c288() -> ()  [unwired: 1 in, 1 out]
              "Tether" <- w1337
              "Attempt #" <- w1354
            }
            n928 = node-c288(w1314) -> ()  [unwired: 1 out]
            n929 = flat-sequence {
              tunnel: w1304 -> [w1323]
              tunnel: [w1323] -> w1303
              tunnel: w1302 -> [w1320]
              tunnel: w1301 -> [w1319]
              tunnel: w1300 -> [w1318]
              tunnel: w1303 -> [w1325]
              frame #0 {
                w1322 = T15 1 items=["no dialog", "OK message", "continue or stop message", "OK message + warnings", "continue/stop + warnings"] ("type of dialog (OK msg:1)")
                n930 = call <vilib>:"DAQmx Clear Task.vi"("task in"=w1320, "error in"=w1319) -> ("error out"=w1321:errorcluster)  [unwired: 13 in]
                n931 = Not(x=w1318) -> (.not. x?=w1317:bool)
                n932 = local write "Fish"(w1317) -> ()
                n933 = Wait (ms)(milliseconds to wait=u32 300) -> ()  [unwired: 1 out]
                n934 = call <vilib>:"Simple Error Handler.vi"("type of dialog (OK msg:1)"=w1322, "error in (no error)"=w1321) -> ()  [unwired: 3 in, 5 out]
              }
              frame #1 {
                n935 = And(x=w1325, y="Raster after\n tether?") -> (x .and. y?=w1326:bool)
                n936 = case shown="True" w1326 {
                  selector: w1326 -> [_ w1328]
                  frame False {
                  }
                  frame True {
                    n937 = property on="Raster scan" class="Bool (strict)"("Val(Sgnl)"=w1328) -> ()  [unwired: 2 in, 2 out]
                    n938 = property on="Inject Sample" class="Bool (strict)"("Val(Sgnl)"=FALSE ("Value (Signaling)")) -> ()  [unwired: 2 in, 2 out]
                  }
                }
              }
            }
          }
        }
      }
      event "Load param": Value Change {
        n939 = event-data() -> ()  [unwired: 1 in, 6 out]
        n940 = property on="Scan Parameters" class="Arr (strict)"() -> ("Index Values"=w1507:u32[])  [unwired: 2 in, 2 out]
        n941 = Index Array(array=w1507, index=0) -> (element=w1504:u32)
        n942 = Index Array(array="Scan Parameters", index=w1504) -> (element=w1503:T18)
        n943 = Unbundle(w1503) -> ("# scans 2"=w1502:i32)  [unwired: 4 out]
        n944 = local write "Load param"(FALSE ("Load param")) -> ()
        n945 = property on="# scans" class="DigNum (strict)"("Val(Sgnl)"=w1502) -> ()  [unwired: 2 in, 2 out]
      }
      event "Step size (nm)", "Scan speed (nm/s)", "# scans", "Pulling direction", "Scan range (nm)": Value Change {
        n946 = event-data() -> ()  [unwired: 1 in, 6 out]
        n947 = local read "Pulling direction"() -> (w1538:bool)
        n948 = Reciprocal(x="Scan speed (nm/s)") -> (1/x=w1530:dbl)
        n949 = local read "Conv Y (nm/V)"() -> (w1536:dbl)
        n950 = local read "Conv X (nm/V)"() -> (w1537:dbl)
        n951 = Multiply(x="Step size (nm)", y=w1530) -> (x*y=w1528:dbl)
        n952 = Divide(x="Scan range (nm)", y="Step size (nm)") -> (x/y=w1535:dbl)
        n953 = Absolute Value(x=w1535) -> (abs(x)=w1534:dbl)
        n954 = Multiply(x=w1528, y=1000.0) -> (x*y=w1515:dbl)
        n955 = Select(t=w1536, s=w1538, f=w1537) -> (s? t:f=w1526:dbl)
        n956 = Multiply(x="# scans", y=2) -> (x*y=w1514:i32)
        n957 = To Unsigned Quad Integer(1:w1534) -> (0:w1524:u64)
        "Scan steps (mirror)" <- w1524
        n958 = Divide(x="Scan range (nm)", y=w1526) -> (x/y=→"Scan range (V)":dbl)
        n959 = Multiply(x=w1524, y=w1515) -> (x*y=w1523:dbl)
        n960 = Divide(x="Step size (nm)", y=w1526) -> (x/y=→"Scan increment (V)":dbl)
        n961 = Round Toward +Infinity(x=w1515) -> (ceil(x): smallest int >= x=w1512:dbl)
        "Time per step (ms)" <- w1512
        n962 = local read "Data update period (s/set)"() -> (w1518:dbl)
        n963 = Multiply(x=w1514, y=w1523) -> (x*y=w1521:dbl)
        n964 = Divide(x=w1521, y=1000.0) -> (x/y=w1519:dbl)
        "Total raster time (s)" <- w1519
        n965 = local read "Data update period (s/set)"() -> (w1510:dbl)
        n966 = Divide(x=w1519, y=w1518) -> (x/y=w1517:dbl)
        n967 = Round Toward -Infinity(1:w1517) -> (0:→"N sets to be saved":dbl)
        n968 = Multiply(x=w1510, y=1000.0) -> (x*y=w1508:dbl)
        n969 = Less?(x=w1512, y=w1508) -> (x < y?=w1511:bool)
        n970 = case shown="True" w1511 {
          selector: w1511 -> [_ w1539]
          frame False {
          }
          frame True {
            n971 = call "Display Message to User"("Enable"=w1539) -> ()  [unwired: 9 in, 2 out]
          }
        }
      }
      event "Averaging Number": Value Change {
        n972 = event-data() -> ()  [unwired: 1 in, 6 out]
        n973 = local read "# Samples/channel (in)"() -> (w1543:i32)
        n974 = local read "Averaging Number"() -> (w1541:i32)
        n975 = Quotient & Remainder(x=w1543, y=w1541) -> (floor(x/y)=w1542:i32)  [unwired: 1 out]
        n976 = Multiply(x=w1542, y=w1541) -> (x*y=w1540:i32)
        n977 = local write "# Samples/channel (in)"(w1540) -> ()
      }
    }
    n978 = node-c288() -> ()  [unwired: 1 in, 1 out]
  }
  n979 = call <vilib>:"Simple Error Handler.vi"("error in (no error)"=w104) -> ()  [unwired: 4 in, 5 out]
  n980 = disable-structure shown="Enabled" {
    frame Disabled {
      n981 = node-c288(2 ("Processor")) -> (w1549:T12)  [unwired: 3 in]
      n982 = timed-loop "Pump Control" {
        timing: w1549 -> [_]
        timing-out: [_] -> w1548
        tunnel: refnum<visa-resource-name> "COM6" ("VISA resource name") -> [w1551]
        stop <- w1550 stop-if-true
        n983 = node-c288() -> ()  [unwired: 1 in, 1 out]
        n984 = event shown="[4] \"Inject Pump 1\": Value Change" {
          selector: _ -> [_ _ _ _ _ _ _ _ _]
          dyn-events: _ -> [_ _ _ _ _ _ _ _ _]
          timeout: _ -> [_ _ _ _ _ _ _ _ _]
          tunnel: w1551 -> [w1559 w1655 _ w1731 w1859 w2002 w2047 w2105 w2164]
          tunnel: [_ _ w1730 _ _ _ _ _ _] -> w1550
          event "Flush Pump 1": Value Change {
            w1560 = "\r"
            n985 = event-data() -> ()  [unwired: 1 in, 5 out]
            n986 = call-poly "VISA Configure Serial Port"("VISA resource name"=w1559) -> ("VISA resource name out"=w1573:refnum<visa-resource-name>, "error out"=w1574:errorcluster)  [unwired: 13 in]
            n987 = local read "Write Wait"() -> (w1552:i32)
            n988 = Concatenate Strings("enter pump1", w1560) -> (w1561:string)
            n989 = flat-sequence {
              tunnel: w1574 -> [w1593]
              tunnel: w1573 -> [w1595]
              tunnel: [w1594] -> w1590
              tunnel: [w1592] -> w1589
              tunnel: w1561 -> [w1591]
              tunnel: w1590 -> [w1598]
              tunnel: [w1598] -> w1588
              tunnel: w1589 -> [w1597]
              tunnel: [w1597] -> w1587
              tunnel: w1552 -> [w1596]
              tunnel: [w1603] -> w1586
              tunnel: w1566 -> [w1602]
              tunnel: [w1599] -> w1585
              tunnel: w1588 -> [w1601]
              tunnel: w1587 -> [w1600]
              tunnel: w1586 -> [w1606]
              tunnel: [w1606] -> w1584
              tunnel: [w1605] -> w1583
              tunnel: w1585 -> [w1605]
              tunnel: w1552 -> [w1604]
              tunnel: w1584 -> [w1611]
              tunnel: [w1610] -> w1582
              tunnel: w1569 -> [w1609]
              tunnel: w1583 -> [w1608]
              tunnel: [w1607] -> w1581
              tunnel: w1582 -> [w1614]
              tunnel: [w1614] -> w1580
              tunnel: [w1613] -> w1579
              tunnel: w1581 -> [w1613]
              tunnel: w1552 -> [w1612]
              tunnel: w1580 -> [w1619]
              tunnel: [w1618] -> w1578
              tunnel: w1572 -> [w1617]
              tunnel: w1579 -> [w1616]
              tunnel: [w1615] -> w1577
              tunnel: [w1622] -> w1576
              tunnel: w1578 -> [w1622]
              tunnel: [w1621] -> w1575
              tunnel: w1577 -> [w1621]
              tunnel: w1552 -> [w1620]
              tunnel: w1576 -> [w1627]
              tunnel: w1575 -> [w1624]
              tunnel: [w1626] -> w1555
              tunnel: [w1625] -> w1553
              tunnel: [w1632] -> w1556
              tunnel: w1555 -> [w1632]
              tunnel: [w1631] -> w1554
              tunnel: w1553 -> [w1631]
              tunnel: w1552 -> [w1630]
              tunnel: w1556 -> [w1634]
              tunnel: w1554 -> [w1633]
              frame #0 {
                n990 = VISA Write(VISA resource name=w1595, write buffer=w1591, error in (no error)=w1593) -> (VISA resource name out=w1594:refnum<visa-resource-name>, error out=w1592:errorcluster)  [unwired: 1 out]
              }
              frame #1 {
                n991 = Wait (ms)(milliseconds to wait=w1596) -> ()  [unwired: 1 out]
              }
              frame #2 {
                n992 = VISA Write(VISA resource name=w1601, write buffer=w1602, error in (no error)=w1600) -> (VISA resource name out=w1603:refnum<visa-resource-name>, error out=w1599:errorcluster)  [unwired: 1 out]
              }
              frame #3 {
                n993 = Wait (ms)(milliseconds to wait=w1604) -> ()  [unwired: 1 out]
              }
              frame #4 {
                n994 = VISA Write(VISA resource name=w1611, write buffer=w1609, error in (no error)=w1608) -> (VISA resource name out=w1610:refnum<visa-resource-name>, error out=w1607:errorcluster)  [unwired: 1 out]
              }
              frame #5 {
                n995 = Wait (ms)(milliseconds to wait=w1612) -> ()  [unwired: 1 out]
              }
              frame #6 {
                n996 = VISA Write(VISA resource name=w1619, write buffer=w1617, error in (no error)=w1616) -> (VISA resource name out=w1618:refnum<visa-resource-name>, error out=w1615:errorcluster)  [unwired: 1 out]
              }
              frame #7 {
                n997 = Wait (ms)(milliseconds to wait=w1620) -> ()  [unwired: 1 out]
              }
              frame #8 {
                n998 = Concatenate Strings("start ", "\r") -> (w1623:string)
                n999 = VISA Write(VISA resource name=w1627, write buffer=w1623, error in (no error)=w1624) -> (VISA resource name out=w1626:refnum<visa-resource-name>, error out=w1625:errorcluster)  [unwired: 1 out]
              }
              frame #9 {
                n1000 = Wait (ms)(milliseconds to wait=w1630) -> ()  [unwired: 1 out]
              }
              frame #10 {
                n1001 = local write "Flush Pump 1"(FALSE ("Flush Pump 1")) -> ()
                n1002 = Concatenate Strings("enter main ", "\r") -> (w1638:string)
                n1003 = VISA Write(VISA resource name=w1634, write buffer=w1638, error in (no error)=w1633) -> (VISA resource name out=w1637:refnum<visa-resource-name>, error out=w1636:errorcluster)  [unwired: 1 out]
                n1004 = VISA Close(VISA resource name=w1637, error in (no error)=w1636) -> ()  [unwired: 1 out]
              }
            }
            n1005 = Concatenate Strings("set units 4 ", w1560) -> (w1566:string)
            n1006 = Multiply(x="Flush\nRate (ul/min)", y=60) -> (x*y=w1564:dbl)
            n1007 = Number To Decimal String(number=w1564) -> (decimal integer string=w1567:string)  [unwired: 1 in]
            n1008 = Concatenate Strings("set rate ", w1567, w1560) -> (w1569:string)
            n1009 = Number To Decimal String(number="Flush\nVolume (ul)") -> (decimal integer string=w1571:string)  [unwired: 1 in]
            n1010 = Concatenate Strings("set volume ", w1571, w1560) -> (w1572:string)
          }
          event "Flush Pump 2": Value Change {
            w1646 = "\r"
            n1011 = event-data() -> ()  [unwired: 1 in, 5 out]
            n1012 = call-poly "VISA Configure Serial Port"("VISA resource name"=w1655) -> ("VISA resource name out"=w1666:refnum<visa-resource-name>, "error out"=w1667:errorcluster)  [unwired: 13 in]
            n1013 = local read "Write Wait"() -> (w1641:i32)
            n1014 = Concatenate Strings("enter pump2", w1646) -> (w1647:string)
            n1015 = flat-sequence {
              tunnel: w1667 -> [w1682]
              tunnel: w1666 -> [w1684]
              tunnel: [w1683] -> w1652
              tunnel: [w1681] -> w1650
              tunnel: w1647 -> [w1680]
              tunnel: w1652 -> [w1687]
              tunnel: [w1687] -> w1651
              tunnel: w1650 -> [w1686]
              tunnel: [w1686] -> w1649
              tunnel: w1641 -> [w1685]
              tunnel: [w1692] -> w1679
              tunnel: w1659 -> [w1691]
              tunnel: [w1688] -> w1678
              tunnel: w1651 -> [w1690]
              tunnel: w1649 -> [w1689]
              tunnel: w1679 -> [w1695]
              tunnel: [w1695] -> w1677
              tunnel: [w1694] -> w1676
              tunnel: w1678 -> [w1694]
              tunnel: w1641 -> [w1693]
              tunnel: w1677 -> [w1700]
              tunnel: [w1699] -> w1675
              tunnel: w1662 -> [w1698]
              tunnel: w1676 -> [w1697]
              tunnel: [w1696] -> w1674
              tunnel: w1675 -> [w1703]
              tunnel: [w1703] -> w1673
              tunnel: [w1702] -> w1672
              tunnel: w1674 -> [w1702]
              tunnel: w1641 -> [w1701]
              tunnel: w1673 -> [w1708]
              tunnel: [w1707] -> w1671
              tunnel: w1665 -> [w1706]
              tunnel: w1672 -> [w1705]
              tunnel: [w1704] -> w1670
              tunnel: [w1711] -> w1669
              tunnel: w1671 -> [w1711]
              tunnel: [w1710] -> w1668
              tunnel: w1670 -> [w1710]
              tunnel: w1641 -> [w1709]
              tunnel: w1669 -> [w1718]
              tunnel: w1668 -> [w1717]
              tunnel: [w1713] -> w1645
              tunnel: [w1712] -> w1643
              tunnel: w1645 -> [w1721]
              tunnel: [w1721] -> w1644
              tunnel: w1643 -> [w1720]
              tunnel: [w1720] -> w1642
              tunnel: w1641 -> [w1719]
              tunnel: w1644 -> [w1725]
              tunnel: w1642 -> [w1724]
              frame #0 {
                n1016 = VISA Write(VISA resource name=w1684, write buffer=w1680, error in (no error)=w1682) -> (VISA resource name out=w1683:refnum<visa-resource-name>, error out=w1681:errorcluster)  [unwired: 1 out]
              }
              frame #1 {
                n1017 = Wait (ms)(milliseconds to wait=w1685) -> ()  [unwired: 1 out]
              }
              frame #2 {
                n1018 = VISA Write(VISA resource name=w1690, write buffer=w1691, error in (no error)=w1689) -> (VISA resource name out=w1692:refnum<visa-resource-name>, error out=w1688:errorcluster)  [unwired: 1 out]
              }
              frame #3 {
                n1019 = Wait (ms)(milliseconds to wait=w1693) -> ()  [unwired: 1 out]
              }
              frame #4 {
                n1020 = VISA Write(VISA resource name=w1700, write buffer=w1698, error in (no error)=w1697) -> (VISA resource name out=w1699:refnum<visa-resource-name>, error out=w1696:errorcluster)  [unwired: 1 out]
              }
              frame #5 {
                n1021 = Wait (ms)(milliseconds to wait=w1701) -> ()  [unwired: 1 out]
              }
              frame #6 {
                n1022 = VISA Write(VISA resource name=w1708, write buffer=w1706, error in (no error)=w1705) -> (VISA resource name out=w1707:refnum<visa-resource-name>, error out=w1704:errorcluster)  [unwired: 1 out]
              }
              frame #7 {
                n1023 = Wait (ms)(milliseconds to wait=w1709) -> ()  [unwired: 1 out]
              }
              frame #8 {
                n1024 = Concatenate Strings("start ", "\r") -> (w1716:string)
                n1025 = VISA Write(VISA resource name=w1718, write buffer=w1716, error in (no error)=w1717) -> (VISA resource name out=w1713:refnum<visa-resource-name>, error out=w1712:errorcluster)  [unwired: 1 out]
              }
              frame #9 {
                n1026 = Wait (ms)(milliseconds to wait=w1719) -> ()  [unwired: 1 out]
              }
              frame #10 {
                n1027 = local write "Flush Pump 2"(FALSE ("Flush Pump 1")) -> ()
                n1028 = Concatenate Strings("enter main ", "\r") -> (w1726:string)
                n1029 = VISA Write(VISA resource name=w1725, write buffer=w1726, error in (no error)=w1724) -> (VISA resource name out=w1723:refnum<visa-resource-name>, error out=w1722:errorcluster)  [unwired: 1 out]
                n1030 = VISA Close(VISA resource name=w1723, error in (no error)=w1722) -> ()  [unwired: 1 out]
              }
            }
            n1031 = Concatenate Strings("set units 4 ", w1646) -> (w1659:string)
            n1032 = Multiply(x="Flush \nRate (ul/min)  2", y=60) -> (x*y=w1657:dbl)
            n1033 = Number To Decimal String(number=w1657) -> (decimal integer string=w1660:string)  [unwired: 1 in]
            n1034 = Concatenate Strings("set rate ", w1660, w1646) -> (w1662:string)
            n1035 = Number To Decimal String(number="Flush\nVolume (ul)  2") -> (decimal integer string=w1664:string)  [unwired: 1 in]
            n1036 = Concatenate Strings("set volume ", w1664, w1646) -> (w1665:string)
          }
          event "Stop": Value Change {
            n1037 = event-data() -> ()  [unwired: 1 in, 5 out]
            n1038 = local read "Stop"() -> (w1730:bool)
          }
          event "Inject Pump 2": Value Change {
            n1039 = event-data() -> ()  [unwired: 1 in, 5 out]
            n1040 = case shown="True" "Inject Pump 2" {
              tunnel: w1731 -> [w1734 w1776]
              frame False {
                n1041 = local read "Write Wait"() -> (w1733:i32)
                n1042 = call-poly "VISA Configure Serial Port"("VISA resource name"=w1734) -> ("VISA resource name out"=w1738:refnum<visa-resource-name>, "error out"=w1739:errorcluster)  [unwired: 13 in]
                n1043 = Concatenate Strings("enter pump2", "\r") -> (w1736:string)
                n1044 = flat-sequence {
                  tunnel: w1739 -> [w1750]
                  tunnel: w1738 -> [w1752]
                  tunnel: [w1751] -> w1747
                  tunnel: [w1749] -> w1746
                  tunnel: w1736 -> [w1748]
                  tunnel: w1747 -> [w1755]
                  tunnel: w1746 -> [w1754]
                  tunnel: [w1755] -> w1745
                  tunnel: [w1754] -> w1744
                  tunnel: w1733 -> [w1753]
                  tunnel: [w1759] -> w1743
                  tunnel: [w1758] -> w1742
                  tunnel: w1745 -> [w1757]
                  tunnel: w1744 -> [w1756]
                  tunnel: w1743 -> [w1765]
                  tunnel: [w1765] -> w1741
                  tunnel: w1742 -> [w1764]
                  tunnel: [w1764] -> w1740
                  tunnel: w1733 -> [w1763]
                  tunnel: w1741 -> [w1769]
                  tunnel: w1740 -> [w1768]
                  frame #0 {
                    n1045 = VISA Write(VISA resource name=w1752, write buffer=w1748, error in (no error)=w1750) -> (VISA resource name out=w1751:refnum<visa-resource-name>, error out=w1749:errorcluster)  [unwired: 1 out]
                  }
                  frame #1 {
                    n1046 = Wait (ms)(milliseconds to wait=w1753) -> ()  [unwired: 1 out]
                  }
                  frame #2 {
                    n1047 = Concatenate Strings("stop ", "\r") -> (w1762:string)
                    n1048 = VISA Write(VISA resource name=w1757, write buffer=w1762, error in (no error)=w1756) -> (VISA resource name out=w1759:refnum<visa-resource-name>, error out=w1758:errorcluster)  [unwired: 1 out]
                  }
                  frame #3 {
                    n1049 = Wait (ms)(milliseconds to wait=w1763) -> ()  [unwired: 1 out]
                  }
                  frame #4 {
                    n1050 = Concatenate Strings("enter main ", "\r") -> (w1770:string)
                    n1051 = VISA Write(VISA resource name=w1769, write buffer=w1770, error in (no error)=w1768) -> (VISA resource name out=w1767:refnum<visa-resource-name>, error out=w1766:errorcluster)  [unwired: 1 out]
                    n1052 = VISA Close(VISA resource name=w1767, error in (no error)=w1766) -> ()  [unwired: 1 out]
                  }
                }
              }
              frame True {
                w1789 = "\r"
                n1053 = call-poly "VISA Configure Serial Port"("VISA resource name"=w1776) -> ("VISA resource name out"=w1778:refnum<visa-resource-name>, "error out"=w1777:errorcluster)  [unwired: 13 in]
                n1054 = local read "Write Wait"() -> (w1773:i32)
                n1055 = Concatenate Strings("enter pump2", w1789) -> (w1788:string)
                n1056 = flat-sequence {
                  tunnel: w1777 -> [w1812]
                  tunnel: w1778 -> [w1814]
                  tunnel: [w1813] -> w1809
                  tunnel: [w1811] -> w1808
                  tunnel: w1788 -> [w1810]
                  tunnel: w1809 -> [w1817]
                  tunnel: [w1817] -> w1807
                  tunnel: w1808 -> [w1816]
                  tunnel: [w1816] -> w1806
                  tunnel: w1773 -> [w1815]
                  tunnel: [w1822] -> w1805
                  tunnel: w1785 -> [w1821]
                  tunnel: [w1818] -> w1804
                  tunnel: w1807 -> [w1820]
                  tunnel: w1806 -> [w1819]
                  tunnel: w1805 -> [w1825]
                  tunnel: [w1825] -> w1803
                  tunnel: [w1824] -> w1802
                  tunnel: w1804 -> [w1824]
                  tunnel: w1773 -> [w1823]
                  tunnel: w1803 -> [w1830]
                  tunnel: [w1829] -> w1801
                  tunnel: w1782 -> [w1828]
                  tunnel: w1802 -> [w1827]
                  tunnel: [w1826] -> w1800
                  tunnel: w1801 -> [w1833]
                  tunnel: [w1833] -> w1799
                  tunnel: [w1832] -> w1798
                  tunnel: w1800 -> [w1832]
                  tunnel: w1773 -> [w1831]
                  tunnel: w1799 -> [w1838]
                  tunnel: [w1837] -> w1797
                  tunnel: w1779 -> [w1836]
                  tunnel: w1798 -> [w1835]
                  tunnel: [w1834] -> w1796
                  tunnel: [w1841] -> w1795
                  tunnel: w1797 -> [w1841]
                  tunnel: [w1840] -> w1794
                  tunnel: w1796 -> [w1840]
                  tunnel: w1773 -> [w1839]
                  tunnel: w1795 -> [w1848]
                  tunnel: w1794 -> [w1847]
                  tunnel: [w1843] -> w1793
                  tunnel: [w1842] -> w1792
                  tunnel: w1793 -> [w1851]
                  tunnel: [w1851] -> w1791
                  tunnel: w1792 -> [w1850]
                  tunnel: [w1850] -> w1790
                  tunnel: w1773 -> [w1849]
                  tunnel: w1791 -> [w1855]
                  tunnel: w1790 -> [w1854]
                  frame #0 {
                    n1057 = VISA Write(VISA resource name=w1814, write buffer=w1810, error in (no error)=w1812) -> (VISA resource name out=w1813:refnum<visa-resource-name>, error out=w1811:errorcluster)  [unwired: 1 out]
                  }
                  frame #1 {
                    n1058 = Wait (ms)(milliseconds to wait=w1815) -> ()  [unwired: 1 out]
                  }
                  frame #2 {
                    n1059 = VISA Write(VISA resource name=w1820, write buffer=w1821, error in (no error)=w1819) -> (VISA resource name out=w1822:refnum<visa-resource-name>, error out=w1818:errorcluster)  [unwired: 1 out]
                  }
                  frame #3 {
                    n1060 = Wait (ms)(milliseconds to wait=w1823) -> ()  [unwired: 1 out]
                  }
                  frame #4 {
                    n1061 = VISA Write(VISA resource name=w1830, write buffer=w1828, error in (no error)=w1827) -> (VISA resource name out=w1829:refnum<visa-resource-name>, error out=w1826:errorcluster)  [unwired: 1 out]
                  }
                  frame #5 {
                    n1062 = Wait (ms)(milliseconds to wait=w1831) -> ()  [unwired: 1 out]
                  }
                  frame #6 {
                    n1063 = VISA Write(VISA resource name=w1838, write buffer=w1836, error in (no error)=w1835) -> (VISA resource name out=w1837:refnum<visa-resource-name>, error out=w1834:errorcluster)  [unwired: 1 out]
                  }
                  frame #7 {
                    n1064 = Wait (ms)(milliseconds to wait=w1839) -> ()  [unwired: 1 out]
                  }
                  frame #8 {
                    n1065 = Concatenate Strings("start ", "\r") -> (w1846:string)
                    n1066 = VISA Write(VISA resource name=w1848, write buffer=w1846, error in (no error)=w1847) -> (VISA resource name out=w1843:refnum<visa-resource-name>, error out=w1842:errorcluster)  [unwired: 1 out]
                  }
                  frame #9 {
                    n1067 = Wait (ms)(milliseconds to wait=w1849) -> ()  [unwired: 1 out]
                  }
                  frame #10 {
                    n1068 = Concatenate Strings("enter main ", "\r") -> (w1856:string)
                    n1069 = VISA Write(VISA resource name=w1855, write buffer=w1856, error in (no error)=w1854) -> (VISA resource name out=w1853:refnum<visa-resource-name>, error out=w1852:errorcluster)  [unwired: 1 out]
                    n1070 = VISA Close(VISA resource name=w1853, error in (no error)=w1852) -> ()  [unwired: 1 out]
                  }
                }
                n1071 = local read "Normal \nRate (ul/hr)  2"() -> (w1774:dbl)
                n1072 = Concatenate Strings("set units 4 ", w1789) -> (w1785:string)
                n1073 = local read "Normal \nVolume (ul) 2"() -> (w1775:dbl)
                n1074 = Number To Decimal String(number=w1774) -> (decimal integer string=w1784:string)  [unwired: 1 in]
                n1075 = Concatenate Strings("set rate ", w1784, w1789) -> (w1782:string)
                n1076 = Number To Decimal String(number=w1775) -> (decimal integer string=w1780:string)  [unwired: 1 in]
                n1077 = Concatenate Strings("set volume ", w1780, w1789) -> (w1779:string)
              }
            }
          }
          event "Inject Pump 1": Value Change {
            n1078 = event-data() -> ()  [unwired: 1 in, 5 out]
            n1079 = case shown="True" "Inject Pump 1" {
              tunnel: w1859 -> [w1862 w1904]
              frame False {
                n1080 = local read "Write Wait"() -> (w1861:i32)
                n1081 = call-poly "VISA Configure Serial Port"("VISA resource name"=w1862) -> ("VISA resource name out"=w1866:refnum<visa-resource-name>, "error out"=w1867:errorcluster)  [unwired: 13 in]
                n1082 = Concatenate Strings("enter pump1", "\r") -> (w1864:string)
                n1083 = flat-sequence {
                  tunnel: w1867 -> [w1878]
                  tunnel: w1866 -> [w1880]
                  tunnel: [w1879] -> w1875
                  tunnel: [w1877] -> w1874
                  tunnel: w1864 -> [w1876]
                  tunnel: w1875 -> [w1883]
                  tunnel: w1874 -> [w1882]
                  tunnel: [w1883] -> w1873
                  tunnel: [w1882] -> w1872
                  tunnel: w1861 -> [w1881]
                  tunnel: [w1887] -> w1871
                  tunnel: [w1886] -> w1870
                  tunnel: w1873 -> [w1885]
                  tunnel: w1872 -> [w1884]
                  tunnel: w1871 -> [w1893]
                  tunnel: [w1893] -> w1869
                  tunnel: w1870 -> [w1892]
                  tunnel: [w1892] -> w1868
                  tunnel: w1861 -> [w1891]
                  tunnel: w1869 -> [w1897]
                  tunnel: w1868 -> [w1896]
                  frame #0 {
                    n1084 = VISA Write(VISA resource name=w1880, write buffer=w1876, error in (no error)=w1878) -> (VISA resource name out=w1879:refnum<visa-resource-name>, error out=w1877:errorcluster)  [unwired: 1 out]
                  }
                  frame #1 {
                    n1085 = Wait (ms)(milliseconds to wait=w1881) -> ()  [unwired: 1 out]
                  }
                  frame #2 {
                    n1086 = Concatenate Strings("stop ", "\r") -> (w1890:string)
                    n1087 = VISA Write(VISA resource name=w1885, write buffer=w1890, error in (no error)=w1884) -> (VISA resource name out=w1887:refnum<visa-resource-name>, error out=w1886:errorcluster)  [unwired: 1 out]
                  }
                  frame #3 {
                    n1088 = Wait (ms)(milliseconds to wait=w1891) -> ()  [unwired: 1 out]
                  }
                  frame #4 {
                    n1089 = Concatenate Strings("enter main ", "\r") -> (w1898:string)
                    n1090 = VISA Write(VISA resource name=w1897, write buffer=w1898, error in (no error)=w1896) -> (VISA resource name out=w1895:refnum<visa-resource-name>, error out=w1894:errorcluster)  [unwired: 1 out]
                    n1091 = VISA Close(VISA resource name=w1895, error in (no error)=w1894) -> ()  [unwired: 1 out]
                  }
                }
              }
              frame True {
                w1917 = "\r"
                n1092 = call-poly "VISA Configure Serial Port"("VISA resource name"=w1904) -> ("VISA resource name out"=w1906:refnum<visa-resource-name>, "error out"=w1905:errorcluster)  [unwired: 13 in]
                n1093 = local read "Write Wait"() -> (w1901:i32)
                n1094 = flat-sequence {
                  tunnel: w1905 -> [w1940]
                  tunnel: w1906 -> [w1942]
                  tunnel: [w1941] -> w1937
                  tunnel: [w1939] -> w1936
                  tunnel: w1916 -> [w1938]
                  tunnel: w1937 -> [w1945]
                  tunnel: [w1945] -> w1935
                  tunnel: w1936 -> [w1944]
                  tunnel: [w1944] -> w1934
                  tunnel: w1901 -> [w1943]
                  tunnel: [w1950] -> w1933
                  tunnel: w1913 -> [w1949]
                  tunnel: [w1946] -> w1932
                  tunnel: w1935 -> [w1948]
                  tunnel: w1934 -> [w1947]
                  tunnel: w1933 -> [w1953]
                  tunnel: [w1953] -> w1931
                  tunnel: [w1952] -> w1930
                  tunnel: w1932 -> [w1952]
                  tunnel: w1901 -> [w1951]
                  tunnel: w1931 -> [w1958]
                  tunnel: [w1957] -> w1929
                  tunnel: w1910 -> [w1956]
                  tunnel: w1930 -> [w1955]
                  tunnel: [w1954] -> w1928
                  tunnel: w1929 -> [w1961]
                  tunnel: [w1961] -> w1927
                  tunnel: [w1960] -> w1926
                  tunnel: w1928 -> [w1960]
                  tunnel: w1901 -> [w1959]
                  tunnel: w1927 -> [w1966]
                  tunnel: [w1965] -> w1925
                  tunnel: w1907 -> [w1964]
                  tunnel: w1926 -> [w1963]
                  tunnel: [w1962] -> w1924
                  tunnel: [w1969] -> w1923
                  tunnel: w1925 -> [w1969]
                  tunnel: [w1968] -> w1922
                  tunnel: w1924 -> [w1968]
                  tunnel: w1901 -> [w1967]
                  tunnel: w1923 -> [w1976]
                  tunnel: w1922 -> [w1975]
                  tunnel: [w1971] -> w1921
                  tunnel: [w1970] -> w1920
                  tunnel: w1921 -> [w1979]
                  tunnel: [w1979] -> w1919
                  tunnel: w1920 -> [w1978]
                  tunnel: [w1978] -> w1918
                  tunnel: w1901 -> [w1977]
                  tunnel: w1919 -> [w1983]
                  tunnel: w1918 -> [w1982]
                  frame #0 {
                    n1095 = VISA Write(VISA resource name=w1942, write buffer=w1938, error in (no error)=w1940) -> (VISA resource name out=w1941:refnum<visa-resource-name>, error out=w1939:errorcluster)  [unwired: 1 out]
                  }
                  frame #1 {
                    n1096 = Wait (ms)(milliseconds to wait=w1943) -> ()  [unwired: 1 out]
                  }
                  frame #2 {
                    n1097 = VISA Write(VISA resource name=w1948, write buffer=w1949, error in (no error)=w1947) -> (VISA resource name out=w1950:refnum<visa-resource-name>, error out=w1946:errorcluster)  [unwired: 1 out]
                  }
                  frame #3 {
                    n1098 = Wait (ms)(milliseconds to wait=w1951) -> ()  [unwired: 1 out]
                  }
                  frame #4 {
                    n1099 = VISA Write(VISA resource name=w1958, write buffer=w1956, error in (no error)=w1955) -> (VISA resource name out=w1957:refnum<visa-resource-name>, error out=w1954:errorcluster)  [unwired: 1 out]
                  }
                  frame #5 {
                    n1100 = Wait (ms)(milliseconds to wait=w1959) -> ()  [unwired: 1 out]
                  }
                  frame #6 {
                    n1101 = VISA Write(VISA resource name=w1966, write buffer=w1964, error in (no error)=w1963) -> (VISA resource name out=w1965:refnum<visa-resource-name>, error out=w1962:errorcluster)  [unwired: 1 out]
                  }
                  frame #7 {
                    n1102 = Wait (ms)(milliseconds to wait=w1967) -> ()  [unwired: 1 out]
                  }
                  frame #8 {
                    n1103 = Concatenate Strings("start ", "\r") -> (w1974:string)
                    n1104 = VISA Write(VISA resource name=w1976, write buffer=w1974, error in (no error)=w1975) -> (VISA resource name out=w1971:refnum<visa-resource-name>, error out=w1970:errorcluster)  [unwired: 1 out]
                  }
                  frame #9 {
                    n1105 = Wait (ms)(milliseconds to wait=w1977) -> ()  [unwired: 1 out]
                  }
                  frame #10 {
                    n1106 = Concatenate Strings("enter main ", "\r") -> (w1984:string)
                    n1107 = VISA Write(VISA resource name=w1983, write buffer=w1984, error in (no error)=w1982) -> (VISA resource name out=w1981:refnum<visa-resource-name>, error out=w1980:errorcluster)  [unwired: 1 out]
                    n1108 = VISA Close(VISA resource name=w1981, error in (no error)=w1980) -> ()  [unwired: 1 out]
                  }
                }
                n1109 = Concatenate Strings("enter pump1", w1917) -> (w1916:string)
                n1110 = local read "Normal \nRate (ul/hr)"() -> (w1902:dbl)
                n1111 = Concatenate Strings("set units 4 ", w1917) -> (w1913:string)
                n1112 = local read "Normal \nVolume (ul)"() -> (w1903:dbl)
                n1113 = Number To Decimal String(number=w1902) -> (decimal integer string=w1912:string)  [unwired: 1 in]
                n1114 = Concatenate Strings("set rate ", w1912, w1917) -> (w1910:string)
                n1115 = Number To Decimal String(number=w1903) -> (decimal integer string=w1908:string)  [unwired: 1 in]
                n1116 = Concatenate Strings("set volume ", w1908, w1917) -> (w1907:string)
              }
            }
          }
          event "Normal \nVolume (ul)": Value Change {
            n1117 = event-data() -> ()  [unwired: 1 in, 5 out]
            n1118 = call-poly "VISA Configure Serial Port"("VISA resource name"=w2002) -> ("VISA resource name out"=w2004:refnum<visa-resource-name>, "error out"=w2003:errorcluster)  [unwired: 13 in]
            n1119 = local read "Write Wait"() -> (w1987:i32)
            n1120 = Concatenate Strings("enter pump1", "\r") -> (w2006:string)
            n1121 = flat-sequence {
              tunnel: w2003 -> [w2016]
              tunnel: w2004 -> [w2018]
              tunnel: [w2017] -> w1996
              tunnel: [w2015] -> w1995
              tunnel: w2006 -> [w2014]
              tunnel: w1996 -> [w2021]
              tunnel: [w2021] -> w1994
              tunnel: w1995 -> [w2020]
              tunnel: [w2020] -> w1992
              tunnel: w1987 -> [w2019]
              tunnel: w1994 -> [w2025]
              tunnel: [w2026] -> w1993
              tunnel: w1992 -> [w2024]
              tunnel: [w2023] -> w1991
              tunnel: w1988 -> [w2022]
              tunnel: w1993 -> [w2029]
              tunnel: w1991 -> [w2028]
              tunnel: [w2029] -> w2013
              tunnel: [w2028] -> w2012
              tunnel: w1987 -> [w2027]
              tunnel: [w2034] -> w2011
              tunnel: [w2033] -> w2010
              tunnel: w2013 -> [w2032]
              tunnel: w2012 -> [w2031]
              tunnel: w1997 -> [w2030]
              tunnel: w2011 -> [w2037]
              tunnel: [w2037] -> w2009
              tunnel: w2010 -> [w2036]
              tunnel: [w2036] -> w2008
              tunnel: w1987 -> [w2035]
              tunnel: w2009 -> [w2041]
              tunnel: w2008 -> [w2040]
              frame #0 {
                n1122 = VISA Write(VISA resource name=w2018, write buffer=w2014, error in (no error)=w2016) -> (VISA resource name out=w2017:refnum<visa-resource-name>, error out=w2015:errorcluster)  [unwired: 1 out]
              }
              frame #1 {
                n1123 = Wait (ms)(milliseconds to wait=w2019) -> ()  [unwired: 1 out]
              }
              frame #2 {
                n1124 = VISA Write(VISA resource name=w2025, write buffer=w2022, error in (no error)=w2024) -> (VISA resource name out=w2026:refnum<visa-resource-name>, error out=w2023:errorcluster)  [unwired: 1 out]
              }
              frame #3 {
                n1125 = Wait (ms)(milliseconds to wait=w2027) -> ()  [unwired: 1 out]
              }
              frame #4 {
                n1126 = VISA Write(VISA resource name=w2032, write buffer=w2030, error in (no error)=w2031) -> (VISA resource name out=w2034:refnum<visa-resource-name>, error out=w2033:errorcluster)  [unwired: 1 out]
              }
              frame #5 {
                n1127 = Wait (ms)(milliseconds to wait=w2035) -> ()  [unwired: 1 out]
              }
              frame #6 {
                n1128 = Concatenate Strings("enter main ", "\r") -> (w2042:string)
                n1129 = VISA Write(VISA resource name=w2041, write buffer=w2042, error in (no error)=w2040) -> (VISA resource name out=w2039:refnum<visa-resource-name>, error out=w2038:errorcluster)  [unwired: 1 out]
                n1130 = VISA Close(VISA resource name=w2039, error in (no error)=w2038) -> ()  [unwired: 1 out]
              }
            }
            n1131 = Concatenate Strings("set units 4", "\r") -> (w1988:string)
            n1132 = Number To Decimal String(number="Normal \nVolume (ul)") -> (decimal integer string=w1999:string)  [unwired: 1 in]
            n1133 = Concatenate Strings("set volume", w1999, "\r") -> (w1997:string)
          }
          event "Normal \nRate (ul/hr)": Value Change {
            n1134 = event-data() -> ()  [unwired: 1 in, 5 out]
            n1135 = call-poly "VISA Configure Serial Port"("VISA resource name"=w2047) -> ("VISA resource name out"=w2055:refnum<visa-resource-name>, "error out"=w2054:errorcluster)  [unwired: 13 in]
            n1136 = local read "Write Wait"() -> (w2045:i32)
            n1137 = Concatenate Strings("enter pump1", "\r") -> (w2057:string)
            n1138 = flat-sequence {
              tunnel: w2054 -> [w2074]
              tunnel: w2055 -> [w2076]
              tunnel: [w2075] -> w2070
              tunnel: [w2073] -> w2069
              tunnel: w2057 -> [w2072]
              tunnel: w2070 -> [w2079]
              tunnel: [w2079] -> w2068
              tunnel: w2069 -> [w2078]
              tunnel: [w2078] -> w2067
              tunnel: w2045 -> [w2077]
              tunnel: w2068 -> [w2083]
              tunnel: [w2084] -> w2066
              tunnel: w2067 -> [w2082]
              tunnel: [w2081] -> w2065
              tunnel: w2048 -> [w2080]
              tunnel: w2066 -> [w2087]
              tunnel: w2065 -> [w2086]
              tunnel: [w2087] -> w2064
              tunnel: [w2086] -> w2063
              tunnel: w2045 -> [w2085]
              tunnel: [w2092] -> w2062
              tunnel: [w2091] -> w2061
              tunnel: w2064 -> [w2090]
              tunnel: w2063 -> [w2089]
              tunnel: w2051 -> [w2088]
              tunnel: w2062 -> [w2095]
              tunnel: [w2095] -> w2060
              tunnel: w2061 -> [w2094]
              tunnel: [w2094] -> w2059
              tunnel: w2045 -> [w2093]
              tunnel: w2060 -> [w2099]
              tunnel: w2059 -> [w2098]
              frame #0 {
                n1139 = VISA Write(VISA resource name=w2076, write buffer=w2072, error in (no error)=w2074) -> (VISA resource name out=w2075:refnum<visa-resource-name>, error out=w2073:errorcluster)  [unwired: 1 out]
              }
              frame #1 {
                n1140 = Wait (ms)(milliseconds to wait=w2077) -> ()  [unwired: 1 out]
              }
              frame #2 {
                n1141 = VISA Write(VISA resource name=w2083, write buffer=w2080, error in (no error)=w2082) -> (VISA resource name out=w2084:refnum<visa-resource-name>, error out=w2081:errorcluster)  [unwired: 1 out]
              }
              frame #3 {
                n1142 = Wait (ms)(milliseconds to wait=w2085) -> ()  [unwired: 1 out]
              }
              frame #4 {
                n1143 = VISA Write(VISA resource name=w2090, write buffer=w2088, error in (no error)=w2089) -> (VISA resource name out=w2092:refnum<visa-resource-name>, error out=w2091:errorcluster)  [unwired: 1 out]
              }
              frame #5 {
                n1144 = Wait (ms)(milliseconds to wait=w2093) -> ()  [unwired: 1 out]
              }
              frame #6 {
                n1145 = Concatenate Strings("enter main ", "\r") -> (w2100:string)
                n1146 = VISA Write(VISA resource name=w2099, write buffer=w2100, error in (no error)=w2098) -> (VISA resource name out=w2097:refnum<visa-resource-name>, error out=w2096:errorcluster)  [unwired: 1 out]
                n1147 = VISA Close(VISA resource name=w2097, error in (no error)=w2096) -> ()  [unwired: 1 out]
              }
            }
            n1148 = Concatenate Strings("set units 4", "\r") -> (w2048:string)
            n1149 = Number To Decimal String(number="Normal \nRate (ul/hr)") -> (decimal integer string=w2046:string)  [unwired: 1 in]
            n1150 = Concatenate Strings("set rate", w2046, "\r") -> (w2051:string)
          }
          event "Normal \nRate (ul/hr)  2": Value Change {
            n1151 = event-data() -> ()  [unwired: 1 in, 5 out]
            n1152 = call-poly "VISA Configure Serial Port"("VISA resource name"=w2105) -> ("VISA resource name out"=w2113:refnum<visa-resource-name>, "error out"=w2112:errorcluster)  [unwired: 13 in]
            n1153 = local read "Write Wait"() -> (w2103:i32)
            n1154 = Concatenate Strings("enter pump2", "\r") -> (w2115:string)
            n1155 = flat-sequence {
              tunnel: w2112 -> [w2132]
              tunnel: w2113 -> [w2134]
              tunnel: [w2133] -> w2128
              tunnel: [w2131] -> w2127
              tunnel: w2115 -> [w2130]
              tunnel: w2128 -> [w2137]
              tunnel: [w2137] -> w2126
              tunnel: w2127 -> [w2136]
              tunnel: [w2136] -> w2125
              tunnel: w2103 -> [w2135]
              tunnel: w2126 -> [w2141]
              tunnel: [w2142] -> w2124
              tunnel: w2125 -> [w2140]
              tunnel: [w2139] -> w2123
              tunnel: w2106 -> [w2138]
              tunnel: w2124 -> [w2145]
              tunnel: w2123 -> [w2144]
              tunnel: [w2145] -> w2122
              tunnel: [w2144] -> w2121
              tunnel: w2103 -> [w2143]
              tunnel: [w2150] -> w2120
              tunnel: [w2149] -> w2119
              tunnel: w2122 -> [w2148]
              tunnel: w2121 -> [w2147]
              tunnel: w2109 -> [w2146]
              tunnel: w2120 -> [w2153]
              tunnel: [w2153] -> w2118
              tunnel: w2119 -> [w2152]
              tunnel: [w2152] -> w2117
              tunnel: w2103 -> [w2151]
              tunnel: w2118 -> [w2157]
              tunnel: w2117 -> [w2156]
              frame #0 {
                n1156 = VISA Write(VISA resource name=w2134, write buffer=w2130, error in (no error)=w2132) -> (VISA resource name out=w2133:refnum<visa-resource-name>, error out=w2131:errorcluster)  [unwired: 1 out]
              }
              frame #1 {
                n1157 = Wait (ms)(milliseconds to wait=w2135) -> ()  [unwired: 1 out]
              }
              frame #2 {
                n1158 = VISA Write(VISA resource name=w2141, write buffer=w2138, error in (no error)=w2140) -> (VISA resource name out=w2142:refnum<visa-resource-name>, error out=w2139:errorcluster)  [unwired: 1 out]
              }
              frame #3 {
                n1159 = Wait (ms)(milliseconds to wait=w2143) -> ()  [unwired: 1 out]
              }
              frame #4 {
                n1160 = VISA Write(VISA resource name=w2148, write buffer=w2146, error in (no error)=w2147) -> (VISA resource name out=w2150:refnum<visa-resource-name>, error out=w2149:errorcluster)  [unwired: 1 out]
              }
              frame #5 {
                n1161 = Wait (ms)(milliseconds to wait=w2151) -> ()  [unwired: 1 out]
              }
              frame #6 {
                n1162 = Concatenate Strings("enter main ", "\r") -> (w2158:string)
                n1163 = VISA Write(VISA resource name=w2157, write buffer=w2158, error in (no error)=w2156) -> (VISA resource name out=w2155:refnum<visa-resource-name>, error out=w2154:errorcluster)  [unwired: 1 out]
                n1164 = VISA Close(VISA resource name=w2155, error in (no error)=w2154) -> ()  [unwired: 1 out]
              }
            }
            n1165 = Concatenate Strings("set units 4", "\r") -> (w2106:string)
            n1166 = Number To Decimal String(number="Normal \nRate (ul/hr)  2") -> (decimal integer string=w2104:string)  [unwired: 1 in]
            n1167 = Concatenate Strings("set rate", w2104, "\r") -> (w2109:string)
          }
          event "Normal \nVolume (ul) 2": Value Change {
            n1168 = event-data() -> ()  [unwired: 1 in, 5 out]
            n1169 = call-poly "VISA Configure Serial Port"("VISA resource name"=w2164) -> ("VISA resource name out"=w2168:refnum<visa-resource-name>, "error out"=w2169:errorcluster)  [unwired: 13 in]
            n1170 = local read "Write Wait"() -> (w2161:i32)
            n1171 = Concatenate Strings("enter pump2", "\r") -> (w2166:string)
            n1172 = flat-sequence {
              tunnel: w2169 -> [w2190]
              tunnel: w2168 -> [w2192]
              tunnel: [w2191] -> w2187
              tunnel: [w2189] -> w2186
              tunnel: w2166 -> [w2188]
              tunnel: w2187 -> [w2195]
              tunnel: [w2195] -> w2185
              tunnel: w2186 -> [w2194]
              tunnel: [w2194] -> w2184
              tunnel: w2161 -> [w2193]
              tunnel: w2185 -> [w2199]
              tunnel: [w2200] -> w2183
              tunnel: w2184 -> [w2198]
              tunnel: [w2197] -> w2182
              tunnel: w2175 -> [w2196]
              tunnel: w2183 -> [w2203]
              tunnel: w2182 -> [w2202]
              tunnel: [w2203] -> w2181
              tunnel: [w2202] -> w2180
              tunnel: w2161 -> [w2201]
              tunnel: [w2208] -> w2179
              tunnel: [w2207] -> w2178
              tunnel: w2181 -> [w2206]
              tunnel: w2180 -> [w2205]
              tunnel: w2172 -> [w2204]
              tunnel: w2179 -> [w2211]
              tunnel: [w2211] -> w2177
              tunnel: w2178 -> [w2210]
              tunnel: [w2210] -> w2176
              tunnel: w2161 -> [w2209]
              tunnel: w2177 -> [w2215]
              tunnel: w2176 -> [w2214]
              frame #0 {
                n1173 = VISA Write(VISA resource name=w2192, write buffer=w2188, error in (no error)=w2190) -> (VISA resource name out=w2191:refnum<visa-resource-name>, error out=w2189:errorcluster)  [unwired: 1 out]
              }
              frame #1 {
                n1174 = Wait (ms)(milliseconds to wait=w2193) -> ()  [unwired: 1 out]
              }
              frame #2 {
                n1175 = VISA Write(VISA resource name=w2199, write buffer=w2196, error in (no error)=w2198) -> (VISA resource name out=w2200:refnum<visa-resource-name>, error out=w2197:errorcluster)  [unwired: 1 out]
              }
              frame #3 {
                n1176 = Wait (ms)(milliseconds to wait=w2201) -> ()  [unwired: 1 out]
              }
              frame #4 {
                n1177 = VISA Write(VISA resource name=w2206, write buffer=w2204, error in (no error)=w2205) -> (VISA resource name out=w2208:refnum<visa-resource-name>, error out=w2207:errorcluster)  [unwired: 1 out]
              }
              frame #5 {
                n1178 = Wait (ms)(milliseconds to wait=w2209) -> ()  [unwired: 1 out]
              }
              frame #6 {
                n1179 = Concatenate Strings("enter main ", "\r") -> (w2216:string)
                n1180 = VISA Write(VISA resource name=w2215, write buffer=w2216, error in (no error)=w2214) -> (VISA resource name out=w2213:refnum<visa-resource-name>, error out=w2212:errorcluster)  [unwired: 1 out]
                n1181 = VISA Close(VISA resource name=w2213, error in (no error)=w2212) -> ()  [unwired: 1 out]
              }
            }
            n1182 = Concatenate Strings("set units 4", "\r") -> (w2175:string)
            n1183 = Number To Decimal String(number="Normal \nVolume (ul) 2") -> (decimal integer string=w2162:string)  [unwired: 1 in]
            n1184 = Concatenate Strings("set volume", w2162, "\r") -> (w2172:string)
          }
        }
        n1185 = node-c288() -> ()  [unwired: 1 in, 1 out]
      }
      n1186 = node-c288(w1548) -> ()  [unwired: 1 out]
    }
    frame Enabled {
      n1187 = node-c288(2 ("Processor")) -> (w2228:T12)  [unwired: 3 in]
      n1188 = timed-loop "Pump Control" {
        timing: w2228 -> [_]
        timing-out: [_] -> w2227
        tunnel: refnum<visa-resource-name> "COM5" ("VISA resource name") -> [w2230]
        stop <- w2229 stop-if-true
        n1189 = node-c288() -> ()  [unwired: 1 in, 1 out]
        n1190 = event shown="[3] \"Normal  Rate (ul/hr)  3\": Value Change" {
          selector: _ -> [_ _ _ _ _]
          dyn-events: _ -> [_ _ _ _ _]
          timeout: _ -> [_ _ _ _ _]
          tunnel: w2230 -> [w2236 _ w2310 w2337 w2342]
          tunnel: [_ w2308 _ _ _] -> w2229
          event "Flush Sample": Value Change {
            n1191 = event-data() -> ()  [unwired: 1 in, 5 out]
            n1192 = local read "Write Wait"() -> (w2250:i32)
            n1193 = flat-sequence {
              tunnel: [w2274] -> w2270
              tunnel: [w2273] -> w2269
              tunnel: "CLD" -> [w2272]
              tunnel: w2236 -> [w2271]
              tunnel: w2270 -> [w2277]
              tunnel: [w2277] -> w2268
              tunnel: w2269 -> [w2276]
              tunnel: [w2276] -> w2267
              tunnel: w2250 -> [w2275]
              tunnel: [w2282] -> w2266
              tunnel: [w2279] -> w2265
              tunnel: w2268 -> [w2281]
              tunnel: w2267 -> [w2280]
              tunnel: "MODVOL" -> [w2278]
              tunnel: w2266 -> [w2285]
              tunnel: [w2285] -> w2264
              tunnel: [w2284] -> w2263
              tunnel: w2265 -> [w2284]
              tunnel: w2250 -> [w2283]
              tunnel: w2264 -> [w2290]
              tunnel: [w2289] -> w2262
              tunnel: w2252 -> [w2288]
              tunnel: w2263 -> [w2287]
              tunnel: [w2286] -> w2261
              tunnel: w2262 -> [w2293]
              tunnel: [w2293] -> w2260
              tunnel: [w2292] -> w2259
              tunnel: w2261 -> [w2292]
              tunnel: w2250 -> [w2291]
              tunnel: w2260 -> [w2298]
              tunnel: [w2297] -> w2258
              tunnel: w2254 -> [w2296]
              tunnel: w2259 -> [w2295]
              tunnel: [w2294] -> w2257
              tunnel: [w2301] -> w2255
              tunnel: w2258 -> [w2301]
              tunnel: [w2300] -> w2256
              tunnel: w2257 -> [w2300]
              tunnel: w2250 -> [w2299]
              tunnel: w2256 -> [w2306]
              tunnel: w2255 -> [w2307]
              tunnel: [w2305] -> w2245
              tunnel: "RUN " -> [w2304]
              frame #0 {
                n1194 = call "Write to pump 2.vi"("String to write"=w2272, "VISA resource name"=w2271) -> ("error out"=w2273:errorcluster, "VISA resource name out"=w2274:refnum<visa-resource-name>)  [unwired: 8 in]
              }
              frame #1 {
                n1195 = Wait (ms)(milliseconds to wait=w2275) -> ()  [unwired: 1 out]
              }
              frame #2 {
                n1196 = call "Write to pump 2.vi"("error in (no error)"=w2280, "String to write"=w2278, "VISA resource name"=w2281) -> ("error out"=w2279:errorcluster, "VISA resource name out"=w2282:refnum<visa-resource-name>)  [unwired: 7 in]
              }
              frame #3 {
                n1197 = Wait (ms)(milliseconds to wait=w2283) -> ()  [unwired: 1 out]
              }
              frame #4 {
                n1198 = call "Write to pump 2.vi"("error in (no error)"=w2287, "String to write"=w2288, "VISA resource name"=w2290) -> ("error out"=w2286:errorcluster, "VISA resource name out"=w2289:refnum<visa-resource-name>)  [unwired: 7 in]
              }
              frame #5 {
                n1199 = Wait (ms)(milliseconds to wait=w2291) -> ()  [unwired: 1 out]
              }
              frame #6 {
                n1200 = call "Write to pump 2.vi"("error in (no error)"=w2295, "String to write"=w2296, "VISA resource name"=w2298) -> ("error out"=w2294:errorcluster, "VISA resource name out"=w2297:refnum<visa-resource-name>)  [unwired: 7 in]
              }
              frame #7 {
                n1201 = Wait (ms)(milliseconds to wait=w2299) -> ()  [unwired: 1 out]
              }
              frame #8 {
                w2303 = TRUE ("Inject Pump 3")
                n1202 = Tick Count (ms)() -> (millisecond timer value=→"Flush Sample Start Time":u32)
                n1203 = call "Write to pump 2.vi"("error in (no error)"=w2306, "String to write"=w2304, "VISA resource name"=w2307) -> ("error out"=w2305:errorcluster)  [unwired: 7 in, 1 out]
                n1204 = local write "Inject Sample"(w2303) -> ()
                "Flushing Sample" <- w2303
              }
            }
            n1205 = Number To Fractional String(number="Flush \nRate (ul/min)  3") -> (F-format string=w2238:string)  [unwired: 3 in]
            n1206 = String Subset(string=w2238, length (rest)=6 ("length (rest)")) -> (substring=w2237:string)  [unwired: 1 in]
            n1207 = Concatenate Strings("RAT", w2237, "UM") -> (w2252:string)
            n1208 = Divide(x="Flush\nVolume (ul)  3", y=1000.0) -> (x/y=w2243:dbl)
            n1209 = Number To Fractional String(number=w2243) -> (F-format string=w2242:string)  [unwired: 3 in]
            n1210 = Divide(x="Flush\nVolume (ul)  3", y="Flush \nRate (ul/min)  3") -> (x/y=w2233:dbl)
            n1211 = Multiply(x=w2233, y=60.0) -> (x*y=→"Sample flush time (s)":dbl)
            n1212 = String Subset(string=w2242, length (rest)=6 ("length (rest)")) -> (substring=w2241:string)  [unwired: 1 in]
            n1213 = Concatenate Strings("TGT", w2241) -> (w2254:string)
            "error out" <- w2245
          }
          event "Stop": Value Change {
            n1214 = event-data() -> ()  [unwired: 1 in, 5 out]
            n1215 = local read "Stop"() -> (w2308:bool)
          }
          event "Inject Sample": Value Change {
            n1216 = event-data() -> ()  [unwired: 1 in, 5 out]
            n1217 = case shown="True" "Inject Sample" {
              tunnel: w2310 -> [w2312 w2313]
              frame False {
                n1218 = call "Write to pump 2.vi"("String to write"="STP", "VISA resource name"=w2312) -> ()  [unwired: 8 in, 2 out]
              }
              frame True {
                n1219 = local read "Normal \nRate (ul/hr)  3"() -> (w2314:dbl)
                n1220 = Number To Fractional String(number=w2314) -> (F-format string=w2317:string)  [unwired: 3 in]
                n1221 = String Subset(string=w2317, length (rest)=6 ("length (rest)")) -> (substring=w2315:string)  [unwired: 1 in]
                n1222 = flat-sequence {
                  tunnel: "RUN " -> [w2329]
                  tunnel: [w2331] -> _
                  tunnel: [w2330] -> _
                  tunnel: w2313 -> [w2328]
                  frame #0 {
                    n1223 = call "Write to pump 2.vi"("String to write"=w2329, "VISA resource name"=w2328) -> ("error out"=w2330:errorcluster, "VISA resource name out"=w2331:refnum<visa-resource-name>)  [unwired: 8 in]
                  }
                }
                n1224 = Concatenate Strings("RAT", w2315, "UH" ("string")) -> ()  [unwired: 1 out]
                n1225 = local read "Normal \nVolume (ul) 3"() -> (w2323:dbl)
                n1226 = Divide(x=w2323, y=1000.0) -> (x/y=w2318:dbl)
                n1227 = Number To Fractional String(number=w2318) -> (F-format string=w2321:string)  [unwired: 3 in]
                n1228 = String Subset(string=w2321, length (rest)=6 ("length (rest)")) -> (substring=w2319:string)  [unwired: 1 in]
                n1229 = Concatenate Strings("TGT", w2319) -> ()  [unwired: 1 out]
              }
            }
          }
          event "Normal \nRate (ul/hr)  3": Value Change {
            n1230 = event-data() -> ()  [unwired: 1 in, 5 out]
            n1231 = Number To Fractional String(number="Normal \nRate (ul/hr)  3") -> (F-format string=w2335:string)  [unwired: 3 in]
            n1232 = String Subset(string=w2335, length (rest)=6 ("length (rest)")) -> (substring=w2333:string)  [unwired: 1 in]
            n1233 = Concatenate Strings("RAT", w2333, "UH") -> (w2336:string)
            n1234 = call "Write to pump 2.vi"("String to write"=w2336, "VISA resource name"=w2337) -> ()  [unwired: 8 in, 2 out]
          }
          event "Clear Volume": Value Change {
            n1235 = event-data() -> ()  [unwired: 1 in, 5 out]
            n1236 = Divide(x="Normal \nVolume (ul) 3", y=1000.0) -> (x/y=w2355:dbl)
            n1237 = Number To Fractional String(number=w2355) -> (F-format string=w2358:string)  [unwired: 3 in]
            n1238 = String Subset(string=w2358, length (rest)=6 ("length (rest)")) -> (substring=w2356:string)  [unwired: 1 in]
            n1239 = flat-sequence {
              tunnel: [w2365] -> w2353
              tunnel: [w2364] -> w2352
              tunnel: w2342 -> [w2363]
              tunnel: w2341 -> [w2362]
              tunnel: [w2367] -> w2350
              tunnel: [w2366] -> w2351
              tunnel: w2347 -> [w2368]
              tunnel: w2353 -> [w2367]
              tunnel: w2352 -> [w2366]
              tunnel: w2351 -> [w2372]
              tunnel: w2350 -> [w2373]
              tunnel: [w2371] -> _
              tunnel: [w2370] -> _
              tunnel: w2340 -> [w2369]
              frame #0 {
                n1240 = call "Write to pump 2.vi"("String to write"=w2362, "VISA resource name"=w2363) -> ("error out"=w2364:errorcluster, "VISA resource name out"=w2365:refnum<visa-resource-name>)  [unwired: 8 in]
              }
              frame #1 {
                n1241 = Wait (ms)(milliseconds to wait=w2368) -> ()  [unwired: 1 out]
              }
              frame #2 {
                n1242 = call "Write to pump 2.vi"("error in (no error)"=w2372, "String to write"=w2369, "VISA resource name"=w2373) -> ("error out"=w2370:errorcluster, "VISA resource name out"=w2371:refnum<visa-resource-name>)  [unwired: 7 in]
              }
            }
            n1243 = local read "Write Wait"() -> (w2347:i32)
            n1244 = Concatenate Strings("TGT", w2356) -> (w2341:string)
            n1245 = local read "Normal \nRate (ul/hr)  3"() -> (w2343:dbl)
            n1246 = local write "Clear Volume"(FALSE ("Clear Volume")) -> ()
            n1247 = Number To Fractional String(number=w2343) -> (F-format string=w2346:string)  [unwired: 3 in]
            n1248 = String Subset(string=w2346, length (rest)=6 ("length (rest)")) -> (substring=w2344:string)  [unwired: 1 in]
            n1249 = Concatenate Strings("RAT", w2344, "UH" ("string")) -> (w2340:string)
          }
        }
        n1250 = node-c288() -> ()  [unwired: 1 in, 1 out]
      }
      n1251 = node-c288(w2227) -> ()  [unwired: 1 out]
    }
  }
  n1252 = node-c288() -> (w84:T12)  [unwired: 4 in]
  n1253 = timed-loop {
    timing: w84 -> [_]
    timing-out: [_] -> w83
    stop <- w2380 stop-if-true
    n1254 = node-c288() -> ()  [unwired: 1 in, 1 out]
    n1255 = event shown="[1] \"Stop\": Value Change" {
      selector: _ -> [_ _]
      dyn-events: _ -> [_ _]
      timeout: _ -> [_ _]
      tunnel: [_ "Stop"] -> w2380
      event Timeout {
        n1256 = event-data() -> ()  [unwired: 1 in, 2 out]
      }
      event "Stop": Value Change {
        n1257 = event-data() -> ()  [unwired: 1 in, 4 out]
        n1258 = local write "Force Feedback"(FALSE ("Force Feedback")) -> ()
      }
    }
    n1259 = node-c288() -> ()  [unwired: 1 in, 1 out]
  }
  n1260 = case shown="True" w73 {
    tunnel: w78 -> [_ w2387]
    tunnel: w77 -> [_ w2386]
    tunnel: w76 -> [_ w2385]
    frame False {
    }
    frame True {
      w2389 = T15 3 items=["no dialog", "OK message", "continue or stop message", "OK message + warnings", "continue/stop + warnings"] ("type of dialog (OK msg:1)")
      w2388 = T15 3 items=["no dialog", "OK message", "continue or stop message", "OK message + warnings", "continue/stop + warnings"] ("type of dialog (OK msg:1)")
      n1261 = call <vilib>:"DAQmx Clear Task.vi"("task in"=w2387, "error in"=w2385) -> ("error out"=w2390:errorcluster)  [unwired: 13 in]
      n1262 = call <vilib>:"DAQmx Clear Task.vi"("task in"=w2386) -> ("error out"=w2391:errorcluster)  [unwired: 14 in]
      n1263 = call <vilib>:"Simple Error Handler.vi"("type of dialog (OK msg:1)"=w2389, "error in (no error)"=w2390) -> ()  [unwired: 3 in, 5 out]
      n1264 = call <vilib>:"Simple Error Handler.vi"("type of dialog (OK msg:1)"=w2388, "error in (no error)"=w2391) -> ()  [unwired: 3 in, 5 out]
    }
  }
  n1265 = case shown="\"Force Feedback\", Default" "?" {
    frame "Force Feedback", Default {
    }
    frame "Raster scan" {
    }
  }
  n1266 = node-c288(w83) -> ()  [unwired: 1 out]
  n1267 = node-c288(w86) -> ()  [unwired: 1 out]
  n1268 = local write "Pause Mouse/Mirror Connection"(FALSE ("Pause Mouse/Mirror Connection")) -> ()
  n1269 = local write "Stop"(FALSE ("Stop all")) -> ()
  "CoordinatesMousePressed" <- T4 {"Horizontal"=0, "Vertical"=0} ("Coords when pressed")
  "Deflection" <- T4 {"Horizontal"=0, "Vertical"=0} ("Coords when pressed")
